vi "Arch_screen_patch_v2.0.vi"() -> ()   [LabVIEW 2012]
uses:
  <vilib>/DAQmx/write.llb/DAQmx Write (Analog DBL 1Chan 1Samp).vi
  <vilib>/DAQmx/create/channels.llb/DAQmx Create Channel (AO-Voltage-Basic).vi
  <vilib>/DAQmx/miscellaneous.llb/DAQmx Fill In Error Info.vi
panel:
  out "ROI cursor":T1={"x offset"=480, "y offset"=456, "x width"=68, "y width"=76} {"x offset" min=1 max=512 step=1; "y offset" min=1 max=512 step=1; "x width" min=1 max=512 step=1; "y width" min=1 max=512 step=1}
  out "Abs V camera":digitalwaveform(waveform)={"t0"=timestamp(0 s since 1904-01-01), "dt"=0.0, "Y"={"transitions"=[], "data"=[]}, "error"={"status"=FALSE, "code"=37421928, "source"=""}}
  out "Abs V lasers":digitalwaveform[](array[waveform])
  out "Abs V DO":digitalwaveform[](array[waveform])
  out "Abs V AO":waveform(dbl)
  out "laser boolean array abs V":bool[](array[boolean])
  out "Previous Bin":u16(ring)=2 caption="Cursor Bin" items=["1x1"=1, "2x2"=2, "4x4"=4]
  in  "Tab":T2(tab)=enum."Acquire"
  in  "Camera trigger":tag="Dev1/port0/line0"
  in  "AOTF info":T3={"AOTF calibration curve path"=path "C:/Peng/LabVIEW codes/Arch_screen_NW348/2013-04-27_AOTF_efficiency", "VISA resource name"="COM8"}
  out "Waveform generated":bool
  in  "Load Mem_AbsV waveform":bool
  in  "Cam frame rate (Hz)\nAbs V":dbl=200.0 format="%0.2p"
  out "# cam. \nframes AbsV":u32=50000
  out "Tot time \nAbs V (s)":dbl=50000.0
  out "# cam. \nframes Mem":u32=50000
  out "Tot time \nMem (s)":dbl=50000.0
  in  "Cam frame rate (Hz)\nMem":dbl=200.0 format="%0.2p"
  out "sample num AbsV":i32
  out "Sample num mem":i32
  out "Model":string="-"
  out "Initialize?":bool
  out "y pixels":i32
  out "x pixels":i32
  out "Bits per Channel":i32
  out "Camera ID":string="-"
  in  "Abs V Waveform txt file":path=path "C:/Peng/LabVIEW codes/Arch_screen_NW348/waveforms/03_waveforms.txt"
  in  "Memory Waveform txt file":path=path "C:/Peng/LabVIEW codes/Arch_screen_NW348/waveforms/03_waveforms.txt"
  in  "stop program":bool
  in  "External":dbl(ring)=10.0 caption="Cursor Bin" items=["div10"=10.0, "div50"=50.0]
  in  "Probe Gain":bool caption="Cursor Bin"
  in  "Gain":dbl(knob)=10.0 scale=1.0..100.0
  in  "Shutter lines":T4={"shutter 640nm"="Dev1/port0/line2", "shutter 594nm"="Dev1/port0/line3", "shutter 561nm"="Dev1/port0/line4", "shutter 532nm"="Dev1/port0/line5", "shutter 488nm"="Dev1/port0/line6", "shutter Dragon"="Dev1/port0/line7", "shutter Global"="Dev1/port0/line13"}
  in  "AOTF digital lines":T5={"AOTF 640nm"="Dev1/port0/line8", "AOTF 594nm"="Dev1/port0/line9", "AOTF 561nm"="Dev1/port0/line10", "AOTF 532nm"="Dev1/port0/line11", "AOTF 488nm"="Dev1/port0/line12", "AOTF weak 488nm"="Dev1/port0/line14"}
  in  "AI ports":T6={"AI scaled output"="Dev1/ai0", "AI V_m"="Dev1/ai1", "photodiode"="Dev1/ai2"}
  in  "AO ports":T7={"AO A-M External"="Dev1/ao0", "White LED"="Dev1/ao1", "447nm laser"="Dev1/ao2"}
  in  "DAQ sampling rate":dbl=10000.0 format="%0.0f"
  in  "DI camera fire":tag="Dev1/port0/line1"
  in  "Simultaneous":bool
  out "# output\nsamples L":u32=12500
  out "Laser Pump Waveform":waveform(dbl)[](graph)=[{"t0"=timestamp(0 s since 1904-01-01), "dt"=0.0001, "Y"=array[12500 elements]}, {"t0"=timestamp(0 s since 1904-01-01), "dt"=0.0001, "Y"=array[12500 elements]}]
  out "Square Waveform":waveform(dbl)[](graph)=[{"t0"=timestamp(0 s since 1904-01-01), "dt"=0.0001, "Y"=array[60000 elements]}, {"t0"=timestamp(0 s since 1904-01-01), "dt"=0.0001, "Y"=array[60000 elements]}]
  out "Triangle Waveform":waveform(dbl)[](graph)=[{"t0"=timestamp(0 s since 1904-01-01), "dt"=0.0001, "Y"=array[120000 elements]}, {"t0"=timestamp(0 s since 1904-01-01), "dt"=0.0001, "Y"=array[120000 elements]}]
  out "memory camera":digitalwaveform(waveform)={"t0"=timestamp(0 s since 1904-01-01), "dt"=0.0, "Y"={"transitions"=[], "data"=[]}, "error"={"status"=FALSE, "code"=37421928, "source"=""}}
  out "Memory DO":digitalwaveform[](array[waveform])
  out "Memory AO":waveform(dbl)
  out "Memory lasers":digitalwaveform[](array[waveform])
  out "laser boolean array memory":bool[](array[boolean])
  in  "Lasers to use":bool[](array[boolean])=[TRUE, FALSE, FALSE, FALSE, FALSE]
  in  "Square setting":T8={"Baseline Sq (mV)"=-70.0, "Stepsize Sq (mV)"=100.0, "Duty cycle (%)"=50.0, "Voltage freq. (Hz)"=5.0, "# cycles per color"=30, "Frame rate (Hz)"=1000.0, "# spect. cycles"=1, "Clamp mode"=FALSE, "Baseline Sq (pA)"=0.0, "Stepsize Sq (pA)"=500.0} caption="Square wave settings" {"Stepsize Sq (pA)" format="%0.2p"; "Baseline Sq (pA)" format="%0.2p"; "Frame rate (Hz)" format="%0.0f"; "Voltage freq. (Hz)" format="%0.2p"; "Duty cycle (%)" format="%0.2f"; "Stepsize Sq (mV)" format="%0.2p"; "Baseline Sq (mV)" format="%0.2p"}
  out "Square info":cluster{"# frames":u32, "# output\nsamples":u32}={"# frames"=6000, "# output\nsamples"=60000}
  in  "Triangle setting":T9={"# cycles per color"=3, "Voltage freq. (Hz)"=0.1, "Amplitude Tri (V)"=0.1, "# spect. cycles"=1, "Frame rate (Hz)"=10.0} caption="Triangle wave settings" {"Frame rate (Hz)" format="%0.2p"; "Amplitude Tri (V)" format="%0.2p"; "Voltage freq. (Hz)" format="%0.3f"}
  out "Triangle info":T10={"# frames"=120, "# output\nsamples"=120000, "voltage slope\n(mV/sec)"=100.0}
  in  "Pump setting":T11={"Duty cycle (%)"=50.0, "# spect. cycles"=1, "# cycles per color"=5, "Laser freq. (Hz)"=4.0, "Holding (mV)"=-70.0} caption="Laser pump settings" {"Holding (mV)" format="%0.2p"; "Laser freq. (Hz)" format="%0.2p"; "Duty cycle (%)" format="%0.2f"}
  out "Elapsed time (sec)":dbl=100.0 min=1.0 max=5000.0 step=1.0
  in  "Total time (sec)":dbl=100.0 min=1.0 max=5000.0 step=1.0
  in  "# frames":u32=100 min=1 max=5000 step=1
  in  "Acquire movie":bool
  in  "447 signal":dbl=2.5 caption="447 signal (0-5V)"
  in  "Shutters":bool[](array[boolean])=[FALSE, FALSE, FALSE, FALSE, FALSE, FALSE, FALSE]
  out "laser bool array":bool[](array[boolean])=[TRUE, FALSE, FALSE, FALSE, FALSE] caption="Waveform"
  in  "AOTF efficiency":dbl[](array[numeric])=[1.0, 0.25363829, 0.20220272, 0.020387013, 0.10018123, 0.010868696] caption="AOTF\nefficiency"
  out "simultaneous ind":bool caption="Simultaneous?"
  in  "Dichroic":u16(ring)=2 caption="Cursor Bin" items=["510/20, 640LP"=1, "ZT532/640rpc"=2]
  in  "Emission filter":u16(ring)=3 items=["600/37"=1, "ET575/50"=2, "708/75"=3, "620LP"=4, "ET590/50M"=5, "HQ660LP"=6, "525/30"=7]
  in  "apply dualview":bool
  in  "apply const power":bool
  in  "apply const fluor":bool
  in  "Const fluor.":u16[](array[numeric])=[595, 455, 150, 360, 150, 150]
  in  "Const power":u16[](array[numeric])=[248, 455, 132, 266, 475, 475]
  in  "DualView":u16[](array[numeric])=[1023, 760, 260, 800, 10, 10]
  in  "AOTF amplitude":u16[](array[numeric])=[604, 144, 112, 51, 71, 24] caption="AOTF\namplitude"
  in  "White LED":bool
  out "file size (MB)":dbl[](array[numeric])=[242.25, 4.845]
  out "cam frame\nrate (Hz)":dbl[](array[numeric])=[1000.0, 10.0]
  out "# cam\nframes":i32[](array[numeric])=[6000, 120]
  in  "Previous ROI":bool
  out "Previous ROI":T1={"x offset"=256, "y offset"=256, "x width"=512, "y width"=512} caption="Previous" {"x offset" min=1 max=512 step=1; "y offset" min=1 max=512 step=1; "x width" min=1 max=512 step=1; "y width" min=1 max=512 step=1}
  out "Location indicator":u16[][](graph)
  out "Waveform Graph":cluster{"xo":i32, dbl, "data":dbl[][]}(graph)={"xo"=0, 0.0001, "data"=array3x120000[360000 elements]}
  in  "appended folder name":string
  out "Status":string="Ready"
  in  "SAVE":bool=TRUE
  in  "Start acquisition":bool
  in  "Exposure (msec)":dbl=100.0 min=1.0 max=5000.0 step=1.0
  in  "Live":bool
  in  "Update ROI":bool
  out "ROI":T1={"x offset"=960, "y offset"=912, "x width"=136, "y width"=152} caption="Current" {"x offset" min=1 max=512 step=1; "y offset" min=1 max=512 step=1; "x width" min=1 max=512 step=1; "y width" min=1 max=512 step=1}
  in  "base path":path=path "C:/Peng/Data"
  in  "Notes":string
  out "Image":u16[][](graph)
  out "Error":errorcluster
  out "full path":path=path "C:/Peng/Data/2013-10-16 patch ssFRET rainbow/PZ083 Arch3.77Q-YFP/fov2/20131016at2350_ST_take1 640"
  in  "Snap&Save":bool
  in  "Bin (n x n)":u16(ring)=1 caption="Cursor Bin" items=["1x1"=1, "2x2"=2, "4x4"=4]
  in  "Camera mode":u16(ring) items=["Focus", "Square wave", "Triangle wave", "Memory", "Absolute Voltage"]
  in  "Symmetrical":bool=TRUE
  in  "Define ROI":bool
  out "max frame rate (Hz)":dbl
  in  "ROI selection":u16(ring)=2 items=["Full ROI", "Central quad", "Custom ROI"]
  in  "Measurements":T12={"Square wave"=TRUE, "Triangle wave"=TRUE, "Laser pump"=FALSE, "Memory"=FALSE, "Absolute Voltage"=FALSE}
  in  "White Light\nCurrent (mA)":dbl=100.0
  in  "AOTF\ndigital":bool[](array[boolean])=[FALSE, FALSE, FALSE, FALSE, FALSE, FALSE]
  in  "447nm":bool
  in  "AOTF channels":string[](array[string])=["640nm", "594nm", "561nm", "532nm", "488nm", "488 weak", ""] caption="AOTF\nchannels"
  out "Image info":T13={"max value"=189, "mean"=115, "min value"=72, "Histogram"={"X Values"=[72.585, 73.755, 74.925, 76.095, 77.265, 78.435, 79.605, 80.775, 81.945, 83.115, 84.285, 85.455, 86.625, 87.795, 88.965, 90.135, 91.305, 92.475, 93.645, 94.815, 95.985, 97.155, 98.325, 99.495, 100.665, 101.835, 103.005, 104.175, 105.345, 106.515, 107.685, 108.855, 110.025, 111.195, 112.365, 113.535, 114.705, 115.875, 117.045, 118.215, 119.385, 120.555, 121.725, 122.895, 124.065, 125.235, 126.405, 127.575, 128.745, 129.915, 131.085, 132.255, 133.425, 134.595, 135.765, 136.935, 138.105, 139.275, 140.445, 141.615, 142.785, 143.955, 145.125, 146.295, 147.465, 148.635, 149.805, 150.975, 152.145, 153.315, 154.485, 155.655, 156.825, 157.995, 159.165, 160.335, 161.505, 162.675, 163.845, 165.015, 166.185, 167.355, 168.525, 169.695, 170.865, 172.035, 173.205, 174.375, 175.545, 176.715, 177.885, 179.055, 180.225, 181.395, 182.565, 183.735, 184.905, 186.075, 187.245, 188.415], "Histogram: h(x)"=[1, 0, 0, 0, 0, 0, 0, 0, 0, 0, 0, 0, 1, 0, 2, 0, 0, 3, 1, 2, 8, 6, 23, 82, 113, 84, 265, 249, 411, 1102, 818, 853, 1028, 1082, 1261, 2548, 1184, 1231, 1256, 891, 1045, 1706, 613, 540, 482, 408, 303, 447, 154, 112, 91, 74, 87, 22, 18, 13, 13, 11, 9, 8, 1, 3, 1, 1, 1, 0, 0, 2, 0, 0, 0, 0, 1, 0, 0, 0, 0, 0, 0, 0, 0, 0, 0, 0, 0, 0, 0, 0, 0, 0, 0, 0, 0, 0, 0, 0, 0, 0, 0, 1]}}
  out "Frames Recorded":i32
  in  "Movie name":string
  out "Patch quality":T14={"Ra (Mohm)"=16.150195020321526, "Rm (Mohm)"=1531.699142639844, "Cm (pF)"=12.467883400052433}
  out "Average I-t curve":cluster{"xo":i32, dbl, dbl[]}(graph)={"xo"=0, 5e-05, [2.8707122065427546, 28.25943561367525, 495.34938130700425, 622.4519180333322, 425.26771536879573, 278.1195833345387, 189.11750895359194, 128.51335365854402, 88.53469124393202, 62.11882679632106, 45.13719962647474, 31.418606844285872, 23.429798545455782, 18.90309568623423, 14.687982318872775, 12.446269046932088, 10.239176831097117, 8.34849917972882, 7.35697405512405, 7.089655767322204, 6.89441489534627, 5.943330783548681, 5.999092552412099, 5.674022726333197, 5.807681868962271, 5.388399026472767, 4.8008359874823965, 5.397054290640863, 5.795196415013253, 5.6037857312452894, 3.6420255502292136, 4.2449093465586785, 4.462285821390441, 4.81232655490619, 4.06314881117431, 4.023702683502782, 4.856597758823761, 5.0643240833158805, 3.890043539987264, 4.402693860851977, 3.6188950637578388, 3.8093108632431627, 4.008381925697188, 3.6092449159742417, 4.208447872227028, 3.5275173543206915, 3.7487240188077378, 4.950810771116034, 4.170842165203316, 3.513042131492717, 4.365088153558202, 4.212128714503955, 3.897703919213018, 4.150696331711198, 3.6774921383958934, 3.478421076610598, 3.5812893553166996, 4.423685227161449, 4.491086914876741, 3.9399853523124615, 3.5245326999555786, 3.8015011340435922, 4.4737763887167485, 3.771705153758482, 3.5033919835424494, 3.688982707357445, 3.5072221719058696, 4.210138942235079, 4.480441882017596, 4.22560904889491, 4.265055177230385, 3.4706113488645483, 4.503423019449819, 4.148557213549512, 3.2147836308660427, 4.159202246520172, 3.6495365784348035, 4.560179676020346, 3.9188446343850734, 3.726439066639748, 3.813986586682297, 3.8717381274540426, 3.962120952275759, 3.611085335331802, 3.2735300559554843, 3.6774921393547224, 3.0860989116048767, 3.0957490597233615, 2.9091634491428553, 3.8179661263568017, 2.9687554116458377, 2.950599347172765, 3.1438504516499965, 2.9419440835611486, 3.116044240320801, 3.9556048097735528, 3.793144570341247, 4.41532866466503, 3.820950782063075, 3.8940230795432553, 4.243068928043317, 5.0057270088990995, 4.145025723437888, 4.121049701768749, 4.235408549596437, 3.484241037148812, 3.047647666451965, 3.167826472926228, 2.7938097180689163, 2.6696513744839825, 3.478421077597534, 3.52070251050323, 3.040832823259014, 3.772700038745409, 3.4802614973361625, 4.136221108929308, 3.518712740842017, 3.8967090322741544, 3.8822338110762447, 3.6580424951603736, 4.364938802393973, 4.243765113064731, 4.017733374522697, 5.402575546268753, 4.085135062157726, 4.03220859674942, 3.940830887980181, 4.681353364917516, 3.958141414588577, 3.436985179664323, 3.484091687209613, 3.9937573539364206, 3.3561031534289367, 4.123586307280213, 3.295516308920549, 3.1879723046440365, 3.183147229597545, 3.0042220007778875, 3.5649737132920962, 3.5688039024557785, 3.5504984908457278, 3.1476806401485162, 2.7408832516409616, 2.666816069009991, 2.896677996222178, 3.254528457670239, 3.812295516696531, 3.6208848342587534, 3.091918870269982, 3.752554208494307, 3.347746588573524, 3.1832965805156896, 3.4141533914677353, 3.238063467210657, 3.737233449313549, 3.665156035932181, 2.9043383758197265, 3.847762108077382, 3.295815006546575, 2.8707122061701376, 2.9196591347766976, 2.8918529229379635, 2.763018853441849, 3.248708499972387, 3.147680641571172, 3.753549092093494, 2.93512924113729, 3.1947871478342127, 3.0927644059598642, 3.065803729594899, 3.4484757489316546, 2.8580774051196585, 3.3407823961033065, 3.610090451051438, 3.1666822395681997, 3.8293073449580333, 3.5466683010591322, 2.7725196519836453, 3.63605624228866, 3.151361482411702, 2.771524768119689, 2.86290247786551, 3.5841246596346896, 3.5985998808722592, 3.8351273041809937, 3.628395862475988, 3.1811574620103262, 3.5283628884880756, 3.125395690871513, 3.6274009786868104, 3.5688039016658197, 2.986911473213223, 2.687807437324858, 3.0263576018969873, 3.394703746055811, 3.17449196711015, 3.210107905674445, 3.503391983506148, 3.298500962686518, 3.35426273396358, 2.4937107964587506, 2.899513300969879, 3.0975894787488385, 2.900358837483566, 3.1696668929879364, 3.9274998985711203, 2.991736548293083, 3.528362889331557, 3.269699866124547, 2.8975235321834654, 2.96676564182466, 2.7763498429642675, 3.0686390350921897, 2.911998753926087, 2.7340684091349785, 2.843751530540078, 2.5003762927589874, 3.188967190353448, 3.9468001942839486, 3.1024145537142283, 2.3350807478640707, 2.848576604166416, 3.5160267863942365, 3.121714850915303, 3.171656662784131, 3.0543131617334405, 2.9341343563008473, 2.7024320079126802, 2.4937107978816617, 2.802464981799372, 3.054462510324043, 3.6506808143167673, 2.947764042002109, 2.8668820164989324, 2.5677779799164897, 2.962089916122025, 3.184291464550388, 2.8572318690848606, 3.837266423481291, 2.8736968594072883, 2.4024824360153496, 3.03814686754593, 3.977740410645141, 3.0775929965325073, 3.207421950221236, 3.315115302978166, 3.31511530295825, 3.8286111597263828, 2.863051827098326, 3.188121654027938, 3.123704619874777, 3.7631992403071175, 3.669831761129438, 2.971590715530302, 3.169816241769228, 3.0621228891125574, 3.0062117702383317, 2.723423377103205, 3.5082170572886073, 3.4687709286069697, 2.8196261602637356, 3.13987091299179, 3.3292918268546083, 2.716757881605072, 1.9935459302372251, 2.463765469786085, 3.3590878088139546, 3.911184257035688, 3.7332539110731227, 2.797639907149591, 3.3246161026796726, 3.4938911844625085, 3.4015185907484784, 3.354412083213049, 3.7092778896912812, 3.3544120829400885, 3.366052000028813, 3.3276007561109537, 2.623539752408288, 3.16698093704695, 2.997705855446494, 3.1371849570223636, 3.7412129879546265, 4.116224628425303, 4.409508707303248, 3.9797301797364373, 3.460414363687271, 3.7363879143265177, 4.414333780436046, 3.944114240479511, 4.273014257618848, 4.416323549705721, 4.187456505855945, 4.628874948847732, 4.683641836040581, 3.7478784833258767, 3.4382787628796616, 3.8152801710309263, 3.6613258471654078, 3.6806261429867977, 3.3469010526306815, 3.0198414573901218, 2.993875665257011, 3.321780796754825, 2.9870608222374897, 3.0746083430207944, 2.91781871363435, 3.084258491383432, 2.89185292323233, 3.1563359041780004, 3.2706947511573845, 2.9417947343628525, 2.9494551143010703, 3.3274514068532004, 3.1302207646192888, 3.0561535815057033, 3.217768286208913, 3.6611764974160215, 3.399528820393036, 3.2024475259457126, 3.416839348063967, 2.7417287879202084, 2.97641578879201, 2.504206481875124, 3.1841421158493204, 2.4907261445403774, 2.889863153396935, 2.860067173150541, 2.8773777000467877, 2.9023486067898947, 2.894688228699809, 2.948609578617893, 3.0072066541537397, 3.191802495675408, 2.9524397675590315, 3.0707781532693157, 3.464095204428533, 3.4564348242220446, 2.997705854696192, 3.7651890097952907, 3.2255780142065733, 3.6969417858473683, 3.3237705669123585, 3.314120419459688, 3.486230806482259, 3.331430946298682, 3.4276337295913986, 3.7440482929472614, 3.7979696435108328, 3.6027287708773934, 3.22955755198841, 4.125874776384638, 4.149850797955419, 3.6468506239541543, 2.8467361844359553, 2.8658871325440525, 2.7044217775683115, 2.873696859302152, 3.568953252296793, 2.761029084912285, 3.1418606820151935, 2.7994803282863496, 3.3121306486931745, 2.689797207877824, 2.3523912747867963, 2.7640137377922342, 3.2601990672746926, 2.889863153600081, 2.5735979393854227, 2.3032949986371962, 3.091918868845924, 3.4323094545038373, 3.22259335983235, 3.435144759394521, 2.5947386555681105, 3.4622547838946183, 3.0967439436231663, 3.139025376806457, 3.0072066539772853, 2.97940044288373, 3.2870103937173187, 2.7610290841459486, 3.0476476671698296, 2.304289882517204, 2.3647273798700876, 2.6398553930502735, 3.356401851900153, 2.9908910117041128, 2.925329743873894, 3.4542957075834346, 3.4947367198543153, 2.446454941428994, 3.5658192487300653, 2.9138391755558537, 3.8389574941100566, 3.7177838033712827, 3.544678531437946, 3.1829978825016005, 3.0955997101196484, 3.247564264913362, 3.1388760280089434, 3.679332559840362, 3.2494046854319616, 3.6370511253032505, 3.3214820995739966, 3.672517716343648, 4.857293941831456, 3.5561691003982703, 3.658191842748496, 3.1656873556728815, 3.940830887540439, 4.065834766619217, 3.644711505535287, 3.3619231125444498, 3.2985009618137697, 3.057148466016686, 2.404173508156449, 2.8033105180842313, 2.773514536907434, 3.023522296436222, 3.4957316048223146, 2.9196591337052973, 2.986065937940638, 2.542807073880078, 3.232392856050453, 3.352571662706912, 3.4516097513376107, 3.0477970160338375, 3.115049355662422, 2.934283704766447, 3.759518399715842, 3.9624196517063375, 3.7219126923054717, 3.9950509371056064, 3.9729153359560283, 4.153680985884926, 3.626555443883822, 3.2765147111710906, 3.036157098054292, 3.432309455356358, 2.9842255162885896, 3.4804108463417456, 2.925479092267475, 3.146685756112349, 2.902348606900604, 3.5350283839702943, 4.16402731985239, 3.218763169057505, 3.231099274872322, 3.785036143660749, 3.384058712902455, 3.288850814307387, 3.1898127254077173, 3.9033745278776797, 4.274555977540524, 4.521728431380804, 4.585150581070805, 4.399559856997121, 4.7630809271232755, 4.2226243956178555, 2.9349798917285366, 4.338973012012414, 4.771736190279414, 4.308182146805416, 3.4321601052121467, 2.8917035738099983, 3.295665657435235, 3.7668800804821823, 2.512712397088227, 2.912844290320792, 2.5281825041943975, 2.6197095611842265, 2.7571988944454744, 3.364062229786042, 2.3147855670896695, 2.6465208886570704, 2.4099934668192833, 2.9620899162682424, 2.7495385155727723, 2.6774611023246933, 3.5842740099090826, 3.0043713499751687, 3.252538689160112, 3.4401191834700438, 3.1140544709583997, 3.0035258135825376, 3.079433417004819, 3.702612394956965, 2.4773951555330798, 2.5947386564887838, 2.6321950152318507, 2.294639735716159, 2.3157804521216305, 3.7535490926542154, 3.0005411606781016, 2.8409162258903518, 3.19379226438722, 2.658160805847134, 3.512196596422924, 2.927468861228087, 2.261859101671224, 3.3034753841867235, 2.8341013820615393, 3.1630013988305703, 3.60342495755381, 3.477426192241734, 3.2898456981942843, 2.9128442908621466, 3.401369241617793, 3.573628976358294, 3.1225603852010773, 2.9456249244133543, 3.268704982686596, 3.567809017106723, 3.743749594095346, 3.8504480628980198, 3.967791563569359, 3.5744745123093096, 3.139870911861787, 2.8224614647197415, 2.994571852654043, 3.368737955242065, 3.9053642967118813, 3.480261498043539, 2.683977248557281, 3.46678116027577, 2.641695814748386, 2.98308128423232, 2.3792026019494914, 3.1764817360571387, 3.5466683010450475, 2.645526004637833, 2.536837767028622, 2.2993154608298614, 2.7195931867553873, 3.5158774379119917, 2.8946882284706312, 3.4784210774742435, 2.987906357593042, 2.865737783050705, 3.6245656742740393, 3.2485591498456823, 3.4524552856115296, 3.1273854594221735, 2.8023156334708594, 2.821466581611065, 3.2081181366250093, 3.1398709132404155, 2.873547510373572, 3.1340509546636404, 2.5647933269685517, 2.4725700810232496, 2.713922577437449, 2.818780624340463, 2.6187146776940993, 3.2265728979400663, 3.4208188854942834, 2.6177197929199445, 3.1255450405709353, 2.438943910463403, 2.7793344966062756, 2.853401679581337, 3.437134529569843, 2.6263750563398855, 3.07843853218823, 3.7680243133907907, 3.293825237849658, 2.451429364599895, 2.965074569746934, 2.3120996104243616, 2.584242971314685, 3.443949373008597, 3.6093942653280466, 3.6315298663401596, 3.4459391420360572, 3.3978377490206912, 3.2497033835177067, 3.554627379050176, 3.7075868185832714, 3.789314380023221, 3.575768095001147, 4.030517527845748, 3.121714849339175, 2.749538515642346, 2.6456753531433232, 3.006361118994488, 2.814950435378252, 2.8053002869655455, 3.36689753564434, 3.7082830032657075, 3.4995617944544164, 3.5428381114677605, 3.2936758883194277, 2.6666667208588324, 2.8850380792147243, 2.950449998655362, 3.198467989377199, 3.026357601825418, 3.4053487790464096, 3.0706288035281237, 3.2495540340692437, 2.6283648255190557, 2.8302711934834415, 3.116889776773911, 3.38619783300024, 2.661145459479385, 3.467925394858015, 2.8429059946754496, 3.1342003033215207, 3.486230804944647, 3.0582927000685065, 3.0045206983146993, 2.907323029248498, 3.2545284579489118, 3.3805272222081584, 3.6921167117505993, 3.854726299132579, 3.3247654510691067, 3.447779562494094, 3.679631259611349, 4.746218450194578, 4.339421061074454, 4.103739175267747, 4.683641836330334, 4.4134882443951735, 4.913503763549747, 4.152835451076204, 3.6190444140867015, 4.372052346803122, 5.1491856501831235, 3.9153131443260176, 3.4757351221100636, 3.24970338400919, 3.0574471640486154, 3.206427065844133, 3.248708498890782, 3.0514778581265514, 3.4284792667479267, 3.0303371412116573, 2.5043558303503772, 2.726557378535541, 2.8284307716438994, 3.313971068918673, 2.8648922478872128, 2.671641143428947, 3.408184084420307, 3.539007923279625, 3.0100419593876726, 3.4158444623486224, 3.377393217997829, 3.211102789808683, 3.4524552870204253, 2.7542142413392883, 3.211102790653623, 2.5398224205947897, 2.384027676348172, 2.5657882114277455, 2.8455919514018952, 3.5861144301665715, 3.0802789515555187, 2.767694579085781, 2.77450942248423, 2.4580948599368115, 2.523506778234475, 2.876382815828854, 3.373563029421537, 3.4188291166461595, 3.6293907493728845, 2.890012501790204, 2.988055707253936, 3.385352295752182, 3.368041768339701, 3.866216868530548, 3.200607108116509, 3.393012674601122, 2.8034598668118655, 3.5007060284466416, 2.60339391993005, 3.668986226450739, 3.228562666862683, 3.9565996938771066, 3.850746761940187, 4.2287430548969756, 2.7408832532462495, 3.0198414568495835, 4.234563013462294, 3.437283877794516, 3.1390253787582423, 3.9757506422853788, 3.502695797235847, 2.8159453195793214, 2.8900125020017096, 3.2428885397123173, 3.10256390149142, 2.280313860930628, 2.5744434752355665, 2.6821368271173562, 2.4639148177307795, 2.448444711253609, 2.8648922468221034, 2.2147525936043913, 2.6994473551363494, 2.839921341475432, 3.0379975195405096, 2.7696843479831807, 2.1388449909872778, 2.985220402980663, 2.5794178975305786, 2.718747651289582, 2.811120245658247, 2.5351466946471115, 2.864892247210859, 3.016856802430847, 3.1515108306108623, 3.5746238617115864, 2.888868269406041, 3.5756187454741997, 3.0360077498616493, 3.1014196684774022, 2.710937923563189, 3.005216885350583, 3.3053158055183807, 3.0235222964606057, 2.9504499984049404, 2.7888352949960984, 3.9438155425655963, 3.4774261920309493, 2.679152174184789, 4.28137082148243, 3.675502369283701, 2.8820534255943944, 3.20528283120111, 3.7697153849204414, 3.949486150704954, 4.3611086129347605, 3.639886430852413, 3.4764313073827946, 3.894719265053249, 3.6350613566469847, 3.88407423119677, 3.8581084417725395, 3.8321426507056975, 4.618776752028438, 3.8110019335047043, 3.282185318935994, 3.712958728979012, 2.9879063575086664, 3.4110193886856375, 2.911003869845291, 3.031182675747701, 3.4764313075037316, 3.9947522383951863, 2.5704639368512936, 2.4349643728163146, 2.7235727253934363, 2.748543631905971, 2.691786975859794, 2.587078276268855, 2.852556142985496, 3.2189125190863614, 3.1842914652289918, 3.345906168799568, 3.2477136148729815, 3.514186366051607, 4.052802478129551, 4.437464266407563, 4.529687511680404, 4.226753285254196, 4.372897880721317, 3.7998100632476666, 3.600739001153996, 3.771854504593163, 2.9947212021110223, 2.8053002867598664, 2.608218993307086, 3.3525716618591686, 3.115894891724995, 2.86772755159027, 2.9782562090090265, 3.8639283997813365, 3.4446455587897358, 2.8512625610801563, 3.353267849250194, 4.176512772927705, 3.7812059531741755, 3.9013847589177035, 4.373594065532543, 3.949486151111848, 3.974457057236737, 4.0398689768775835, 3.9802770156724288, 3.9255101291466334, 3.9764468254645498, 4.68617843862758, 3.6580424953189214, 4.039868976500649, 4.006242805841156, 3.4581258960137555, 3.787025912602684, 3.7409142884921494, 3.7735455738841948, 3.3446125845637, 3.0609786553161276, 2.948460229833577, 2.5042064817417504, 2.4522749004642965, 3.4967264886104665, 2.6350303198045713, 2.611054297362029, 3.0985843644453364, 2.780329379754096, 2.8668820158082453, 2.686116364802426, 2.7879897604189163, 3.1198744294060066, 3.4602650148195875, 3.1198744302534345, 3.0303371409589688, 2.8111202455677153, 2.3562214651060356, 2.4734156180231146, 3.368887304693373, 3.0572978153935395, 2.503360946022986, 2.5351466953206456, 3.0621228900233657, 3.3419266298632486, 3.225578013197459, 2.8379315726950907, 2.665821185242384, 2.508186019508689, 3.4977213737469155, 3.0687883843172283, 2.581258318084501, 2.58409362302537, 3.38987867230673, 3.777525112664155, 2.829276308406159, 3.261044603319716, 2.6859670167409626, 3.215778515613859, 2.9474653449395984, 2.658011457719395, 2.926324628195077, 3.5014022140214114, 3.5754693965876014, 3.1070902795925472, 2.9965616209151382, 3.3965441663368208, 4.141891718396798, 3.4619560857926674, 3.575469395696376, 3.5774591653139067, 3.3311322481742125, 3.6100904510630714, 3.026357601091023, 3.272535171525131, 3.472601119124259, 2.949455113859931, 3.3812234088615956, 3.052323392411207, 3.3129761847539054, 3.796676059896518, 2.941794734235092, 2.955275071979059, 2.4243193404922048, 2.6148844879098574, 3.16782647239356, 2.9840761679593046, 3.1167404265729095, 3.0955997112309848, 3.4716062338254376, 3.2533842232105825, 2.8638973626515902, 2.586928927806612, 3.0446630141286297, 3.13703560731219, 3.1195757326206524, 2.623390403040666, 2.733073524383954, 2.7725196521279116, 3.017702338984356, 3.2841750888594357, 2.6235397516903234, 2.716757882733719, 3.258209297283213, 3.9814212498305848, 2.631200130229006, 3.421813770532127, 2.5975739611783095, 2.6495055416174407, 2.611054298691691, 2.5494725690420856, 3.1217148501690337, 2.2869793561090592, 3.0592875841345686, 3.0448123623561334, 2.9840761691742683, 2.288819777102465, 2.490875492496891, 3.5593031041673315, 2.862056942735918, 2.8918529226227268, 2.664975648506261, 2.955424421264373, 3.8334362334256666, 3.4294741500522, 2.6514953116853435, 2.860216521845456, 4.218247370470854, 3.5036906814591484, 3.640185130021633, 3.3324258308247305, 4.042157444754421, 3.0313320249506344, 3.203591760530328, 3.436288993026063, 2.932293935559244, 2.892847807416193, 3.788170146544091, 2.8630518259343334, 3.1332054181667934, 3.061128003867776, 2.7764991900913527, 3.0148670338601113, 2.548477684353669, 2.636870741124723, 3.3311322484611146, 3.3937088609443578, 3.098435015344185, 3.1080851631835054, 2.976415788512079, 2.9234893237889383, 2.7032775441012156, 3.4419596025018433, 3.0293422560221486, 3.064958193556626, 3.1024145539957444, 3.46892027751956, 3.4574297101470086, 3.1295245777958085, 3.183296579986558, 3.578603400360894, 3.3083004603221497, 2.832260962956884, 4.264209646646693, 3.4247984244725873, 3.316110186732325, 3.2448783095798217, 3.755538862538854, 3.1122140510041194, 3.991220748852429, 3.8873575852520257, 3.7806591160532506, 4.094089027845379, 3.710422123592654, 3.606558959780672, 3.511351060790711, 4.170145978560038, 3.947944430238941, 3.957594578530026, 3.8903422382094317, 4.450944603513299, 3.8257758561187742, 3.948939314615614, 3.9046681119328817, 3.2651734904991696, 2.73620752675853, 3.6872916378687823, 3.6122295709539602, 3.420818886165599, 3.208267486285765, 3.021681876440441, 3.2851699733153876, 2.9024979548745153, 3.0669479632632024, 2.1821213083040876, 3.513042131760244, 3.3427721661924266, 3.44862509684586, 3.0764487625964145, 2.593594423314543, 3.5947696931958446, 3.5726340914925183, 3.3043209209310733, 2.9601001454474893, 2.820621044091441, 2.967760525716685, 2.8407668776967885, 2.6811419432465633, 2.906178796291823, 2.841761761878927, 3.197622453114008, 2.40999346672357, 2.5657882121174533, 3.434149874742689, 2.9725856003173283, 3.100424785159968, 2.9601001465206704, 2.25036853271538]}
  out "Scaled output":cluster{"xo":i32, dbl, "data":dbl[][]}(graph)={"xo"=0, 5e-05, "data"=array2x40000[80000 elements]}
  in  "Test patch":bool
  in  "Patch tuning param":T15={"Amplitude (mV)"=5.0, "Number of repeats"=20, "Sampling rate"=20000.0, "Wave Freq. (Hz)"=10.0}
  in  "Save patch param":bool
  # "External Memory and Absolute Voltage waveform settings"
  # "High"
  # "Low"
  # "red"
  # "orange"
  # "yellow"
  # "To image with 447 nm laser, choose blue laser here to generate voltage waveform, \nbut TURN OFF blue laser in Acquire page and TURN ON 447 nm laser"
  # "green"
  # "blue"
  # "Voltage"
  # "Current"
  # "Camera settings"
  # "Focus mode settings"
  # "ROI control"
  # "square"
  # "triangle"
  # "mem"
  # "Abs V"
  # "Laser settings"
  # "640nm"
  # "594nm"
  # "561nm"
  # "532nm"
  # "488nm"
  # "Dragon"
  # "Global"
  # "V"
  # "File settings"
  # "Lasers: \n1) Expansion\n2) Shutters\n3) Waveform\n4) White LED off\n5) Em. filter\n\nPatch:\n1) Vclamp\n2) Vhold off"
  # "square"
  # "triangle"
  # "mem"
  # "AbsV"
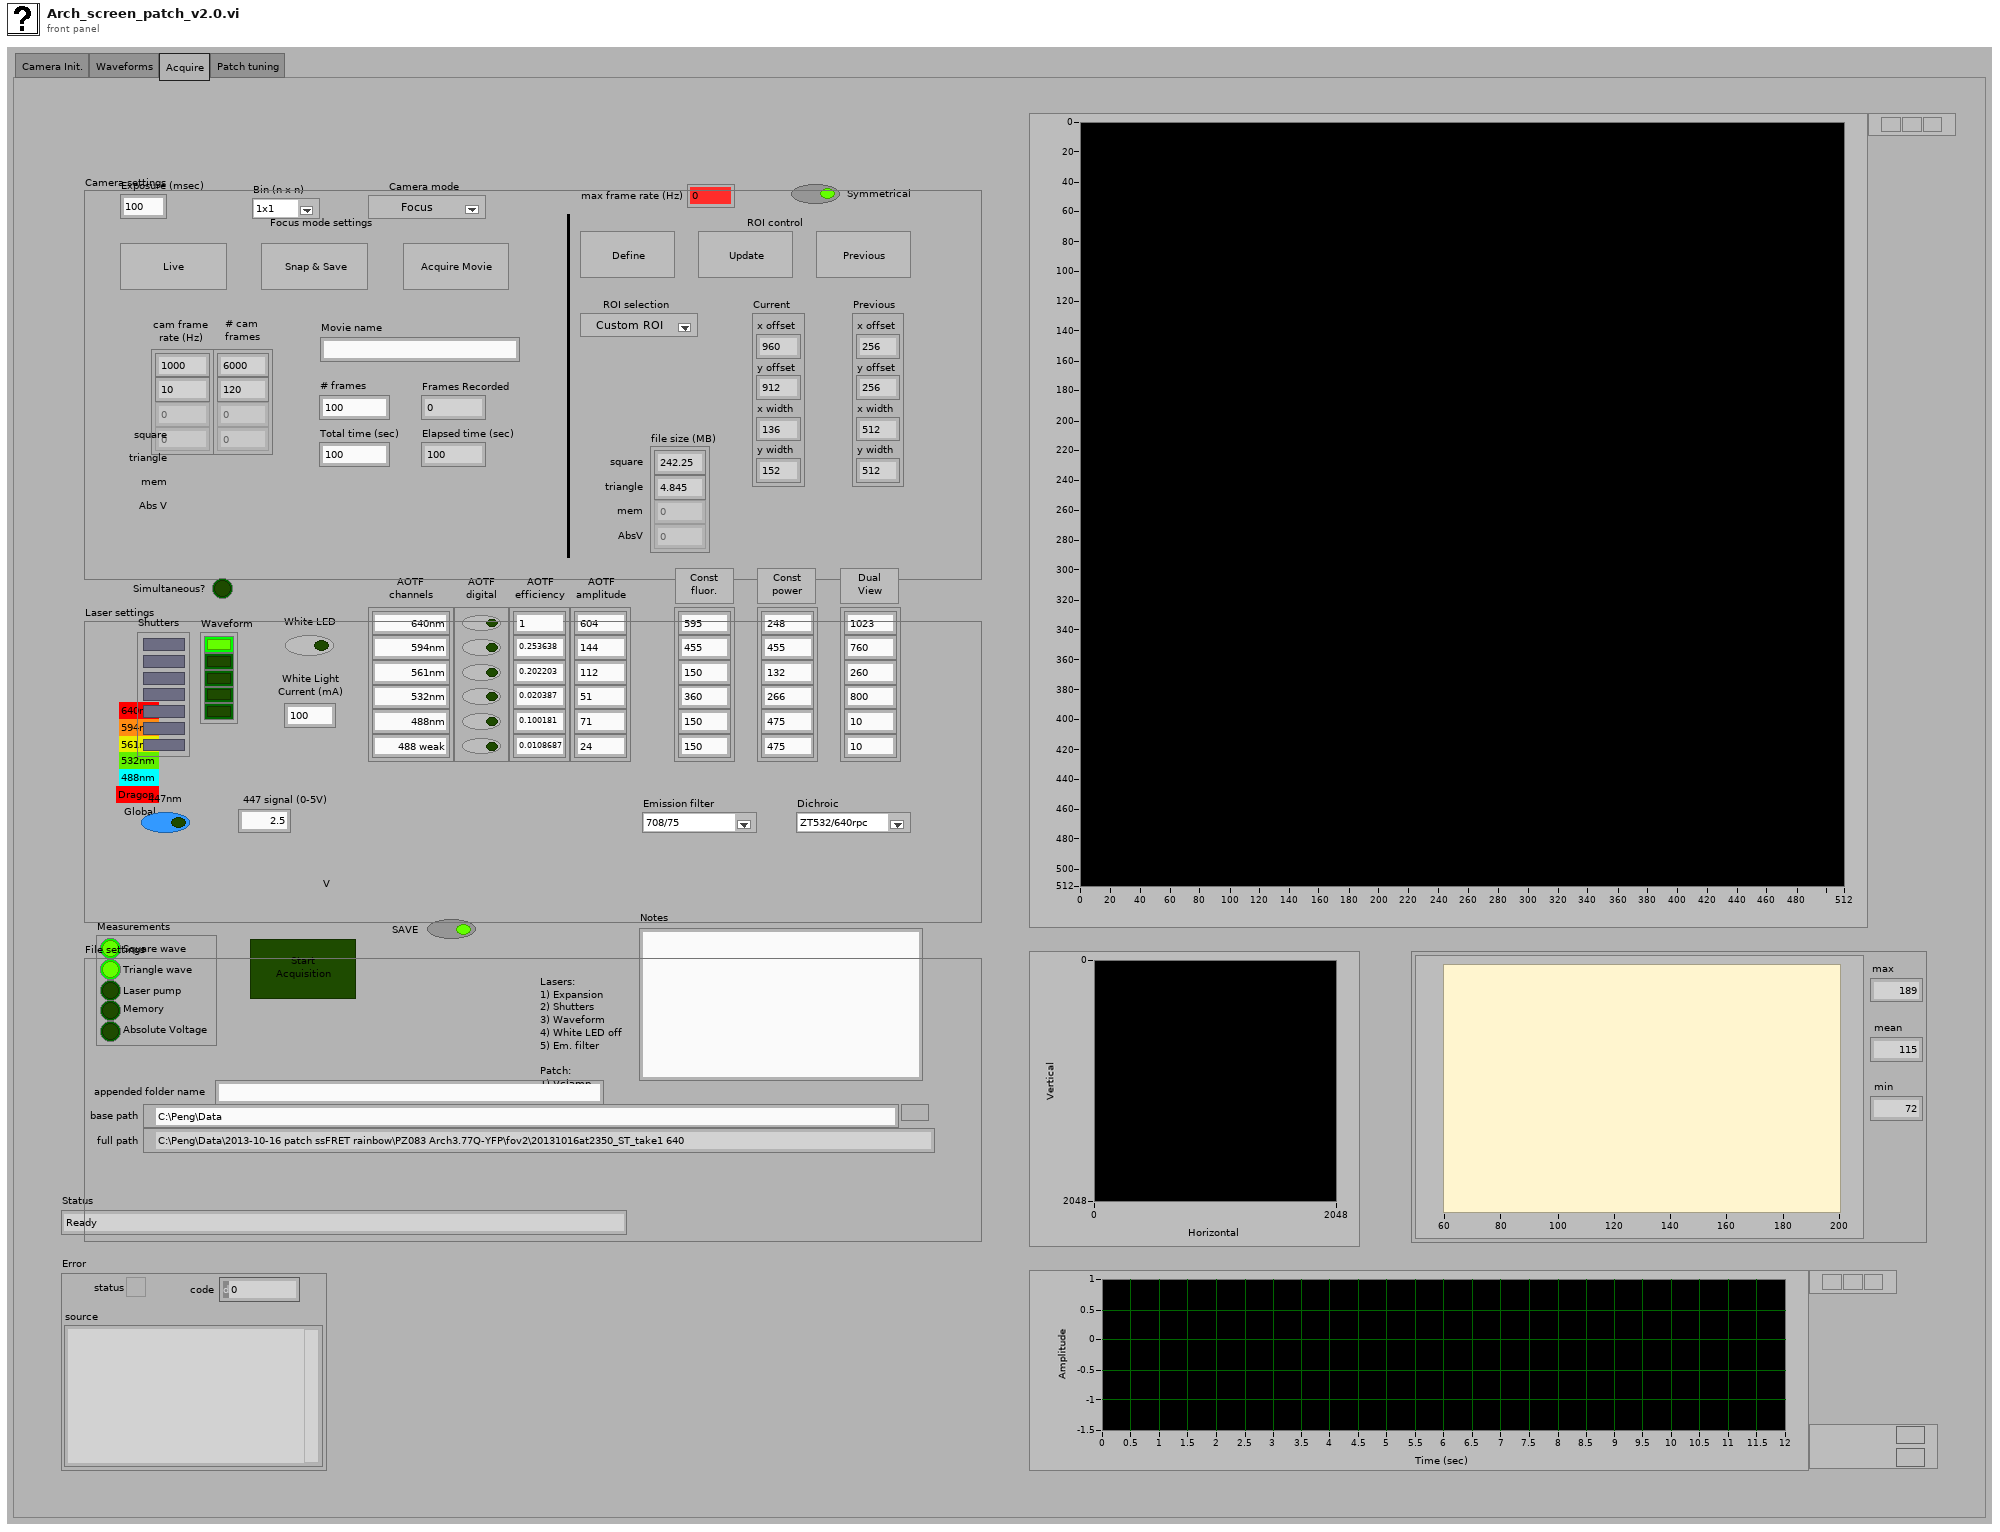
[diagram p1: front panel]
types:
  T1 = cluster{"x offset":i32, "y offset":i32, "x width":i32, "y width":i32}
  T2 = enum32{"Camera Init.", "Waveforms", "Acquire", "Patch tuning"}
  T3 = cluster{"AOTF calibration curve path":path, "VISA resource name":refnum<visa-resource-name>}
  T4 = cluster{"shutter 640nm":tag, "shutter 594nm":tag, "shutter 561nm":tag, "shutter 532nm":tag, "shutter 488nm":tag, "shutter Dragon":tag, "shutter Global":tag}
  T5 = cluster{"AOTF 640nm":tag, "AOTF 594nm":tag, "AOTF 561nm":tag, "AOTF 532nm":tag, "AOTF 488nm":tag, "AOTF weak 488nm":tag}
  T6 = cluster{"AI scaled output":tag, "AI V_m":tag, "photodiode":tag}
  T7 = cluster{"AO A-M External":tag, "White LED":tag, "447nm laser":tag}
  T8 = cluster{"Baseline Sq (mV)":dbl, "Stepsize Sq (mV)":dbl, "Duty cycle (%)":dbl, "Voltage freq. (Hz)":dbl, "# cycles per color":u32, "Frame rate (Hz)":dbl, "# spect. cycles":u32, "Clamp mode":bool, "Baseline Sq (pA)":dbl, "Stepsize Sq (pA)":dbl}
  T9 = cluster{"# cycles per color":u32, "Voltage freq. (Hz)":dbl, "Amplitude Tri (V)":dbl, "# spect. cycles":u32, "Frame rate (Hz)":dbl}
  T10 = cluster{"# frames":u32, "# output\nsamples":u32, "voltage slope\n(mV/sec)":dbl}
  T11 = cluster{"Duty cycle (%)":dbl, "# spect. cycles":u32, "# cycles per color":u32, "Laser freq. (Hz)":dbl, "Holding (mV)":dbl}
  T12 = cluster{"Square wave":bool, "Triangle wave":bool, "Laser pump":bool, "Memory":bool, "Absolute Voltage":bool}
  T13 = cluster{"max value":u16, "mean":i16, "min value":u16, "Histogram":cluster{"X Values":dbl[], "Histogram: h(x)":i32[]}}
  T14 = cluster{"Ra (Mohm)":dbl, "Rm (Mohm)":dbl, "Cm (pF)":dbl}
  T15 = cluster{"Amplitude (mV)":dbl, "Number of repeats":i32, "Sampling rate":dbl, "Wave Freq. (Hz)":dbl}
  T16 = cluster{"width":u32, "height":u32, "datatype":u32}
  T17 = enum8{"Enabled", "Disabled", "Disabled and Grayed Out"}
  T18 = cluster{"# cam. frames":u32, "# output\nsamples":u32}
  T19 = cluster{"Value":i32, "Minimum":i32, "Maximum":i32, "Increment":i32}
  T20 = cluster{"# cam. frame":u32, "# output\nsamples":u32, "voltage slope\n(mV/sec)":dbl}
  T21 = cluster{"X min":dbl, "Y min":dbl, "X max":dbl, "Y max":dbl}
  T22 = cluster{"max value":u16, "mean":i16, "min value":u16, "Image histogram":cluster{"X Values":dbl[], "Histogram: h(x)":i32[]}}
  T23 = cluster{"Cursor.Cursor X":dbl, "Cursor.Cursor Y":dbl, "Cursor.Cursor X":dbl, "Cursor.Cursor Y":dbl}
  T24 = cluster{"Cursor1. X":dbl, "Cursor1. Y":dbl, "Cursor2. X":dbl, "Cursor2. Y":dbl}
  T25 = cluster{"x offset":dbl, "y offset":dbl, "x width":dbl, "y width":dbl}
  T26 = typedef "LVPointDoubleTypeDef.ctl" = cluster{"Cursor X":dbl, "Cursor Y":dbl}
  T27 = cluster{"XScale.Minimum":dbl, "YScale.Minimum":dbl, "XScale.Maximum":dbl, "YScale.Maximum":dbl}
  T28 = cluster{"Cursor.Cursor Position":T26, "Cursor.Cursor Position":T26}
  T29 = cluster{"Cursor1.Position":T26, "Cursor2.Position":T26}
  T30 = cluster{"Active Cursor":u32, "Active Cursor":u32, dbl, dbl}
  T31 = cluster{"ROI":cluster{"x offset":i32, "y offset":i32, "x width":i32, "y width":i32}, "Exposure (msec)":dbl, i32}
  T32 = cluster{"Voltage freq. (Hz)":dbl, "# cycles per color":u32, "# spect. cycles":u32}
  T33 = cluster{"Laser freq. (Hz)":dbl, "# cycles per color":u32, "# spect. cycles":u32}
  T34 = cluster{"cam frame\nrate (Hz)":dbl[], "# cam\nframes":i32[], "ROI":cluster{"x offset":i32, "y offset":i32, "x width":i32, "y width":i32}}
  T35 = cluster{cluster{"Voltage freq. (Hz)":dbl, "# cycles per color":u32, "# spect. cycles":u32}, cluster{"Voltage freq. (Hz)":dbl, "# cycles per color":u32, "# spect. cycles":u32}, cluster{"Laser freq. (Hz)":dbl, "# cycles per color":u32, "# spect. cycles":u32}, "DAQ sampling rate":dbl}
  T36 = cluster{"Measurements":cluster{"Square wave":bool, "Triangle wave":bool, "Laser pump":bool, "Memory":bool, "Absolute Voltage":bool}, "laser bool array":bool[], "Simultaneous":bool, "AOTF efficiency":dbl[]}
  T37 = cluster{"ROI":cluster{"x offset":i32, "y offset":i32, "x width":i32, "y width":i32}, dbl, i32}
  T38 = cluster{"DI camera fire":tag, tag[], "AO A-M External":tag, "AI ports":tag[]}
  T39 = cluster{"Ra (Mohm)":string, "Rm (Mohm)":string, "Cm (pF)":string}
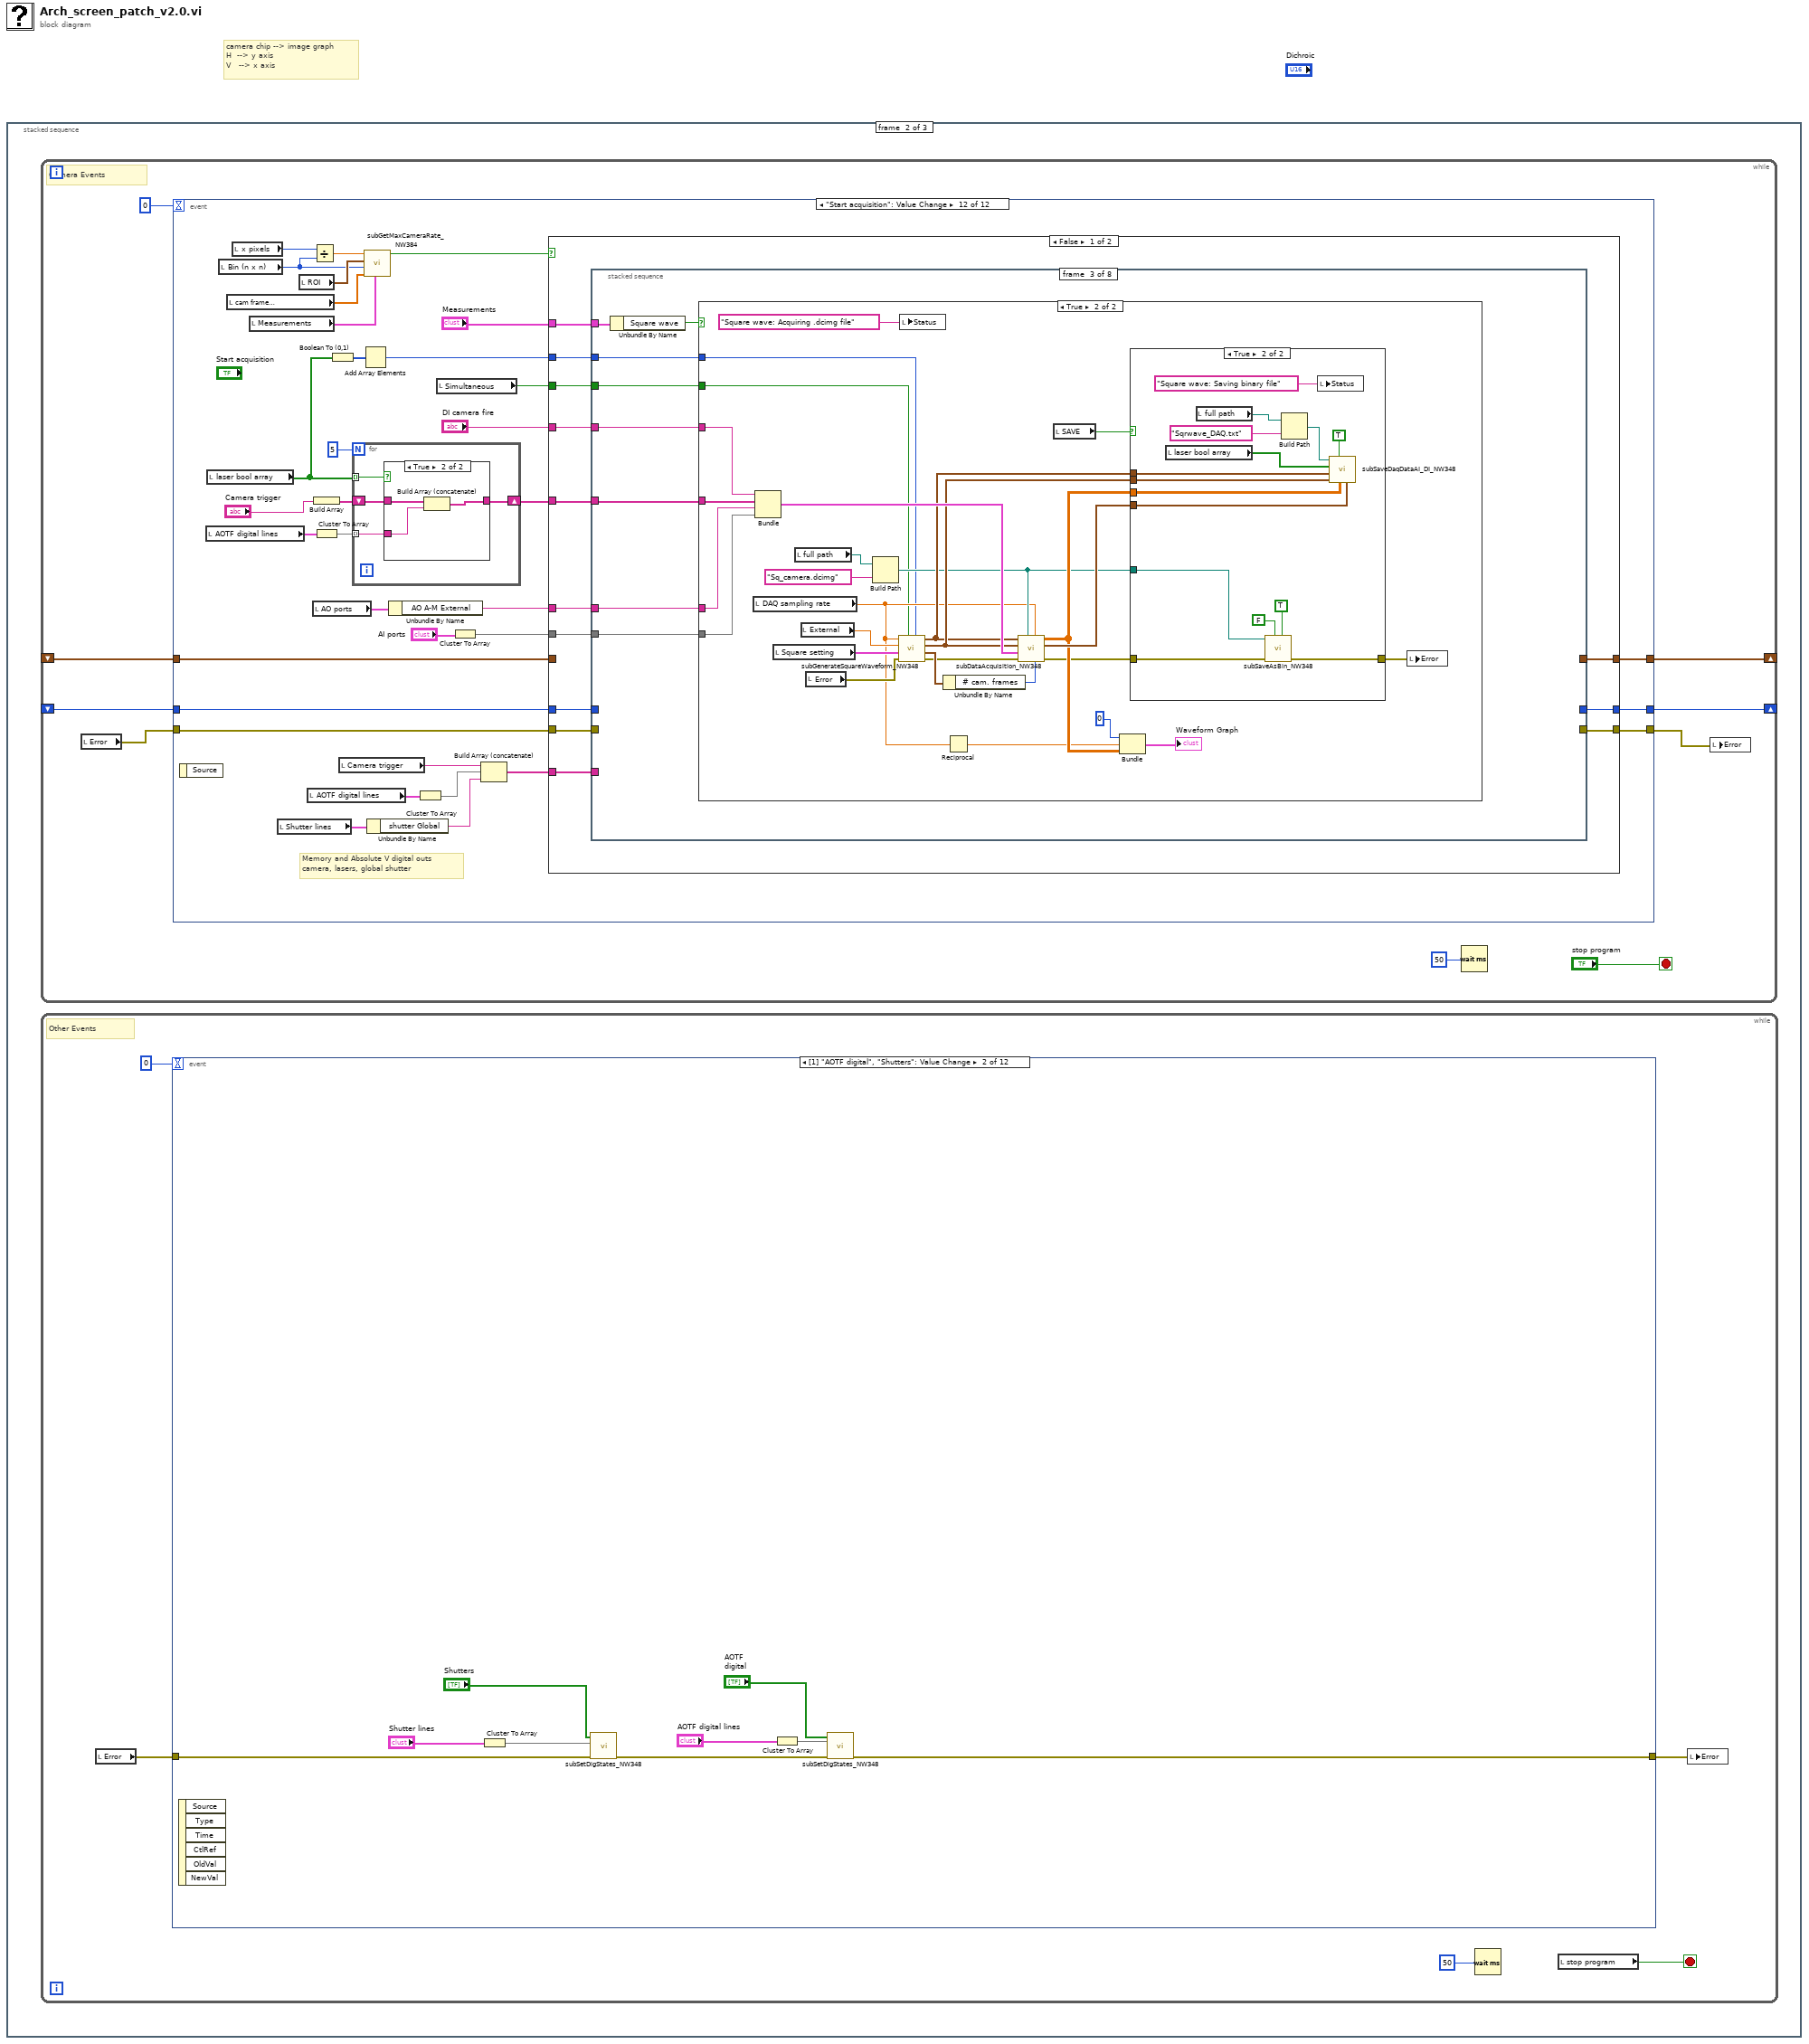
[diagram p0: block diagram]
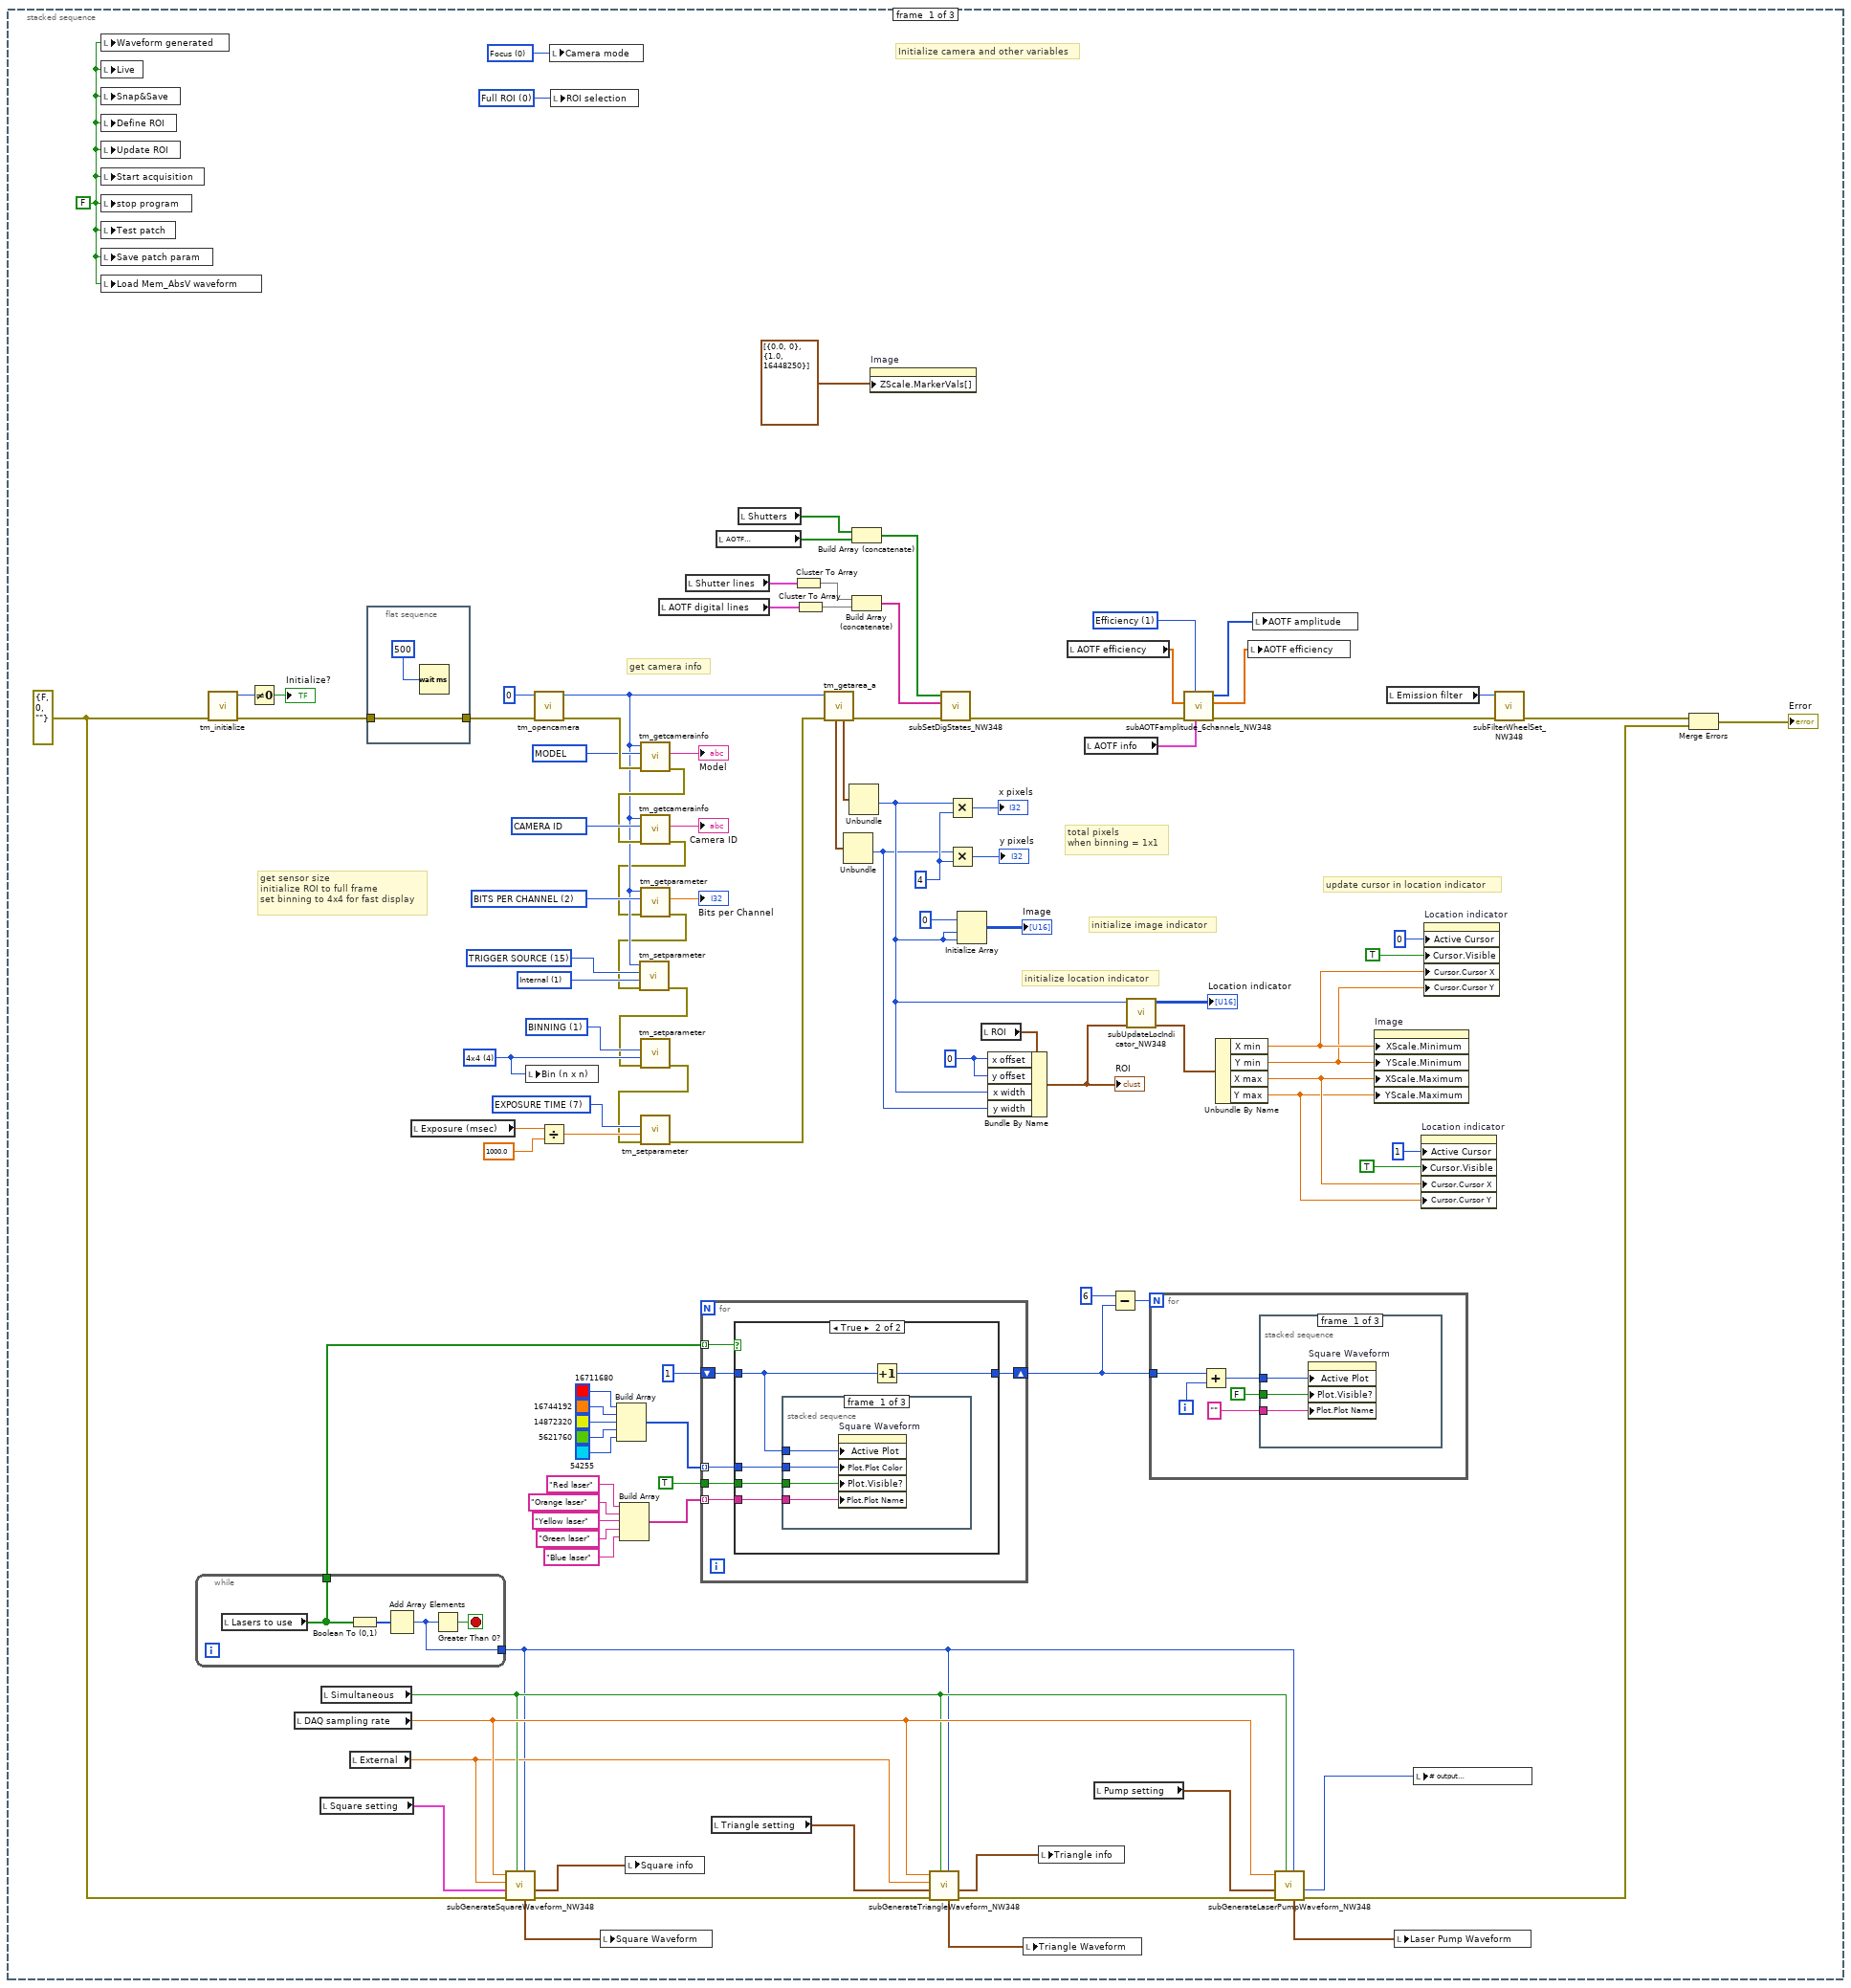
[diagram p2: hidden frame]
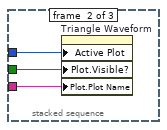
[diagram p3: hidden frame]
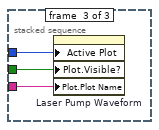
[diagram p4: hidden frame]
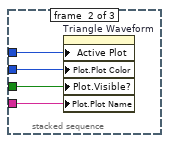
[diagram p6: hidden frame]
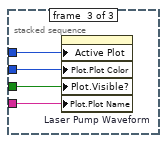
[diagram p7: hidden frame]
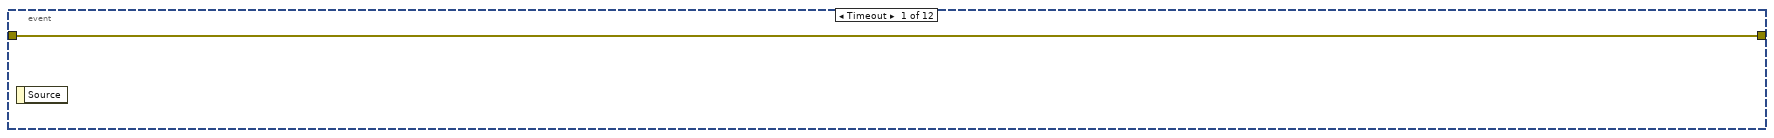
[diagram p8: hidden frame]
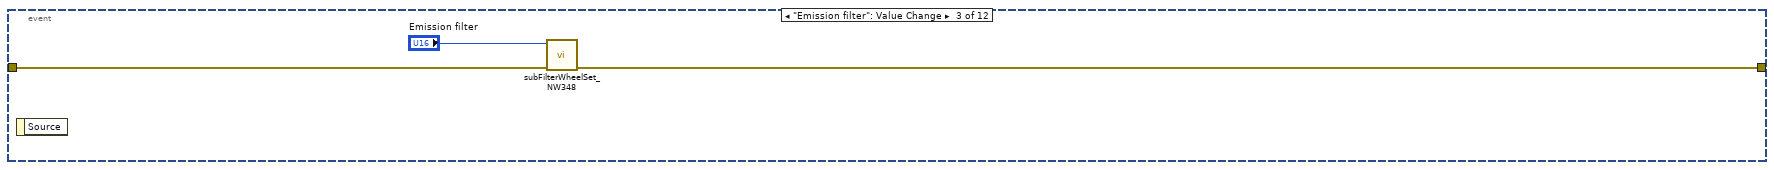
[diagram p9: hidden frame]
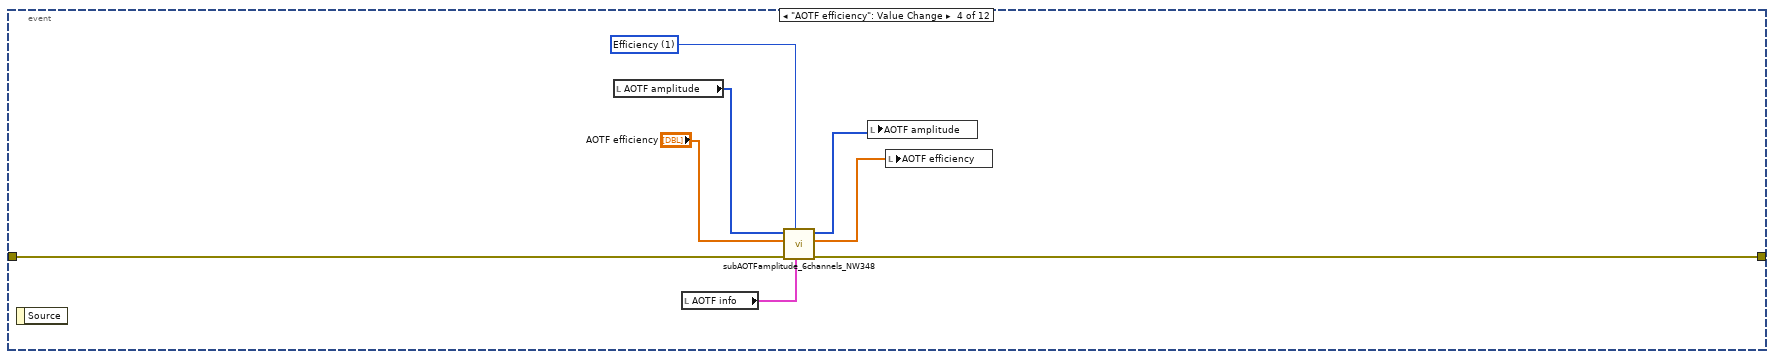
[diagram p10: hidden frame]
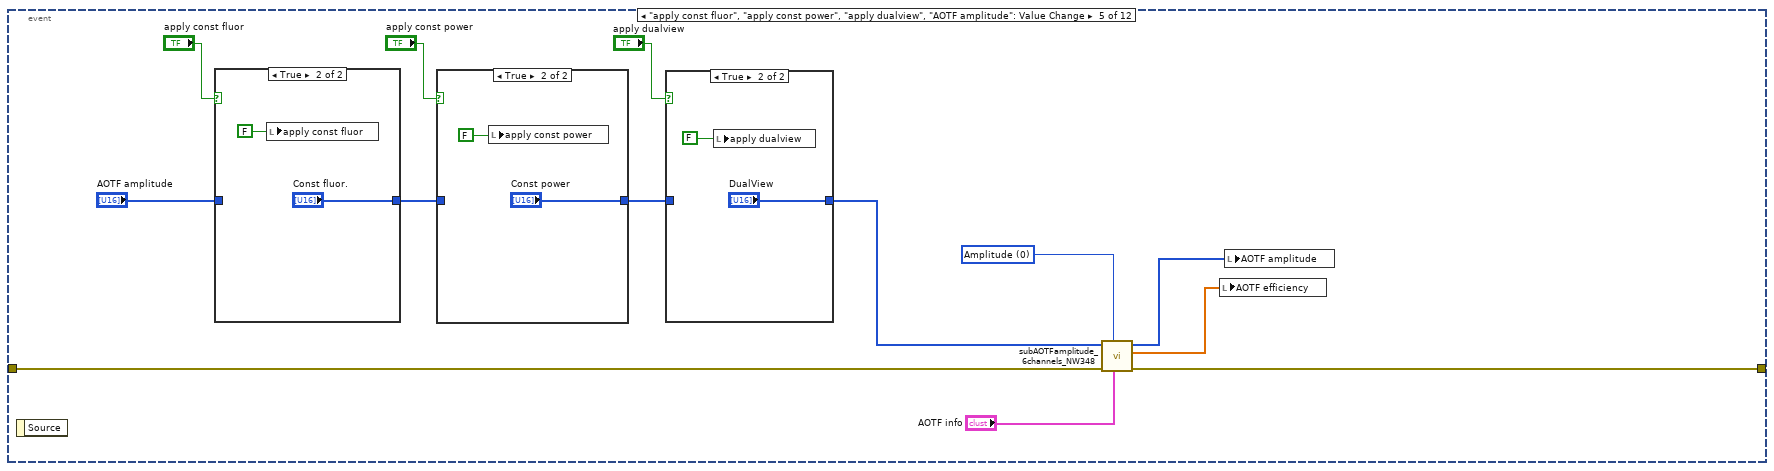
[diagram p11: hidden frame]
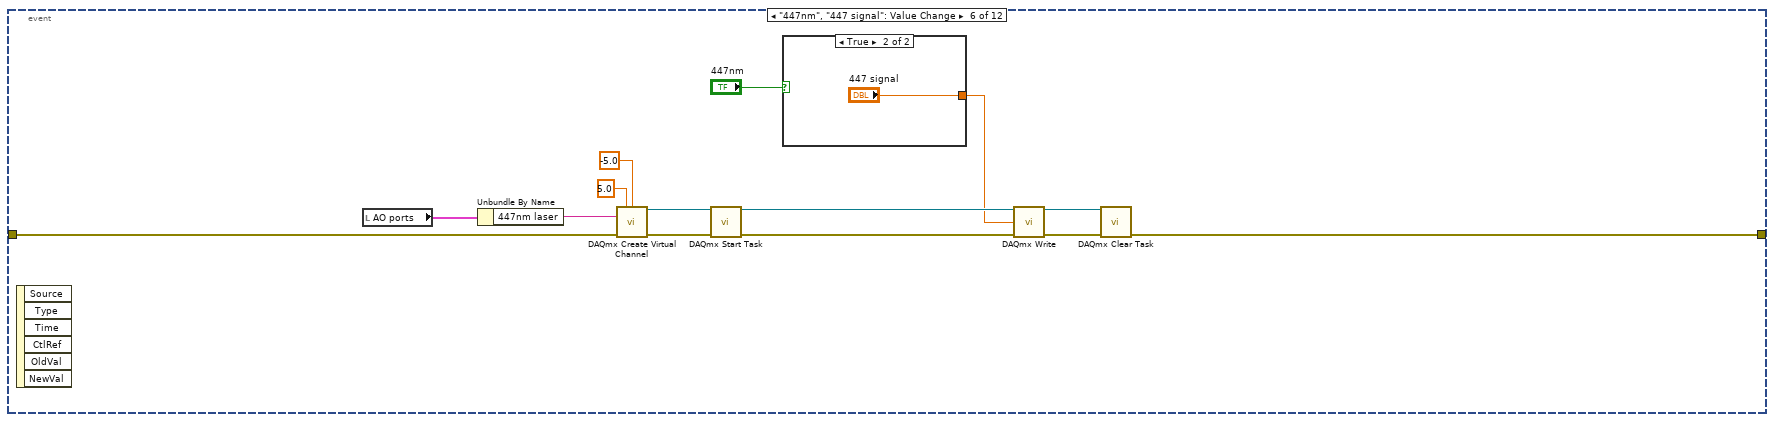
[diagram p15: hidden frame]
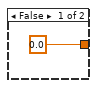
[diagram p16: hidden frame]
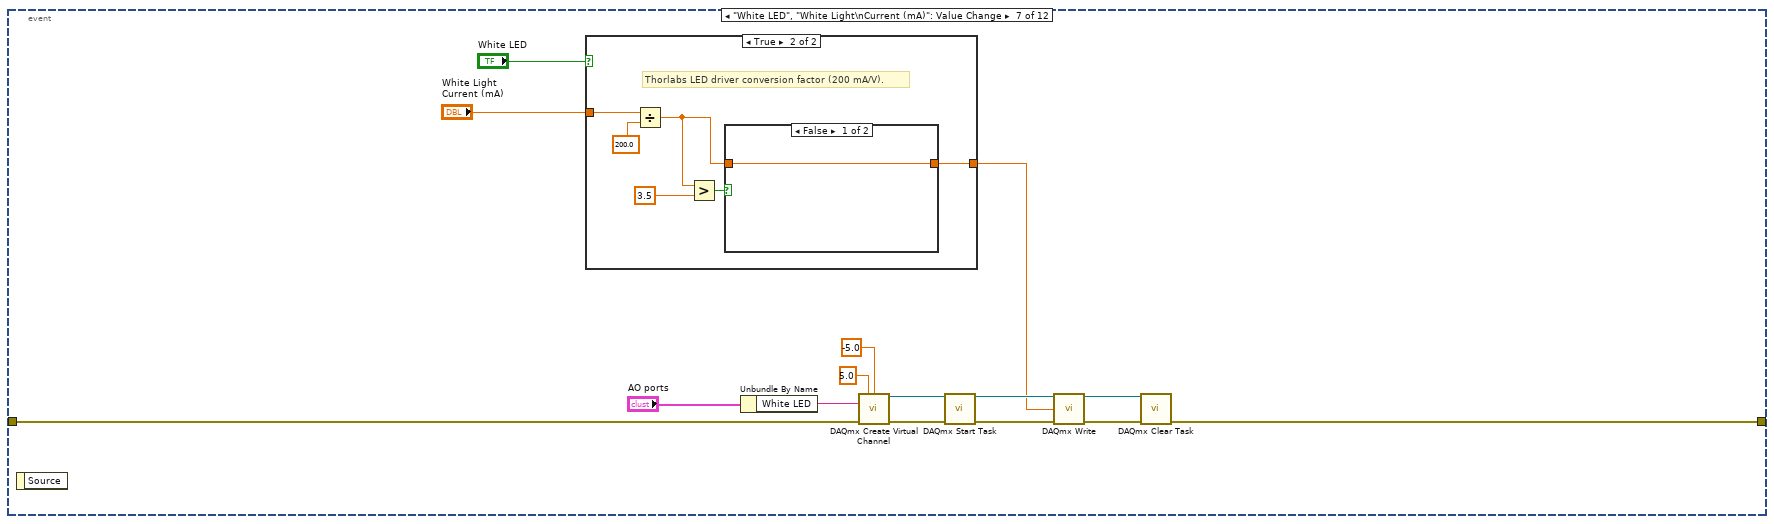
[diagram p17: hidden frame]
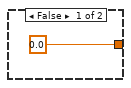
[diagram p18: hidden frame]
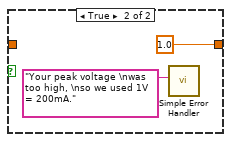
[diagram p19: hidden frame]
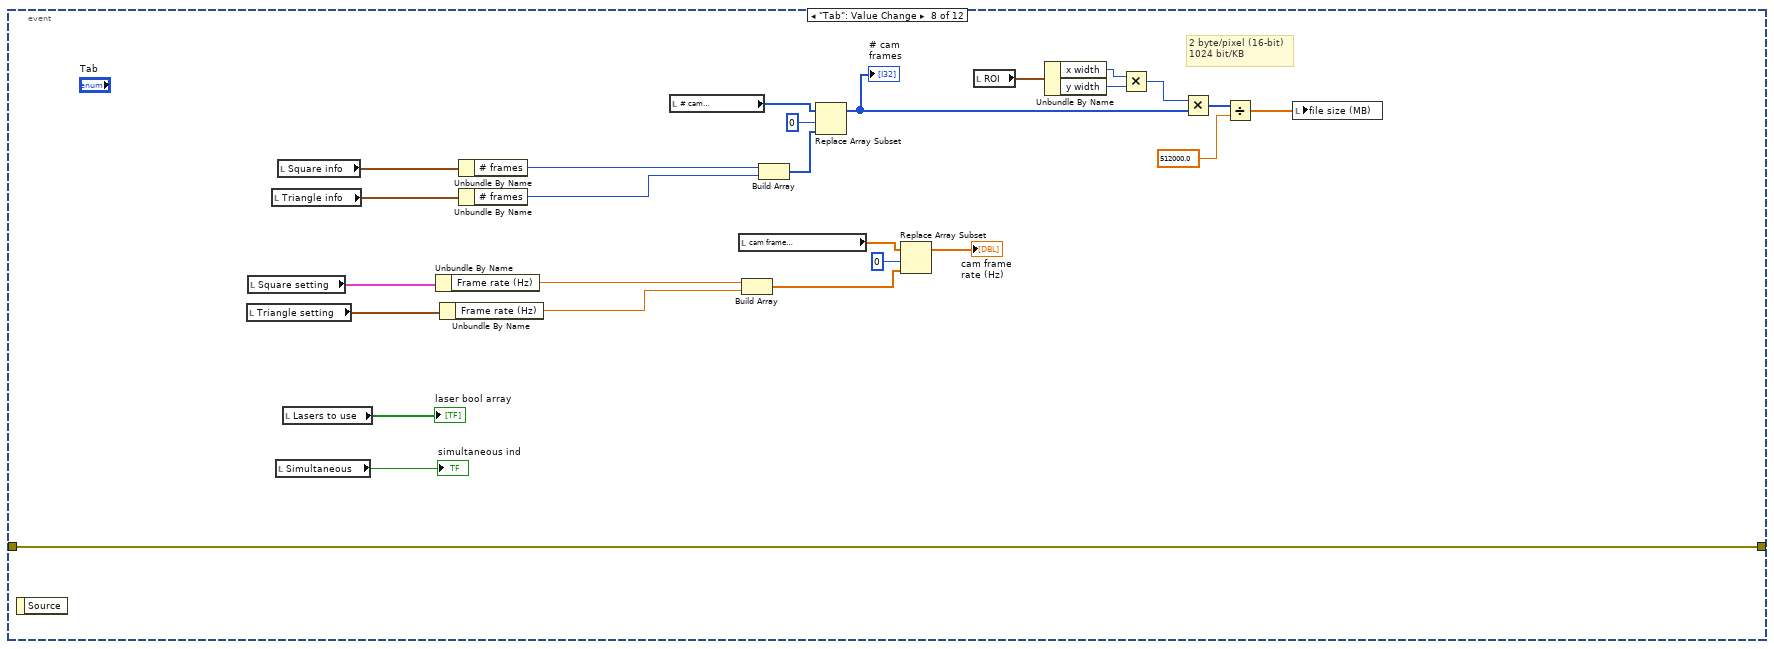
[diagram p20: hidden frame]
diagram:
  # "camera chip --> image graph\nH  --> y axis\nV   --> x axis"
  n1 = stacked-sequence {
    frame #0 {
      w42 = 1 items=["Internal"=1, "External"=2, "Software"=3] ("Trigger Source")
      w43 = 15 items=["BINNING"=1, "BITS PER CHANNEL"=2, "ACTIVE VIEW INDEX"=3, "CCD MODE"=4, "SENSOR MODE"=5, "READOUT MODE"=6, "EXPOSURE TIME"=7, "CONTRAST GAIN"=8, "CONTRAST OFFSET"=9, "LIGHT MODE"=10, "SENSITIVITY"=11, "WHITE BALANCE"=12, "PHOTON IMAGING MODE"=13, "HIGH DYNAMIC RANGE MODE"=14, "TRIGGER SOURCE"=15, "TRIGGER ACTIVE"=16, "TRIGGER MODE"=17, "TRIGGER POLARITY"=18, "TRIGGER GLOBAL EXPOSURE"=19, "FIRST TRIGGER BEHAVIOR"=20, "TRIGGER TIMES"=21, "OUTPUT TRIGGER POLARITY"=22, "OUTPUT TRIGGER DELAY"=23, "OUTPUT TRIGGER PERIOD"=24, "TEMPERATURE"=25, "TEMPERATURE TARGET"=26, "SENSOR COOLER FAN"=27, "MECHANICAL SHUTTER"=28, "BACK FOCUS POSITION"=29, "FRAMEBUNDLE MODE"=30, "FRAMEBUNDLE NUMBER"=31, "LINEBUNDLE HEIGHT"=32, "TRIGGER CONNECTOR"=33, "IMAGE PIXEL TYPE"=34] ("Parameter")
      w49 = 7 items=["BINNING"=1, "BITS PER CHANNEL"=2, "ACTIVE VIEW INDEX"=3, "CCD MODE"=4, "SENSOR MODE"=5, "READOUT MODE"=6, "EXPOSURE TIME"=7, "CONTRAST GAIN"=8, "CONTRAST OFFSET"=9, "LIGHT MODE"=10, "SENSITIVITY"=11, "WHITE BALANCE"=12, "PHOTON IMAGING MODE"=13, "HIGH DYNAMIC RANGE MODE"=14, "TRIGGER SOURCE"=15, "TRIGGER ACTIVE"=16, "TRIGGER MODE"=17, "TRIGGER POLARITY"=18, "TRIGGER GLOBAL EXPOSURE"=19, "FIRST TRIGGER BEHAVIOR"=20, "TRIGGER TIMES"=21, "OUTPUT TRIGGER POLARITY"=22, "OUTPUT TRIGGER DELAY"=23, "OUTPUT TRIGGER PERIOD"=24, "TEMPERATURE"=25, "TEMPERATURE TARGET"=26, "SENSOR COOLER FAN"=27, "MECHANICAL SHUTTER"=28, "BACK FOCUS POSITION"=29, "FRAMEBUNDLE MODE"=30, "FRAMEBUNDLE NUMBER"=31, "LINEBUNDLE HEIGHT"=32, "TRIGGER CONNECTOR"=33, "IMAGE PIXEL TYPE"=34] ("Parameter")
      w4 = errorcluster {"status"=FALSE, "code"=0, "source"=""} ("camera \ninitialization\nerror")
      w75 = u16 1 items=["Amplitude", "Efficiency"] ("Input type")
      w82 = u16 4 items=["1x1"=1, "2x2"=2, "4x4"=4] ("Bin (n x n)")
      w86 = 4 ("milliseconds to wait")
      w89 = 0 ("milliseconds to wait")
      w90 = 1 items=["BINNING"=1, "BITS PER CHANNEL"=2, "ACTIVE VIEW INDEX"=3, "CCD MODE"=4, "SENSOR MODE"=5, "READOUT MODE"=6, "EXPOSURE TIME"=7, "CONTRAST GAIN"=8, "CONTRAST OFFSET"=9, "LIGHT MODE"=10, "SENSITIVITY"=11, "WHITE BALANCE"=12, "PHOTON IMAGING MODE"=13, "HIGH DYNAMIC RANGE MODE"=14, "TRIGGER SOURCE"=15, "TRIGGER ACTIVE"=16, "TRIGGER MODE"=17, "TRIGGER POLARITY"=18, "TRIGGER GLOBAL EXPOSURE"=19, "FIRST TRIGGER BEHAVIOR"=20, "TRIGGER TIMES"=21, "OUTPUT TRIGGER POLARITY"=22, "OUTPUT TRIGGER DELAY"=23, "OUTPUT TRIGGER PERIOD"=24, "TEMPERATURE"=25, "TEMPERATURE TARGET"=26, "SENSOR COOLER FAN"=27, "MECHANICAL SHUTTER"=28, "BACK FOCUS POSITION"=29, "FRAMEBUNDLE MODE"=30, "FRAMEBUNDLE NUMBER"=31, "LINEBUNDLE HEIGHT"=32, "TRIGGER CONNECTOR"=33, "IMAGE PIXEL TYPE"=34] ("Parameter")
      w92 = 2 items=["BINNING"=1, "BITS PER CHANNEL"=2, "ACTIVE VIEW INDEX"=3, "CCD MODE"=4, "SENSOR MODE"=5, "READOUT MODE"=6, "EXPOSURE TIME"=7, "CONTRAST GAIN"=8, "CONTRAST OFFSET"=9, "LIGHT MODE"=10, "SENSITIVITY"=11, "WHITE BALANCE"=12, "PHOTON IMAGING MODE"=13, "HIGH DYNAMIC RANGE MODE"=14, "TRIGGER SOURCE"=15, "TRIGGER ACTIVE"=16, "TRIGGER MODE"=17, "TRIGGER POLARITY"=18, "TRIGGER GLOBAL EXPOSURE"=19, "FIRST TRIGGER BEHAVIOR"=20, "TRIGGER TIMES"=21, "OUTPUT TRIGGER POLARITY"=22, "OUTPUT TRIGGER DELAY"=23, "OUTPUT TRIGGER PERIOD"=24, "TEMPERATURE"=25, "TEMPERATURE TARGET"=26, "SENSOR COOLER FAN"=27, "MECHANICAL SHUTTER"=28, "BACK FOCUS POSITION"=29, "FRAMEBUNDLE MODE"=30, "FRAMEBUNDLE NUMBER"=31, "LINEBUNDLE HEIGHT"=32, "TRIGGER CONNECTOR"=33, "IMAGE PIXEL TYPE"=34] ("Parameter")
      w98 = u32 67109122 items=["BUS"=67109121, "CAMERA ID"=67109122, "VENDOR"=67109123, "MODEL"=67109124, "CAMERA VERSION"=67109125, "DRIVER VERSION"=67109126, "MODULE VERSIOIN"=67109127, "DCAMAPI VERSION"=67109128] ("Info ID")
      w97 = u32 67109124 items=["BUS"=67109121, "CAMERA ID"=67109122, "VENDOR"=67109123, "MODEL"=67109124, "CAMERA VERSION"=67109125, "DRIVER VERSION"=67109126, "MODULE VERSIOIN"=67109127, "DCAMAPI VERSION"=67109128] ("Info ID")
      w105 = u16 0 items=["Focus", "Square wave", "Triangle wave"] ("Camera mode")
      w106 = u16 0 items=["Full ROI", "Central quad", "Custom ROI"] ("ROI selection")
      w71 = FALSE ("stop program")
      # "update cursor in location indicator"
      # "initialize image indicator"
      # "initialize location indicator"
      # "get sensor size\ninitialize ROI to full frame\nset binning to 4x4 for fast display"
      # "total pixels\nwhen binning = 1x1"
      # "get camera info"
      # "Initialize camera and other variables"
      n2 = local write "Waveform generated"(w71) -> ()
      n3 = local write "Live"(w71) -> ()
      n4 = local write "Snap&Save"(w71) -> ()
      n5 = local write "Define ROI"(w71) -> ()
      n6 = local write "Update ROI"(w71) -> ()
      n7 = local write "Start acquisition"(w71) -> ()
      n8 = local write "stop program"(w71) -> ()
      n9 = local write "Test patch"(w71) -> ()
      n10 = local write "Save patch param"(w71) -> ()
      n11 = local write "Load Mem_AbsV waveform"(w71) -> ()
      n12 = while {
        tunnel: [w147] -> w5
        tunnel: [w146] -> w37
        stop <- w148 stop-if-true
        n13 = local read "Lasers to use"() -> (w146:bool[])
        n14 = Boolean To (0,1)(Boolean=w146) -> (0, 1=w149:i16[])
        n15 = Add Array Elements(numeric array=w149) -> (sum=w147:i16)
        n16 = Greater Than 0?(x=w147) -> (x > 0?=w148:bool)
      }
      n17 = call <userlib>:"tm_initialize.vi"("error in (no error)"=w4) -> ("error out"=w81:errorcluster, "Number Of Cameras"=w103:u32)  [unwired: 9 in]
      n18 = Not Equal To 0?(x=w103) -> (x != 0?=→"Initialize?":bool)
      n19 = local read "DAQ sampling rate"() -> (w10:dbl)
      n20 = local read "Square setting"() -> (w11:T8)
      n21 = local read "Simultaneous"() -> (w9:bool)
      n22 = local read "External"() -> (w7:dbl)
      n23 = flat-sequence {
        tunnel: w81 -> [w150]
        tunnel: [w150] -> w80
        frame #0 {
          n24 = Wait (ms)(milliseconds to wait=u32 500) -> ()  [unwired: 1 out]
        }
      }
      n25 = local read "Exposure (msec)"() -> (w48:dbl)
      n26 = call "subGenerateSquareWaveform_NW348.vi"("num colors"=w5, "Simultaneous"=w9, "error in (no error)"=w4, "Square wave settings"=w11, "External"=w7, "DAQ sampling rate"=w10) -> ("error out"=w8:errorcluster, "Info"=w13:T18, "Display Waveform"=w14:waveform(dbl)[])  [unwired: 3 out]
      n27 = local write "Bin (n x n)"(w82) -> ()
      n28 = call <userlib>:"tm_opencamera.vi"("error in (no error)"=w80, "Camera Index"=u32 0 ("milliseconds to wait")) -> ("error out"=w100:errorcluster, "Handle out"=w41:u32)  [unwired: 8 in]
      n29 = Divide(x=w48, y=1000.0 ("milliseconds to wait")) -> (x/y=w47:dbl)
      n30 = local write "Camera mode"(w105) -> ()
      n31 = local write "ROI selection"(w106) -> ()
      n32 = local write "Square Waveform"(w14) -> ()
      n33 = Build Array(u32 16711680, u32 16744192, u32 14872320, u32 5621760, u32 54255) -> (w24:u32[])
      n34 = Build Array("Red laser", "Orange laser", "Yellow laser", "Green laser", "Blue laser") -> (w25:string[])
      n35 = local write "Square info"(w13) -> ()
      n36 = call <userlib>:"tm_getcamerainfo.vi"("error in (no error)"=w100, "Info ID"=w97, "Handle in"=w41) -> ("error out"=w96:errorcluster, "String"=→"Model":string)  [unwired: 6 in, 1 out]
      n37 = call <userlib>:"tm_getcamerainfo.vi"("error in (no error)"=w96, "Info ID"=w98, "Handle in"=w41) -> ("error out"=w40:errorcluster, "String"=→"Camera ID":string)  [unwired: 6 in, 1 out]
      n38 = call <userlib>:"tm_getparameter.vi"("error in (no error)"=w40, "Parameter"=w92, "Handle in"=w41) -> ("error out"=w39:errorcluster, "Value out"=→"Bits per Channel":dbl)  [unwired: 6 in, 1 out]
      n39 = call <userlib>:"tm_setparameter.vi"("error in (no error)"=w39, "Value in"=w42, "Parameter"=w43, "Handle in"=w41) -> ("error out"=w38:errorcluster)  [unwired: 6 in, 1 out]
      n40 = call <userlib>:"tm_setparameter.vi"("error in (no error)"=w38, "Value in"=w82, "Parameter"=w90) -> ("error out"=w45:errorcluster)  [unwired: 7 in, 1 out]
      n41 = call <userlib>:"tm_setparameter.vi"("error in (no error)"=w45, "Value in"=w47, "Parameter"=w49) -> ("error out"=w44:errorcluster)  [unwired: 7 in, 1 out]
      n42 = local read "AOTF digital lines"() -> (w57:T5)
      n43 = local read "Shutter lines"() -> (w58:T4)
      n44 = for {
        shift-right: [w125] -> w23
        shift-left: 1 -> [w126]
        tunnel: w37 -> [w127] mode=indexing
        tunnel: w25 -> [w124] mode=indexing
        tunnel: w24 -> [w123] mode=indexing
        tunnel: TRUE ("Plot.Visible") -> [w122]
        n45 = case shown="True" w127 {
          tunnel: w126 -> [w128 w129]
          tunnel: [w128 w133] -> w125
          tunnel: w124 -> [_ w131]
          tunnel: w123 -> [_ w130]
          tunnel: w122 -> [_ w132]
          frame False {
          }
          frame True {
            n46 = stacked-sequence {
              tunnel: w132 -> [w134 w139 w144]
              tunnel: w131 -> [w135 w138 w143]
              tunnel: w130 -> [w137 w140 w145]
              tunnel: w129 -> [w136 w141 w142]
              frame #0 {
                n47 = property on="Square Waveform" class="WFGraph (strict)"("Active Plot"=w136, "Plot.Plot Color"=w137, "Plot.Visible?"=w134, "Plot.Plot Name"=w135) -> ()  [unwired: 2 in, 2 out]
              }
              frame #1 {
                n48 = property on="Triangle Waveform" class="WFGraph (strict)"("Active Plot"=w141, "Plot.Plot Color"=w140, "Plot.Visible?"=w139, "Plot.Plot Name"=w138) -> ()  [unwired: 2 in, 2 out]
              }
              frame #2 {
                n49 = property on="Laser Pump Waveform" class="WFGraph (strict)"("Active Plot"=w142, "Plot.Plot Color"=w145, "Plot.Visible?"=w144, "Plot.Plot Name"=w143) -> ()  [unwired: 2 in, 2 out]
              }
            }
            n50 = Increment(x=w129) -> (x+1=w133:i32)
          }
        }
      }
      n51 = local read "Triangle setting"() -> (w12:T9)
      n52 = local read "AOTF\ndigital"() -> (w53:bool[])
      n53 = local read "Shutters"() -> (w52:bool[])
      n54 = Cluster To Array(cluster=w58) -> (array=w56:tag[])
      n55 = Cluster To Array(cluster=w57) -> (array=w55:tag[])
      n56 = call <userlib>:"tm_getarea_a.vi"("error in (no error)"=w44, "Handle in"=w41) -> ("error out"=w60:errorcluster, "H Width"=w94:T19, "V Width"=w93:T19)  [unwired: 4 in, 3 out]
      n57 = Unbundle(w93) -> ("Maximum"=w79:i32)  [unwired: 3 out]
      n58 = Unbundle(w94) -> ("Maximum"=w83:i32)  [unwired: 3 out]
      n59 = Build Array (concatenate)(w52, w53) -> (w51:bool[])
      n60 = Build Array (concatenate)(w56, w55) -> (w54:tag[])
      n61 = property on="Image" class="IntGraph (strict)"("ZScale.MarkerVals[]"=cluster{dbl, u32}[] [{0.0, 0}, {1.0, 16448250}] ("Z Scale.Marker Values[]")) -> ()  [unwired: 2 in, 2 out]
      n62 = call "subGenerateTriangleWaveform_NW348.vi"("num colors"=w5, "Simultaneous"=w9, "error in (no error)"=w8, "Triangle wave settings"=w12, "External"=w7, "DAQ sampling rate"=w10) -> ("error out"=w6:errorcluster, "Triangle info"=w17:T20, "Triangle Waveform"=w18:waveform(dbl)[])  [unwired: 3 out]
      n63 = call "subSetDigStates_NW348.vi"("Error in (no error)"=w60, "Digital line array"=w54, "Digital state array"=w51) -> ("Error out"=w59:errorcluster)  [unwired: 8 in]
      n64 = Multiply(x=w83, y=w86) -> (x*y=→"x pixels":i32)
      n65 = Multiply(x=w79, y=w86) -> (x*y=→"y pixels":i32)
      n66 = Initialize Array(u16 0 ("element"), w83, w83) -> (→"Image":u16[][])
      n67 = local read "ROI"() -> (w102:T1)
      n68 = Bundle By Name(cluster=w102, "x offset"=w89, "y offset"=w89, "x width"=w83, "y width"=w79) -> (w72:T1)
      "ROI" <- w72
      n69 = local write "Triangle Waveform"(w18) -> ()
      n70 = local write "Triangle info"(w17) -> ()
      n71 = local read "AOTF efficiency"() -> (w69:dbl[])
      n72 = local read "AOTF info"() -> (w74:T3)
      n73 = local read "Pump setting"() -> (w16:T11)
      n74 = Subtract(x=6, y=w23) -> (x-y=w21:i32)
      n75 = call "subUpdateLocIndicator_NW348.vi"("ROI"=w72, "pixel range"=w83) -> ("Graph scale"=w85:T21, "Location indicator"=→"Location indicator":u16[][])  [unwired: 8 in]
      n76 = for {
        N: w21 -> [_]
        tunnel: w23 -> [w109]
        i -> [w108]
        n77 = Add(x=w109, y=w108) -> (x+y=w112:i32)
        n78 = stacked-sequence {
          tunnel: w112 -> [w115 w118 w119]
          tunnel: "" ("Plot.Plot Name") -> [w114 w116 w120]
          tunnel: FALSE ("Plot.Visible") -> [w113 w117 w121]
          frame #0 {
            n79 = property on="Square Waveform" class="WFGraph (strict)"("Active Plot"=w115, "Plot.Visible?"=w113, "Plot.Plot Name"=w114) -> ()  [unwired: 2 in, 2 out]
          }
          frame #1 {
            n80 = property on="Triangle Waveform" class="WFGraph (strict)"("Active Plot"=w118, "Plot.Visible?"=w117, "Plot.Plot Name"=w116) -> ()  [unwired: 2 in, 2 out]
          }
          frame #2 {
            n81 = property on="Laser Pump Waveform" class="WFGraph (strict)"("Active Plot"=w119, "Plot.Visible?"=w121, "Plot.Plot Name"=w120) -> ()  [unwired: 2 in, 2 out]
          }
        }
      }
      n82 = call "subAOTFamplitude_6channels_NW348.vi"("AOTF info"=w74, "Input type"=w75, "Error in"=w59, "Efficiency In"=w69) -> ("Error out"=w50:errorcluster, "Efficiency Out"=w70:dbl[], "Amplitude Out"=w76:u16[])  [unwired: 5 in]
      n83 = Unbundle By Name(w85) -> ("X min"=w65:dbl, "Y min"=w64:dbl, "X max"=w62:dbl, "Y max"=w61:dbl)
      n84 = local write "AOTF efficiency"(w70) -> ()
      n85 = local write "AOTF amplitude"(w76) -> ()
      n86 = call "subGenerateLaserPumpWaveform_NW348.vi"("num colors"=w5, "Simultaneous"=w9, "error in (no error)"=w6, "Laser pump settings"=w16, "A & D I/O\nsampling rate"=w10) -> ("error out"=w3:errorcluster, "num. output\nsamples L"=w19:u32, "Display Waveform"=w15:waveform(dbl)[])  [unwired: 2 in, 2 out]
      n87 = property on="Image" class="IntGraph (strict)"("XScale.Minimum"=w65, "YScale.Minimum"=w64, "XScale.Maximum"=w62, "YScale.Maximum"=w61) -> ()  [unwired: 2 in, 2 out]
      n88 = local read "Emission filter"() -> (w73:u16)
      n89 = local write "Laser Pump Waveform"(w15) -> ()
      n90 = local write "# output\nsamples L"(w19) -> ()
      n91 = property on="Location indicator" class="IntGraph (strict)"("Active Cursor"=u16 1 ("element"), "Cursor.Visible"=TRUE, "Cursor.Cursor X"=w62, "Cursor.Cursor Y"=w61) -> ()  [unwired: 2 in, 2 out]
      n92 = property on="Location indicator" class="IntGraph (strict)"("Active Cursor"=u16 0 ("element"), "Cursor.Visible"=TRUE, "Cursor.Cursor X"=w65, "Cursor.Cursor Y"=w64) -> ()  [unwired: 2 in, 2 out]
      n93 = call "subFilterWheelSet_NW348.vi"("Error in"=w50, "Filter Wheel Position - Control"=w73) -> ("Error out"=w2:errorcluster)  [unwired: 9 in]
      n94 = Merge Errors(w2, w3) -> (→"Error":errorcluster)
    }
    frame #1 {
      n95 = while {
        shift-right: [w423] -> _
        shift-left: _ -> [w424]
        shift-right: [w421] -> _
        shift-left: _ -> [w422]
        stop <- "stop program" stop-if-true
        # "Camera Events"
        n96 = local read "Error"() -> (w426:errorcluster)
        n97 = event shown="[11] \"Start acquisition\": Value Change" {
          selector: _ -> [_ _ _ _ _ _ _ _ _ _ _ _]
          dyn-events: _ -> [_ _ _ _ _ _ _ _ _ _ _ _]
          timeout: 0 -> [_ _ _ _ _ _ _ _ _ _ _ _]
          tunnel: w426 -> [w442 w518 w532 w596 w701 w724 w782 w856 w894 w977 w989 w1001]
          tunnel: w422 -> [w441 w519 w531 w595 w702 w723 w781 w855 w895 w978 w990 w1000]
          tunnel: w424 -> [w432 w515 _ _ w703 _ w776 _ _ w979 w991 w992]
          tunnel: [w429 w515 w528 w586 w703 w718 w778 w850 w888 w979 w991 w999] -> w423
          tunnel: [w433 w517 w529 w588 w702 w715 w779 w852 w881 w978 w990 w998] -> w421
          tunnel: [w434 w516 w530 w589 w701 w716 w780 w853 w882 w977 w989 w997] -> w425
          event Timeout {
            n98 = event-data() -> ()  [unwired: 1 in, 1 out]
            n99 = local read "Define ROI"() -> (w431:bool)
            n100 = local read "Live"() -> (w430:bool)
            n101 = case shown="True" w430 {
              tunnel: w442 -> [w444 w457]
              tunnel: w441 -> [w445 w456]
              tunnel: [w444 w455] -> w434
              tunnel: [w445 w454] -> w433
              tunnel: w432 -> [_ w450]
              tunnel: [T16 {"width"=0, "height"=0, "datatype"=0} ("Buffer") w450] -> w429
              frame False {
              }
              frame True {
                n102 = local read "Bin (n x n)"() -> (w448:u16)
                n103 = local read "x pixels"() -> (w447:i32)
                n104 = call <userlib>:"tm_waitnextframe.vi"("error in (no error)"=w457, "Handle in"=w456) -> ("error out"=w458:errorcluster, "Frame Index"=w460:i32, "Handle out"=w459:u32)  [unwired: 6 in, 1 out]
                n105 = Divide(x=w447, y=w448) -> (x/y=w446:dbl)
                n106 = call <userlib>:"tm_getframe_a.vi"("error in (no error)"=w458, "Frame Index"=w460, "Buffer"=w450, "Handle in"=w459) -> ("error out"=w455:errorcluster, "Data 16"=w452:u16[][], "Handle out"=w454:u32)  [unwired: 4 in, 1 out]
                n107 = local read "ROI"() -> (w453:T1)
                n108 = call "subPadImage_NW348.vi"("ROI"=w453, "Full size"=w446, "Image in"=w452) -> ("image info"=→"Image info":T22, "Image out"=w451:u16[][])  [unwired: 7 in]
                n109 = local write "Image"(w451) -> ()
              }
            }
            n110 = case shown="True" w431 {
              frame False {
              }
              frame True {
                w465 = u32 4 ("Active Cursor")
                # "set ROI cursor"
                # "2 byte/pixel (16-bit)\n1024 bit/KB"
                # "calculate frame rate\nbased on cursor"
                # "update cursor info"
                n111 = local read "Bin (n x n)"() -> (w466:u16)
                n112 = property on="Image" class="IntGraph (strict)"("Active Cursor"=u32 0) -> ("Cursor.Cursor X"=w497:dbl, "Cursor.Cursor Y"=w498:dbl)  [unwired: 2 in, 2 out]
                n113 = property on="Image" class="IntGraph (strict)"("Active Cursor"=u32 1) -> ("Cursor.Cursor X"=w499:dbl, "Cursor.Cursor Y"=w500:dbl)  [unwired: 2 in, 2 out]
                n114 = local read "x pixels"() -> (w468:i32)
                n115 = Divide(x=w468, y=w466) -> (x/y=w467:dbl)
                n116 = Bundle("Cursor.Cursor X"=w497, "Cursor.Cursor Y"=w498, "Cursor.Cursor X"=w499, "Cursor.Cursor Y"=w500) -> (w501:T23)  [unwired: 1 in]
                n117 = call "subApplyCursorLimit_NW348.vi"("Cursor limit"=w467, "Cursor input"=w501, "Symmetrical ROI"="Symmetrical") -> ("Cursor output"=w476:T24)  [unwired: 2 in]
                n118 = Unbundle By Name(w476) -> ("Cursor1. X"=w480:dbl, "Cursor1. Y"=w479:dbl)
                n119 = Unbundle By Name(w476) -> ("Cursor2. X"=w478:dbl, "Cursor2. Y"=w477:dbl)
                n120 = Unbundle By Name(w476) -> ("Cursor1. X"=w475:dbl, "Cursor2. X"=w474:dbl, "Cursor1. Y"=w473:dbl, "Cursor2. Y"=w472:dbl)
                n121 = property on="Image" class="IntGraph (strict)"("Active Cursor"=u32 0, "Cursor.Cursor X"=w480, "Cursor.Cursor Y"=w479) -> ()  [unwired: 2 in, 2 out]
                n122 = property on="Image" class="IntGraph (strict)"("Active Cursor"=u32 1, "Cursor.Cursor X"=w478, "Cursor.Cursor Y"=w477) -> ()  [unwired: 2 in, 2 out]
                n123 = Max & Min(x=w475, y=w474) -> (max(x,y)=w494:dbl, min(x,y)=w486:dbl)
                n124 = Max & Min(x=w473, y=w472) -> (max(x,y)=w493:dbl, min(x,y)=w484:dbl)
                n125 = Subtract(x=w494, y=w486) -> (x-y=w487:dbl)
                n126 = Subtract(x=w493, y=w484) -> (x-y=w485:dbl)
                n127 = local read "# cam\nframes"() -> (w490:i32[])
                n128 = Multiply(x=w487, y=w485) -> (x*y=w492:dbl)
                n129 = local read "ROI cursor"() -> (w488:T1)
                n130 = Bundle By Name(cluster=w488, "x width"=w487, "x offset"=w486, "y width"=w485, "y offset"=w484) -> (w462:T1)
                n131 = Multiply(x=w490, y=w492) -> (x*y=w491:dbl[])
                n132 = local read "cam frame\nrate (Hz)"() -> (w483:dbl[])
                n133 = Divide(x=w491, y=512000.0) -> (x/y=→"file size (MB)":dbl[])
                n134 = Divide(x=w462, y=w465) -> (x/y=w463:T25)
                n135 = local read "Measurements"() -> (w482:T12)
                n136 = Round To Nearest(number=w463) -> (nearest integer value=w464:T25)
                n137 = Multiply(x=w464, y=w465) -> (x*y=w461:T25)
                "ROI cursor" <- w461
                n138 = call "subGetMaxCameraRate_NW384.vi"("measure bool cluster"=w482, "cam frame\nrate (Hz)"=w483, "Bin (n x n)"=w466, "ROI"=w461, "Binned pixels"=w467) -> ("max frame rate (Hz)"=→"max frame rate (Hz)":dbl, "ROI too large"=w471:bool)  [unwired: 5 in]
                n139 = Select(t=u32 16723242, s=w471, f=u32 14745528) -> (s? t:f=w504:u32)
                n140 = property on="max frame rate (Hz)" class="DigNum (strict)"("NumText.BGColor"=w504) -> ()  [unwired: 2 in, 2 out]
              }
            }
            n141 = property on="Image" class="IntGraph (strict)"() -> ("XScale.Minimum"=w437:dbl, "YScale.Minimum"=w438:dbl, "XScale.Maximum"=w439:dbl, "YScale.Maximum"=w440:dbl)  [unwired: 2 in, 2 out]
            n142 = property on="Location indicator" class="IntGraph (strict)"("Active Cursor"=u32 0, "Cursor.Cursor X"=w437, "Cursor.Cursor Y"=w438) -> ()  [unwired: 2 in, 2 out]
            n143 = property on="Location indicator" class="IntGraph (strict)"("Active Cursor"=u32 1, "Cursor.Cursor X"=w439, "Cursor.Cursor Y"=w440) -> ()  [unwired: 2 in, 2 out]
          }
          event "Exposure (msec)", "Camera mode": Value Change {
            w520 = 7 items=["BINNING"=1, "BITS PER CHANNEL"=2, "ACTIVE VIEW INDEX"=3, "CCD MODE"=4, "SENSOR MODE"=5, "READOUT MODE"=6, "EXPOSURE TIME"=7, "CONTRAST GAIN"=8, "CONTRAST OFFSET"=9, "LIGHT MODE"=10, "SENSITIVITY"=11, "WHITE BALANCE"=12, "PHOTON IMAGING MODE"=13, "HIGH DYNAMIC RANGE MODE"=14, "TRIGGER SOURCE"=15, "TRIGGER ACTIVE"=16, "TRIGGER MODE"=17, "TRIGGER POLARITY"=18, "TRIGGER GLOBAL EXPOSURE"=19, "FIRST TRIGGER BEHAVIOR"=20, "TRIGGER TIMES"=21, "OUTPUT TRIGGER POLARITY"=22, "OUTPUT TRIGGER DELAY"=23, "OUTPUT TRIGGER PERIOD"=24, "TEMPERATURE"=25, "TEMPERATURE TARGET"=26, "SENSOR COOLER FAN"=27, "MECHANICAL SHUTTER"=28, "BACK FOCUS POSITION"=29, "FRAMEBUNDLE MODE"=30, "FRAMEBUNDLE NUMBER"=31, "LINEBUNDLE HEIGHT"=32, "TRIGGER CONNECTOR"=33, "IMAGE PIXEL TYPE"=34] ("Parameter")
            n144 = event-data() -> ()  [unwired: 1 in, 1 out]
            n145 = local read "cam frame\nrate (Hz)"() -> (w514:dbl[])
            n146 = Reciprocal(x=w514) -> (1/x=w513:dbl[])
            n147 = Divide(x="Exposure (msec)", y=1000.0 ("milliseconds to wait")) -> (x/y=w511:dbl)
            n148 = Build Array (concatenate)(w511, w513) -> (w510:dbl[])
            n149 = Index Array(array=w510, index="Camera mode") -> (element=w508:dbl)
            n150 = call <userlib>:"tm_setparameter.vi"("error in (no error)"=w518, "Value in"=w508, "Parameter"=w520, "Handle in"=w519) -> ("error out"=w516:errorcluster, "Handle out"=w517:u32)  [unwired: 6 in]
          }
          event "Bin (n x n)": Value Change {
            # "calculate frame rate\nbased on ROI"
            n151 = event-data() -> ("OldVal"=w553:u16, "NewVal"=w522:u16)  [unwired: 1 in]
            n152 = local read "Live"() -> (w533:bool)
            n153 = case shown="True" w533 {
              tunnel: [w578 w583] -> w523
              tunnel: [w579 w582] -> w524
              tunnel: w531 -> [w579 w581]
              tunnel: w532 -> [w578 w580]
              frame False {
              }
              frame True {
                n154 = call <userlib>:"tm_stopcapture.vi"("error in (no error)"=w580, "Handle in"=w581) -> ("error out"=w584:errorcluster, "Handle out"=w585:u32)  [unwired: 8 in]
                n155 = call <userlib>:"tm_unpreparecapture.vi"("error in (no error)"=w584, "Handle in"=w585) -> ("error out"=w583:errorcluster, "Handle out"=w582:u32)  [unwired: 8 in]
              }
            }
            n156 = local read "x pixels"() -> (w552:i32)
            n157 = Divide(x=w552, y="Bin (n x n)") -> (x/y=w546:dbl)
            n158 = property on="Image" class="IntGraph (strict)"() -> ("XScale.Minimum"=w544:dbl, "YScale.Minimum"=w543:dbl, "XScale.Maximum"=w542:dbl, "YScale.Maximum"=w541:dbl)  [unwired: 2 in, 2 out]
            n159 = property on="Image" class="IntGraph (strict)"("Active Cursor"=u32 0) -> ("Cursor.Cursor Position"=w565:T26)  [unwired: 2 in, 2 out]
            n160 = property on="Image" class="IntGraph (strict)"("Active Cursor"=u32 1) -> ("Cursor.Cursor Position"=w566:T26)  [unwired: 2 in, 2 out]
            n161 = Bundle("XScale.Minimum"=w544, "YScale.Minimum"=w543, "XScale.Maximum"=w542, "YScale.Maximum"=w541) -> (w540:T27)  [unwired: 1 in]
            n162 = Bundle("Cursor.Cursor Position"=w565, "Cursor.Cursor Position"=w566) -> (w539:T28)  [unwired: 1 in]
            n163 = local read "ROI"() -> (w537:T1)
            n164 = call "subUpdateCameraBin_NW348.vi"("Bin (n x n)"=w522, "Previous bin"=w553, "Cursor in"=w539, "Error in (no error)"=w523, "Graph scale in"=w540, "ROI in"=w537, "Handle in"=w524) -> ("Error out"=w525:errorcluster, "Graph scale out"=w560:T27, "ROI out"=w536:T1, "Handle out"=w526:u32, "Cursor out"=w538:T29)
            n165 = local write "ROI"(w536) -> ()
            n166 = call "subUpdateLocIndicator_NW348.vi"("ROI"=w536, "pixel range"=w546) -> ("Location indicator"=w551:u16[][])  [unwired: 8 in, 1 out]
            n167 = Unbundle(w538) -> ("Cursor1.Position"=w555:T26, "Cursor2.Position"=w554:T26)
            n168 = local read "cam frame\nrate (Hz)"() -> (w547:dbl[])
            n169 = local read "Measurements"() -> (w545:T12)
            n170 = Unbundle By Name(w560) -> ("XScale.Minimum"=w559:dbl, "YScale.Minimum"=w558:dbl, "XScale.Maximum"=w557:dbl, "YScale.Maximum"=w556:dbl)
            n171 = local write "Location indicator"(w551) -> ()
            n172 = property on="Image" class="IntGraph (strict)"("Active Cursor"=u32 0, "Cursor.Cursor Position"=w555) -> ()  [unwired: 2 in, 2 out]
            n173 = property on="Image" class="IntGraph (strict)"("Active Cursor"=u32 1, "Cursor.Cursor Position"=w554) -> ()  [unwired: 2 in, 2 out]
            n174 = call "subGetMaxCameraRate_NW384.vi"("measure bool cluster"=w545, "cam frame\nrate (Hz)"=w547, "Bin (n x n)"="Bin (n x n)", "ROI"=w536, "Binned pixels"=w546) -> ("max frame rate (Hz)"=w534:dbl, "ROI too large"=w535:bool)  [unwired: 5 in]
            n175 = property on="Image" class="IntGraph (strict)"("XScale.Minimum"=w559, "YScale.Minimum"=w558, "XScale.Maximum"=w557, "YScale.Maximum"=w556) -> ()  [unwired: 2 in, 2 out]
            n176 = local write "max frame rate (Hz)"(w534) -> ()
            n177 = Select(t=u32 16723242, s=w535, f=u32 14745528) -> (s? t:f=w548:u32)
            n178 = property on="max frame rate (Hz)" class="DigNum (strict)"("NumText.BGColor"=w548) -> ()  [unwired: 2 in, 2 out]
            n179 = local read "Live"() -> (w527:bool)
            n180 = case shown="True" w527 {
              tunnel: w526 -> [w569 w574]
              tunnel: w525 -> [w568 w573]
              tunnel: [w568 w572] -> w530
              tunnel: [w569 w571] -> w529
              tunnel: [T16 {"width"=0, "height"=0, "datatype"=0} ("Buffer") w570] -> w528
              frame False {
              }
              frame True {
                w575 = 1 items=["Snap", "Sequence"] ("Capture mode")
                n181 = call <userlib>:"tm_preparecapture.vi"("error in (no error)"=w573, "Capture mode"=w575, "Handle in"=w574) -> ("error out"=w577:errorcluster, "Buffer"=w570:T16, "Handle out"=w576:u32)  [unwired: 5 in, 1 out]
                n182 = call <userlib>:"tm_startcapture_b.vi"("error in (no error)"=w577, "Handle in"=w576) -> ("error out"=w572:errorcluster, "Handle out"=w571:u32)  [unwired: 8 in]
              }
            }
          }
          event "Update ROI": Value Change {
            n183 = event-data() -> ()  [unwired: 1 in, 1 out]
            n184 = local read "Live"() -> (w592:bool)
            n185 = case shown="False" w592 {
              tunnel: [w618 w623] -> w593
              tunnel: [w619 w622] -> w594
              tunnel: w596 -> [w618 w621]
              tunnel: w595 -> [w619 w620]
              frame False {
              }
              frame True {
                n186 = call <userlib>:"tm_stopcapture.vi"("error in (no error)"=w621, "Handle in"=w620) -> ("error out"=w624:errorcluster, "Handle out"=w625:u32)  [unwired: 8 in]
                n187 = call <userlib>:"tm_unpreparecapture.vi"("error in (no error)"=w624, "Handle in"=w625) -> ("error out"=w623:errorcluster, "Handle out"=w622:u32)  [unwired: 8 in]
              }
            }
            n188 = flat-sequence {
              tunnel: [w631] -> w606
              tunnel: ["ROI selection"] -> w605
              tunnel: w594 -> [w627]
              tunnel: w593 -> [w626]
              tunnel: [w627] -> w603
              tunnel: [w626] -> w602
              tunnel: [w630] -> w599
              tunnel: w606 -> [w640]
              tunnel: w605 -> [w639]
              tunnel: [w638] -> w604
              tunnel: w603 -> [w638]
              tunnel: w602 -> [w637]
              tunnel: [w637] -> w601
              tunnel: [w636] -> w600
              tunnel: w599 -> [w636]
              tunnel: [w635] -> w598
              tunnel: [w634] -> w597
              tunnel: [w665] -> w590
              tunnel: [w666] -> w591
              tunnel: w604 -> [w689]
              tunnel: w601 -> [w688]
              tunnel: w600 -> [w687]
              tunnel: w598 -> [w686]
              tunnel: w597 -> [w670]
              frame #0 {
                n189 = local read "Bin (n x n)"() -> (w630:u16)
                "Previous Bin" <- w630
                n190 = local read "ROI"() -> (→"Previous ROI":T1)
                n191 = local read "Define ROI"() -> (w631:bool)
                n192 = local write "Update ROI"(FALSE ("Update ROI")) -> ()
                n193 = property on="Previous ROI" class="Bool (strict)"("DisabledEnum"=T17."Enabled" ("Disabled")) -> ()  [unwired: 2 in, 2 out]
              }
              frame #1 {
                n194 = case shown="False" w640 {
                  tunnel: [w643 w662] -> w634
                  tunnel: w639 -> [w642 _]
                  tunnel: [w641 w659] -> w635
                  frame False {
                    n195 = case shown="1" w642 {
                      tunnel: [w648 w654] -> w643
                      tunnel: [w647 w653] -> w641
                      frame 0, Default {
                        w647 = u16 4 items=["1x1"=1, "2x2"=2, "4x4"=4] ("Bin (n x n)")
                        w649 = u32 0 ("Active Cursor")
                        # "full ROI"
                        n196 = local read "Previous Bin"() -> (w646:u16)
                        n197 = local read "x pixels"() -> (w645:i32)
                        n198 = local write "Bin (n x n)"(w647) -> ()
                        n199 = Divide(x=w645, y=w646) -> (x/y=w644:dbl)
                        n200 = Bundle("Active Cursor"=w649, "Active Cursor"=w649, w644, w644) -> (w648:T30)  [unwired: 1 in]
                      }
                      frame 1 {
                        w653 = u16 2 items=["1x1"=1, "2x2"=2, "4x4"=4] ("Bin (n x n)")
                        # "Central quadrant"
                        n201 = local read "Previous Bin"() -> (w651:u16)
                        n202 = local read "x pixels"() -> (w652:i32)
                        n203 = Divide(x=w652, y=w651) -> (x/y=w650:dbl)
                        n204 = local write "Bin (n x n)"(w653) -> ()
                        n205 = Multiply(x=0.25, y=w650) -> (x*y=w657:dbl)
                        n206 = Multiply(x=w650, y=0.5) -> (x*y=w655:dbl)
                        n207 = Bundle(w657, w657, w655, w655) -> (w654:cluster{dbl, dbl, dbl, dbl})  [unwired: 1 in]
                      }
                    }
                  }
                  frame True {
                    w659 = u16 1 items=["1x1"=1, "2x2"=2, "4x4"=4] ("Bin (n x n)")
                    w661 = u16 2 items=["Full ROI", "Central quad", "Custom ROI"] ("ROI selection")
                    w660 = FALSE ("Visible")
                    n208 = local write "Define ROI"(w660) -> ()
                    n209 = property on="Image" class="IntGraph (strict)"("Active Cursor"=u32 0, "Cursor.Visible"=w660) -> ()  [unwired: 2 in, 2 out]
                    n210 = property on="Image" class="IntGraph (strict)"("Active Cursor"=u32 1, "Cursor.Visible"=w660) -> ()  [unwired: 2 in, 2 out]
                    n211 = local write "ROI selection"(w661) -> ()
                    n212 = local read "ROI cursor"() -> (w662:T1)
                    n213 = local write "Bin (n x n)"(w659) -> ()
                  }
                }
              }
              frame #2 {
                # "cursor position = ROI"
                # "calculate frame rate\nbased on ROI"
                # "new pixel range"
                # "update ROI with new camera bin"
                n214 = call "subUpdateCameraBin_NW348.vi"("Bin (n x n)"=w686, "Previous bin"=w687, "Error in (no error)"=w688, "ROI in"=w670, "Handle in"=w689) -> ("Error out"=w691:errorcluster, "ROI out"=w669:T1, "Handle out"=w692:u32)  [unwired: 2 in, 2 out]
                n215 = local read "cam frame\nrate (Hz)"() -> (w682:dbl[])
                n216 = local read "Bin (n x n)"() -> (w672:u16)
                n217 = Unbundle By Name(w669) -> ("x offset"=w679:i32, "y offset"=w681:i32, "x width"=w678:i32, "y width"=w680:i32)
                n218 = call "subImageROI2CameraROI_NW348.vi"("image ROI"=w669) -> ("camera ROI"=w690:T1)
                n219 = local write "ROI"(w669) -> ()
                n220 = local read "x pixels"() -> (w693:i32)
                n221 = local read "Measurements"() -> (w671:T12)
                n222 = call <userlib>:"tm_setarea.vi"("error in (no error)"=w691, "Sub Region"=w690, "Handle in"=w692) -> ("error out"=w665:errorcluster, "Handle out"=w666:u32)  [unwired: 7 in]
                n223 = Divide(x=w693, y=w672) -> (x/y=w673:dbl)
                n224 = Add(x=w681, y=w680) -> (x+y=w677:i32)
                n225 = call "subUpdateLocIndicator_NW348.vi"("ROI"=w669, "pixel range"=w673) -> ("Graph scale"=w694:T21, "Location indicator"=w699:u16[][])  [unwired: 8 in]
                n226 = call "subGetMaxCameraRate_NW384.vi"("measure bool cluster"=w671, "cam frame\nrate (Hz)"=w682, "Bin (n x n)"=w672, "ROI"=w669, "Binned pixels"=w673) -> ("max frame rate (Hz)"=w668:dbl, "ROI too large"=w667:bool)  [unwired: 5 in]
                n227 = Add(x=w679, y=w678) -> (x+y=w676:i32)
                n228 = property on="Image" class="IntGraph (strict)"("Active Cursor"=u32 0, "Cursor.Cursor X"=w679, "Cursor.Cursor Y"=w681) -> ()  [unwired: 2 in, 2 out]
                n229 = Select(t=u32 16723242, s=w667, f=u32 14745528) -> (s? t:f=w683:u32)
                n230 = local write "max frame rate (Hz)"(w668) -> ()
                n231 = Unbundle By Name(w694) -> ("X min"=w695:dbl, "Y min"=w696:dbl, "X max"=w697:dbl, "Y max"=w698:dbl)
                n232 = property on="Image" class="IntGraph (strict)"("Active Cursor"=u32 1, "Cursor.Cursor X"=w676, "Cursor.Cursor Y"=w677) -> ()  [unwired: 2 in, 2 out]
                n233 = property on="max frame rate (Hz)" class="DigNum (strict)"("NumText.BGColor"=w683) -> ()  [unwired: 2 in, 2 out]
                n234 = local write "Location indicator"(w699) -> ()
                n235 = property on="Image" class="IntGraph (strict)"("XScale.Minimum"=w695, "YScale.Minimum"=w696, "XScale.Maximum"=w697, "YScale.Maximum"=w698) -> ()  [unwired: 2 in, 2 out]
              }
            }
            n236 = local read "Live"() -> (w587:bool)
            n237 = case shown="True" w587 {
              tunnel: w591 -> [w609 w614]
              tunnel: w590 -> [w608 w613]
              tunnel: [w608 w612] -> w589
              tunnel: [w609 w611] -> w588
              tunnel: [T16 {"width"=0, "height"=0, "datatype"=0} ("Buffer") w610] -> w586
              frame False {
              }
              frame True {
                w615 = 1 items=["Snap", "Sequence"] ("Capture mode")
                n238 = call <userlib>:"tm_preparecapture.vi"("error in (no error)"=w613, "Capture mode"=w615, "Handle in"=w614) -> ("error out"=w617:errorcluster, "Buffer"=w610:T16, "Handle out"=w616:u32)  [unwired: 5 in, 1 out]
                n239 = call <userlib>:"tm_startcapture_b.vi"("error in (no error)"=w617, "Handle in"=w616) -> ("error out"=w612:errorcluster, "Handle out"=w611:u32)  [unwired: 8 in]
              }
            }
          }
          event "Define ROI": Value Change {
            n240 = event-data() -> ()  [unwired: 1 in, 1 out]
            n241 = case shown="False" "Define ROI" {
              frame False {
                w704 = FALSE ("Visible")
                # "hide cursors from image graph"
                n242 = property on="Image" class="IntGraph (strict)"("Active Cursor"=u32 0, "Cursor.Visible"=w704) -> ()  [unwired: 2 in, 2 out]
                n243 = property on="Image" class="IntGraph (strict)"("Active Cursor"=u32 1, "Cursor.Visible"=w704) -> ()  [unwired: 2 in, 2 out]
              }
              frame True {
                w707 = TRUE ("Visible")
                # "initialize ROI cursor to\nthe current field of view"
                n244 = property on="Image" class="IntGraph (strict)"() -> ("XScale.Minimum"=w712:dbl, "YScale.Minimum"=w711:dbl, "XScale.Maximum"=w710:dbl, "YScale.Maximum"=w709:dbl)  [unwired: 2 in, 2 out]
                n245 = property on="Image" class="IntGraph (strict)"("Active Cursor"=u32 0, "Cursor.Visible"=w707, "Cursor.Cursor X"=w712, "Cursor.Cursor Y"=w711) -> ()  [unwired: 2 in, 2 out]
                n246 = property on="Image" class="IntGraph (strict)"("Active Cursor"=u32 1, "Cursor.Visible"=w707, "Cursor.Cursor X"=w710, "Cursor.Cursor Y"=w709) -> ()  [unwired: 2 in, 2 out]
              }
            }
          }
          event "Previous ROI": Value Change {
            w741 = 1 items=["BINNING"=1, "BITS PER CHANNEL"=2, "ACTIVE VIEW INDEX"=3, "CCD MODE"=4, "SENSOR MODE"=5, "READOUT MODE"=6, "EXPOSURE TIME"=7, "CONTRAST GAIN"=8, "CONTRAST OFFSET"=9, "LIGHT MODE"=10, "SENSITIVITY"=11, "WHITE BALANCE"=12, "PHOTON IMAGING MODE"=13, "HIGH DYNAMIC RANGE MODE"=14, "TRIGGER SOURCE"=15, "TRIGGER ACTIVE"=16, "TRIGGER MODE"=17, "TRIGGER POLARITY"=18, "TRIGGER GLOBAL EXPOSURE"=19, "FIRST TRIGGER BEHAVIOR"=20, "TRIGGER TIMES"=21, "OUTPUT TRIGGER POLARITY"=22, "OUTPUT TRIGGER DELAY"=23, "OUTPUT TRIGGER PERIOD"=24, "TEMPERATURE"=25, "TEMPERATURE TARGET"=26, "SENSOR COOLER FAN"=27, "MECHANICAL SHUTTER"=28, "BACK FOCUS POSITION"=29, "FRAMEBUNDLE MODE"=30, "FRAMEBUNDLE NUMBER"=31, "LINEBUNDLE HEIGHT"=32, "TRIGGER CONNECTOR"=33, "IMAGE PIXEL TYPE"=34] ("Parameter")
            w742 = u16 2 items=["Full ROI", "Central quad", "Custom ROI"] ("ROI selection")
            w735 = FALSE ("Update ROI")
            # "calculate frame rate\nbased on ROI"
            # "set new ROI"
            # "update location indicator"
            n247 = event-data() -> ()  [unwired: 1 in, 1 out]
            n248 = local read "Live"() -> (w722:bool)
            n249 = case shown="False" w722 {
              tunnel: [w762 w767] -> w720
              tunnel: [w763 w766] -> w721
              tunnel: w723 -> [w763 w765]
              tunnel: w724 -> [w762 w764]
              frame False {
              }
              frame True {
                n250 = call <userlib>:"tm_stopcapture.vi"("error in (no error)"=w764, "Handle in"=w765) -> ("error out"=w768:errorcluster, "Handle out"=w769:u32)  [unwired: 8 in]
                n251 = call <userlib>:"tm_unpreparecapture.vi"("error in (no error)"=w768, "Handle in"=w769) -> ("error out"=w767:errorcluster, "Handle out"=w766:u32)  [unwired: 8 in]
              }
            }
            n252 = local write "Define ROI"(w735) -> ()
            n253 = local write "Previous ROI"(w735) -> ()
            n254 = property on="Image" class="IntGraph (strict)"("Active Cursor"=u32 0, "Cursor.Visible"=w735) -> ()  [unwired: 2 in, 2 out]
            n255 = property on="Image" class="IntGraph (strict)"("Active Cursor"=u32 1, "Cursor.Visible"=w735) -> ()  [unwired: 2 in, 2 out]
            n256 = local write "ROI selection"(w742) -> ()
            n257 = stacked-sequence {
              seq-local: [w771 _ _] -> [_ _ w775]
              seq-local: [w770 _ _] -> [_ _ w774]
              tunnel: [_ w773 _] -> w728
              tunnel: [_ w772 _] -> w727
              frame #0 {
                n258 = local read "Bin (n x n)"() -> (w770:u16)
                n259 = local read "ROI"() -> (w771:T1)
              }
              frame #1 {
                n260 = local read "Previous ROI"() -> (w773:T1)
                n261 = local read "Previous Bin"() -> (w772:u16)
                n262 = local write "ROI"(w773) -> ()
                n263 = local write "Bin (n x n)"(w772) -> ()
              }
              frame #2 {
                n264 = local write "Previous ROI"(w775) -> ()
                n265 = local write "Previous Bin"(w774) -> ()
              }
            }
            n266 = local read "x pixels"() -> (w736:i32)
            n267 = local read "cam frame\nrate (Hz)"() -> (w731:dbl[])
            n268 = local read "Measurements"() -> (w729:T12)
            n269 = Divide(x=w736, y=w727) -> (x/y=w730:dbl)
            n270 = call <userlib>:"tm_setparameter.vi"("error in (no error)"=w720, "Value in"=w727, "Parameter"=w741, "Handle in"=w721) -> ("error out"=w740:errorcluster, "Handle out"=w739:u32)  [unwired: 6 in]
            n271 = call "subUpdateLocIndicator_NW348.vi"("ROI"=w728, "pixel range"=w730) -> ("Graph scale"=w744:T21, "Location indicator"=w749:u16[][])  [unwired: 8 in]
            n272 = call "subImageROI2CameraROI_NW348.vi"("image ROI"=w728) -> ("camera ROI"=w743:T1)
            n273 = call "subGetMaxCameraRate_NW384.vi"("measure bool cluster"=w729, "cam frame\nrate (Hz)"=w731, "Bin (n x n)"=w727, "ROI"=w728, "Binned pixels"=w730) -> ("max frame rate (Hz)"=w725:dbl, "ROI too large"=w726:bool)  [unwired: 5 in]
            n274 = local write "max frame rate (Hz)"(w725) -> ()
            n275 = Select(t=u32 16723242, s=w726, f=u32 14745528) -> (s? t:f=w732:u32)
            n276 = call <userlib>:"tm_setarea.vi"("error in (no error)"=w740, "Sub Region"=w743, "Handle in"=w739) -> ("error out"=w717:errorcluster, "Handle out"=w719:u32)  [unwired: 7 in]
            n277 = local write "Location indicator"(w749) -> ()
            n278 = Unbundle By Name(w744) -> ("X min"=w745:dbl, "Y min"=w746:dbl, "X max"=w747:dbl, "Y max"=w748:dbl)
            n279 = property on="max frame rate (Hz)" class="DigNum (strict)"("NumText.BGColor"=w732) -> ()  [unwired: 2 in, 2 out]
            n280 = property on="Image" class="IntGraph (strict)"("XScale.Minimum"=w745, "YScale.Minimum"=w746, "XScale.Maximum"=w747, "YScale.Maximum"=w748) -> ()  [unwired: 2 in, 2 out]
            n281 = local read "Live"() -> (w714:bool)
            n282 = Wait (ms)(milliseconds to wait=u32 200) -> ()  [unwired: 1 out]
            n283 = case shown="False" w714 {
              tunnel: w719 -> [w753 w758]
              tunnel: w717 -> [w752 w757]
              tunnel: [w752 w756] -> w716
              tunnel: [w753 w755] -> w715
              tunnel: [T16 {"width"=0, "height"=0, "datatype"=0} ("Buffer") w754] -> w718
              frame False {
              }
              frame True {
                w759 = 1 items=["Snap", "Sequence"] ("Capture mode")
                n284 = call <userlib>:"tm_preparecapture.vi"("error in (no error)"=w757, "Capture mode"=w759, "Handle in"=w758) -> ("error out"=w761:errorcluster, "Buffer"=w754:T16, "Handle out"=w760:u32)  [unwired: 5 in, 1 out]
                n285 = call <userlib>:"tm_startcapture_b.vi"("error in (no error)"=w761, "Handle in"=w760) -> ("error out"=w756:errorcluster, "Handle out"=w755:u32)  [unwired: 8 in]
              }
            }
          }
          event "Live": Value Change {
            n286 = event-data() -> ()  [unwired: 1 in, 1 out]
            n287 = case shown="False" "Live" {
              tunnel: w782 -> [w787 w791]
              tunnel: w781 -> [w785 w792]
              tunnel: [w786 w796] -> w780
              tunnel: [w783 w795] -> w779
              tunnel: [w784 w794] -> w778
              tunnel: w776 -> [w784 _]
              frame False {
                n288 = local write "Status"("Ready" ("Status")) -> ()
                n289 = call <userlib>:"tm_stopcapture.vi"("error in (no error)"=w787, "Handle in"=w785) -> ("error out"=w788:errorcluster, "Handle out"=w789:u32)  [unwired: 8 in]
                n290 = call <userlib>:"tm_unpreparecapture.vi"("error in (no error)"=w788, "Handle in"=w789) -> ("error out"=w786:errorcluster, "Handle out"=w783:u32)  [unwired: 8 in]
              }
              frame True {
                w799 = 1 items=["Snap", "Sequence"] ("Capture mode")
                n291 = local write "Status"("Focusing" ("Status")) -> ()
                n292 = call <userlib>:"tm_preparecapture.vi"("error in (no error)"=w791, "Capture mode"=w799, "Handle in"=w792) -> ("error out"=w798:errorcluster, "Buffer"=w794:T16, "Handle out"=w797:u32)  [unwired: 5 in, 1 out]
                n293 = call <userlib>:"tm_startcapture_b.vi"("error in (no error)"=w798, "Handle in"=w797) -> ("error out"=w796:errorcluster, "Handle out"=w795:u32)  [unwired: 8 in]
              }
            }
          }
          event "Snap&Save": Value Change {
            w800 = bool[] [FALSE, FALSE, FALSE, FALSE, FALSE, FALSE]
            # "Turn off all lasers AOTF"
            # "Turn off 447 laser"
            n294 = event-data() -> ()  [unwired: 1 in, 1 out]
            n295 = local read "Live"() -> (w854:bool)
            n296 = local read "Exposure (msec)"() -> (w804:dbl)
            n297 = case shown="True" w854 {
              tunnel: [w874 w877] -> w808
              tunnel: w856 -> [w874 w876]
              tunnel: w855 -> [_ w875]
              frame False {
              }
              frame True {
                n298 = call <userlib>:"tm_stopcapture.vi"("error in (no error)"=w876, "Handle in"=w875) -> ("error out"=w878:errorcluster, "Handle out"=w879:u32)  [unwired: 8 in]
                n299 = call <userlib>:"tm_unpreparecapture.vi"("error in (no error)"=w878, "Handle in"=w879) -> ("error out"=w877:errorcluster)  [unwired: 8 in, 1 out]
              }
            }
            n300 = local read "ROI"() -> (w805:T1)
            n301 = Bundle("ROI"=w805, "Exposure (msec)"=w804, 1) -> (w810:T31)  [unwired: 1 in]
            n302 = local read "Bin (n x n)"() -> (w803:u16)
            n303 = local read "cam frame\nrate (Hz)"() -> (w837:dbl[])
            n304 = local read "x pixels"() -> (w802:i32)
            n305 = call "subSnapshot_NW348.vi"("Error in"=w808, "Camera info"=w810) -> ("Error out"=w807:errorcluster, "Image"=w806:u16[][])  [unwired: 8 in]
            n306 = Divide(x=w802, y=w803) -> (x/y=w801:dbl)
            n307 = local read "Camera mode"() -> (w842:u16)
            n308 = Reciprocal(x=w837) -> (1/x=w838:dbl[])
            n309 = Divide(x=w804, y=1000.0 ("milliseconds to wait")) -> (x/y=w840:dbl)
            n310 = local read "AOTF digital lines"() -> (w848:T5)
            n311 = call "subPadImage_NW348.vi"("ROI"=w805, "Full size"=w801, "Image in"=w806) -> ("image info"=w845:T22, "Image out"=w844:u16[][])  [unwired: 7 in]
            n312 = Build Array (concatenate)(w840, w838) -> (w841:dbl[])
            n313 = local write "Image"(w844) -> ()
            n314 = local write "Image info"(w845) -> ()
            n315 = local read "AO ports"() -> (w835:T7)
            n316 = Index Array(array=w841, index=w842) -> (element=w846:dbl)
            n317 = local read "AOTF efficiency"() -> (w813:dbl[])
            n318 = local read "Emission filter"() -> (w824:u16)
            n319 = local read "AOTF\ndigital"() -> (w820:bool[])
            n320 = Cluster To Array(cluster=w848) -> (array=w849:tag[])
            n321 = local read "447nm"() -> (w819:bool)
            n322 = local write "AOTF\ndigital"(w800) -> ()
            n323 = Unbundle By Name(w835) -> ("447nm laser"=w836:tag)
            n324 = call "subSetDigStates_NW348.vi"("Error in (no error)"=w807, "Digital line array"=w849, "Digital state array"=w800) -> ("Error out"=w834:errorcluster)  [unwired: 8 in]
            n325 = Multiply(x=1000.0 ("y"), y=w846) -> (x*y=w818:dbl)
            n326 = Build Array (concatenate)(w813, 1.0 ("y")) -> (w822:dbl[])
            n327 = local read "Bin (n x n)"() -> (w817:u16)
            n328 = Build Array(w818) -> (w843:dbl[])
            n329 = Build Array (concatenate)(w820, w819) -> (w821:bool[])
            n330 = call-poly <vilib>:"DAQmx Create Virtual Channel.vi"("maximum value"=5.0, "minimum value"=-5.0, "physical channels"=w836, "error in"=w834) -> ("task out"=w828:refnum<k21>, "error out"=w829:errorcluster)  [unwired: 5 in, 5 out]
            n331 = call "subAcquisitionInfo_NW348.vi"("Emission filter"=w824, "Bin (n x n)"=w817, "AOTF digital"=w821, "Channel names"="AOTF channels", "Efficiency"=w822, "Exposure time (msec)"=w843) -> ("Text"=w815:string)  [unwired: 4 in, 1 out]
            n332 = call <vilib>:"DAQmx Start Task.vi"("task/channels in"=w828, "error in"=w829) -> ("task out"=w827:refnum<k21>, "error out"=w826:errorcluster)  [unwired: 12 out]
            n333 = local read "base path"() -> (w811:path)
            n334 = call-poly <vilib>:"DAQmx Write.vi"("task/channels in"=w827, "data"=0.0 ("minimum value"), "error in"=w826) -> ("task out"=w833:refnum<k21>, "error out"=w832:errorcluster)  [unwired: 1 in, 10 out]
            n335 = call <vilib>:"DAQmx Clear Task.vi"("task in"=w833, "error in"=w832) -> ("error out"=w816:errorcluster)  [unwired: 13 out]
            n336 = flat-sequence {
              tunnel: w815 -> [w863]
              tunnel: w816 -> [w862]
              tunnel: w811 -> [w860]
              tunnel: w806 -> [w859]
              tunnel: [w858] -> w812
              frame #0 {
                w861 = TRUE ("Snap&Save")
                n337 = local write "Snap&Save"(FALSE ("Snap&Save")) -> ()
                n338 = call "subSaveAsTiff_NW348.vi"("Open file dialog? (F)"=w861, "Save Text file? (F)"=w861, "Error in (no error)"=w862, "text"=w863, "File path/name"=w860, "Image"=w859) -> ("Error out"=w858:errorcluster)  [unwired: 5 in]
              }
            }
            n339 = local read "Live"() -> (w851:bool)
            n340 = case shown="False" w851 {
              tunnel: w812 -> [w866 w870]
              tunnel: [w866 w869] -> w853
              tunnel: [u32 0 ("Handle out") w868] -> w852
              tunnel: [T16 {"width"=0, "height"=0, "datatype"=0} ("Buffer") w867] -> w850
              frame False {
              }
              frame True {
                w871 = 1 items=["Snap", "Sequence"] ("Capture mode")
                n341 = call <userlib>:"tm_preparecapture.vi"("error in (no error)"=w870, "Capture mode"=w871) -> ("error out"=w873:errorcluster, "Buffer"=w867:T16, "Handle out"=w872:u32)  [unwired: 6 in, 1 out]
                n342 = call <userlib>:"tm_startcapture_b.vi"("error in (no error)"=w873, "Handle in"=w872) -> ("error out"=w869:errorcluster, "Handle out"=w868:u32)  [unwired: 8 in]
              }
            }
          }
          event "Acquire movie": Value Change {
            w885 = bool[] [FALSE, FALSE, FALSE, FALSE, FALSE, FALSE]
            w914 = 1 items=["Snap", "Sequence"] ("Capture mode")
            # "Turn off all lasers AOTF"
            n343 = event-data() -> ()  [unwired: 1 in, 5 out]
            n344 = flat-sequence {
              tunnel: [w932] -> w890
              frame #0 {
                n345 = Get Date/Time In Seconds() -> (seconds since 1Jan1904=w925:timestamp)
                n346 = Format Date/Time String(time format string (%c)="_at%H%M%S", seconds (now)=w925) -> (date/time string=w924:string)  [unwired: 1 in]
                n347 = local read "base path"() -> (w929:path)
                n348 = local write "Status"("Acquiring movie" ("Status")) -> ()
                n349 = Concatenate Strings("Movie name", w924, ".dcimg" ("string")) -> (w930:string)
                n350 = Build Path(base path=w929, name or relative path=w930) -> (appended path=w932:path)
              }
            }
            n351 = local read "Live"() -> (w896:bool)
            n352 = case shown="True" w896 {
              tunnel: [w944 w948] -> w893
              tunnel: w894 -> [w944 w947]
              tunnel: w895 -> [w943 w946]
              tunnel: [w943 w945] -> w892
              frame False {
              }
              frame True {
                n353 = call <userlib>:"tm_stopcapture.vi"("error in (no error)"=w947, "Handle in"=w946) -> ("error out"=w949:errorcluster, "Handle out"=w950:u32)  [unwired: 8 in]
                n354 = call <userlib>:"tm_unpreparecapture.vi"("error in (no error)"=w949, "Handle in"=w950) -> ("error out"=w948:errorcluster, "Handle out"=w945:u32)  [unwired: 8 in]
              }
            }
            n355 = local read "# frames"() -> (w901:u32)
            n356 = call <userlib>:"tm_preparecapture.vi"("error in (no error)"=w893, "Capture mode"=w914, "Handle in"=w892) -> ("error out"=w913:errorcluster, "Handle out"=w912:u32)  [unwired: 5 in, 2 out]
            n357 = call <userlib>:"tm_startrecorder.vi"("error in (no error)"=w913, "frames"=w901, "File"=w890, "Handle in"=w912) -> ("error out"=w911:errorcluster, "Handle out"=w910:u32)  [unwired: 6 in]
            n358 = Tick Count (ms)() -> (millisecond timer value=w880:u32)
            n359 = call <userlib>:"tm_startcapture_b.vi"("error in (no error)"=w911, "Handle in"=w910) -> ("error out"=w909:errorcluster, "Handle out"=w908:u32)  [unwired: 8 in]
            n360 = case shown="No Error" w909 {
              selector: w909 -> [w956 w970]
              tunnel: w908 -> [w955 w971]
              tunnel: [w953 w971] -> w902
              tunnel: [w954 w970] -> w903
              tunnel: w901 -> [w952 _]
              tunnel: w880 -> [w951 _]
              frame No Error {
                n361 = while {
                  tunnel: w956 -> [w967]
                  tunnel: w955 -> [w966]
                  tunnel: [w965] -> w954
                  tunnel: [w968] -> w953
                  tunnel: w952 -> [w969]
                  tunnel: w951 -> [w960]
                  stop <- w963 stop-if-true
                  n362 = Tick Count (ms)() -> (millisecond timer value=w959:u32)
                  n363 = Wait (ms)(milliseconds to wait=u32 100) -> ()  [unwired: 1 out]
                  n364 = Subtract(x=w959, y=w960) -> (x-y=w958:u32)
                  n365 = call <userlib>:"tm_getrecorderstatus.vi"("error in (no error)"=w967, "Handle"=w966) -> ("error out"=w965:errorcluster, "Count"=w964:i32, "Handle"=w968:u32)  [unwired: 6 in, 1 out]
                  "Frames Recorded" <- w964
                  n366 = Divide(x=w958, y=1000.0) -> (x/y=→"Elapsed time (sec)":dbl)
                  n367 = Greater Or Equal?(x=w964, y=w969) -> (x >= y?=w963:bool)
                }
              }
              frame Error {
              }
            }
            n368 = call <userlib>:"tm_stoprecorder.vi"("error in (no error)"=w903, "Handle in"=w902) -> ("error out"=w904:errorcluster, "Handle out"=w905:u32)  [unwired: 8 in]
            n369 = local read "AOTF digital lines"() -> (w899:T5)
            n370 = call <userlib>:"tm_stopcapture.vi"("error in (no error)"=w904, "Handle in"=w905) -> ("error out"=w907:errorcluster, "Handle out"=w906:u32)  [unwired: 8 in]
            n371 = call <userlib>:"tm_unpreparecapture.vi"("error in (no error)"=w907, "Handle in"=w906) -> ("error out"=w898:errorcluster)  [unwired: 8 in, 1 out]
            n372 = Cluster To Array(cluster=w899) -> (array=w900:tag[])
            n373 = flat-sequence {
              tunnel: w885 -> [w923]
              tunnel: w900 -> [w922]
              tunnel: w898 -> [w921]
              tunnel: [w920] -> w897
              frame #0 {
                n374 = local write "Status"("Saving binary file" ("Status")) -> ()
                n375 = call "subSetDigStates_NW348.vi"("Error in (no error)"=w921, "Digital line array"=w922, "Digital state array"=w923) -> ("Error out"=w920:errorcluster)  [unwired: 8 in]
              }
            }
            n376 = local write "AOTF\ndigital"(w885) -> ()
            n377 = call "subSaveAsBin_NW348.vi"("Delete .dcimg?"=TRUE, "Save Text file?"=FALSE, "Error in"=w897, ".dcimg file name"=w890) -> ("Error out"=w889:errorcluster)  [unwired: 7 in]
            n378 = local read "Live"() -> (w891:bool)
            n379 = case shown="True" w891 {
              tunnel: w889 -> [w935 w939]
              tunnel: [w935 w938] -> w883
              tunnel: [u32 0 ("Handle out") w937] -> w884
              tunnel: [T16 {"width"=0, "height"=0, "datatype"=0} ("Buffer") w936] -> w888
              frame False {
              }
              frame True {
                w940 = 1 items=["Snap", "Sequence"] ("Capture mode")
                n380 = call <userlib>:"tm_preparecapture.vi"("error in (no error)"=w939, "Capture mode"=w940) -> ("error out"=w942:errorcluster, "Buffer"=w936:T16, "Handle out"=w941:u32)  [unwired: 6 in, 1 out]
                n381 = call <userlib>:"tm_startcapture_b.vi"("error in (no error)"=w942, "Handle in"=w941) -> ("error out"=w938:errorcluster, "Handle out"=w937:u32)  [unwired: 8 in]
              }
            }
            n382 = flat-sequence {
              tunnel: w884 -> [w917]
              tunnel: w883 -> [w918]
              tunnel: [w918] -> w882
              tunnel: [w917] -> w881
              frame #0 {
                n383 = local write "Acquire movie"(FALSE ("Acquire movie")) -> ()
                n384 = local write "Status"("ready" ("Status")) -> ()
              }
            }
          }
          event "# frames": Value Change {
            n385 = event-data() -> ()  [unwired: 1 in, 1 out]
            n386 = local read "Exposure (msec)"() -> (w975:dbl)
            n387 = Multiply(x="# frames", y=w975) -> (x*y=w974:dbl)
            n388 = Divide(x=w974, y=1000.0) -> (x/y=w972:dbl)
            n389 = local write "Total time (sec)"(w972) -> ()
          }
          event "Total time (sec)": Value Change {
            n390 = event-data() -> ()  [unwired: 1 in, 5 out]
            n391 = local read "Exposure (msec)"() -> (w987:dbl)
            n392 = Multiply(x=1000.0 ("y"), y="Total time (sec)") -> (x*y=w983:dbl)
            n393 = Divide(x=w983, y=w987) -> (x/y=w988:dbl)
            n394 = Round To Nearest(number=w988) -> (nearest integer value=w986:dbl)
            n395 = local write "# frames"(w986) -> ()
            n396 = Multiply(x=w986, y=w987) -> (x*y=w981:dbl)
            n397 = Divide(x=w981, y=1000.0) -> (x/y=w980:dbl)
            n398 = local write "Total time (sec)"(w980) -> ()
          }
          event "Start acquisition": Value Change {
            # "Memory and Absolute V digital outs\ncamera, lasers, global shutter"
            n399 = event-data() -> ()  [unwired: 1 in, 1 out]
            n400 = local read "AOTF digital lines"() -> (w1012:T5)
            n401 = local read "laser bool array"() -> (w995:bool[])
            n402 = local read "Bin (n x n)"() -> (w1022:u16)
            n403 = local read "cam frame\nrate (Hz)"() -> (w1026:dbl[])
            n404 = local read "x pixels"() -> (w1023:i32)
            n405 = local read "Measurements"() -> (w1025:T12)
            n406 = local read "Shutter lines"() -> (w1018:T4)
            n407 = local read "ROI"() -> (w1024:T1)
            n408 = local read "AOTF digital lines"() -> (w1019:T5)
            n409 = Divide(x=w1023, y=w1022) -> (x/y=w1021:dbl)
            n410 = local read "AO ports"() -> (w1011:T7)
            n411 = Build Array("Camera trigger") -> (w1014:tag[])
            n412 = Cluster To Array(cluster=w1012) -> (array=w1010:tag[])
            n413 = Boolean To (0,1)(Boolean=w995) -> (0, 1=w996:i16[])
            n414 = local read "Camera trigger"() -> (w1016:tag)
            n415 = for {
              N: 5 -> [_]
              tunnel: w995 -> [w1030] mode=indexing
              tunnel: w1010 -> [w1028] mode=indexing
              shift-right: [w1027] -> w1005
              shift-left: w1014 -> [w1029]
              n416 = case shown="True" w1030 {
                tunnel: w1029 -> [w1031 w1034]
                tunnel: w1028 -> [_ w1032]
                tunnel: [w1031 w1033] -> w1027
                frame False {
                }
                frame True {
                  n417 = Build Array (concatenate)(w1034, w1032) -> (w1033:tag[])
                }
              }
            }
            n418 = Add Array Elements(numeric array=w996) -> (sum=w994:i16)
            n419 = call "subGetMaxCameraRate_NW384.vi"("measure bool cluster"=w1025, "cam frame\nrate (Hz)"=w1026, "Bin (n x n)"=w1022, "ROI"=w1024, "Binned pixels"=w1021) -> ("ROI too large"=w1020:bool)  [unwired: 5 in, 1 out]
            n420 = Unbundle By Name(w1018) -> ("shutter Global"=w1015:tag)
            n421 = Unbundle By Name(w1011) -> ("AO A-M External"=w1004:tag)
            n422 = Cluster To Array(cluster=w1019) -> (array=w1017:tag[])
            n423 = local read "Simultaneous"() -> (w993:bool)
            n424 = Cluster To Array(cluster="AI ports") -> (array=w1003:tag[])
            n425 = Build Array (concatenate)(w1016, w1017, w1015) -> (w1002:tag[])
            n426 = case shown="False" w1020 {
              tunnel: "Measurements" -> [w1047 _]
              tunnel: "DI camera fire" -> [w1046 _]
              tunnel: w1005 -> [w1045 _]
              tunnel: w1004 -> [w1044 _]
              tunnel: w1003 -> [w1043 _]
              tunnel: w1002 -> [w1042 _]
              tunnel: w1001 -> [w1037 w1457]
              tunnel: w1000 -> [w1038 w1458]
              tunnel: [w1041 w1455] -> w999
              tunnel: [w1040 w1458] -> w998
              tunnel: [w1039 w1457] -> w997
              tunnel: w994 -> [w1036 _]
              tunnel: w993 -> [w1035 _]
              tunnel: w992 -> [_ w1455]
              frame False {
                n427 = stacked-sequence {
                  tunnel: w1043 -> [_ _ w1187 w1234 w1286 w1332 w1377 _]
                  tunnel: w1047 -> [w1082 w1132 w1186 w1239 w1291 w1336 w1381 _]
                  tunnel: w1045 -> [_ _ w1184 w1236 w1288 _ _ _]
                  tunnel: w1044 -> [_ _ w1183 w1235 w1287 w1333 w1378 _]
                  tunnel: w1046 -> [_ _ w1182 w1237 w1289 w1334 w1379 _]
                  tunnel: w1042 -> [_ _ _ _ _ w1331 w1376 _]
                  tunnel: [_ _ _ _ _ _ _ w1438] -> w1041
                  tunnel: [_ _ _ _ _ _ _ w1439] -> w1040
                  tunnel: [_ _ _ _ _ _ _ w1440] -> w1039
                  tunnel: w1038 -> [w1050 _ _ _ _ _ _ w1435]
                  tunnel: w1037 -> [w1049 _ _ _ _ _ _ _]
                  tunnel: w1036 -> [_ _ w1181 w1233 w1285 _ _ _]
                  tunnel: w1035 -> [_ _ w1180 w1232 w1284 _ _ _]
                  frame #0 {
                    # "1. Create folder name with current time.\n2. Save notes as a text file.\n3. Save experimental parameters in tab-delimited text file."
                    n428 = Cluster To Array(cluster=w1082) -> (array=w1077:bool[])
                    n429 = local read "Live"() -> (w1051:bool)
                    n430 = for {
                      N: 5 -> [_]
                      tunnel: w1077 -> [w1118] mode=indexing
                      tunnel: string[] ["S", "T", "L", "M", "A"] -> [w1117] mode=indexing
                      shift-right: [w1116] -> w1079
                      shift-left: "_" -> [w1115]
                      n431 = case shown="True" w1118 {
                        tunnel: w1117 -> [_ w1120]
                        tunnel: [w1119 w1121] -> w1116
                        tunnel: w1115 -> [w1119 w1122]
                        frame False {
                        }
                        frame True {
                          n432 = Concatenate Strings(w1122, w1120) -> (w1121:string)
                        }
                      }
                    }
                    n433 = case shown="False" w1051 {
                      tunnel: [w1083 w1086] -> w1048
                      tunnel: w1049 -> [w1083 w1085]
                      tunnel: w1050 -> [_ w1084]
                      frame False {
                      }
                      frame True {
                        n434 = call <userlib>:"tm_stopcapture.vi"("error in (no error)"=w1085, "Handle in"=w1084) -> ("error out"=w1087:errorcluster, "Handle out"=w1088:u32)  [unwired: 8 in]
                        n435 = call <userlib>:"tm_unpreparecapture.vi"("error in (no error)"=w1087, "Handle in"=w1088) -> ("error out"=w1086:errorcluster)  [unwired: 8 in, 1 out]
                      }
                    }
                    n436 = Get Date/Time In Seconds() -> (seconds since 1Jan1904=w1073:timestamp)
                    n437 = Format Date/Time String(time format string (%c)="%H%M%S", seconds (now)=w1073) -> (date/time string=w1075:string)  [unwired: 1 in]
                    n438 = local write "Error"(w1048) -> ()
                    n439 = Concatenate Strings(w1075, w1079, "_", "appended folder name") -> (w1067:string)
                    n440 = Build Path(base path="base path", name or relative path=w1067) -> (appended path=w1068:path)
                    n441 = local read "Square setting"() -> (w1064:T8)
                    n442 = local read "Triangle setting"() -> (w1060:T9)
                    n443 = local read "Pump setting"() -> (w1059:T11)
                    n444 = Create Folder(path (use dialog)=w1068) -> (created path=w1066:path)  [unwired: 2 in, 2 out]
                    "full path" <- w1066
                    n445 = Build Path(base path=w1066, name or relative path="notes.txt") -> (appended path=w1072:path)
                    n446 = Unbundle By Name(w1064) -> ("Voltage freq. (Hz)"=w1063:dbl, "# cycles per color"=w1062:u32, "# spect. cycles"=w1061:u32)
                    n447 = Unbundle By Name(w1060) -> ("Voltage freq. (Hz)"=w1058:dbl, "# cycles per color"=w1057:u32, "# spect. cycles"=w1056:u32)
                    n448 = Unbundle By Name(w1059) -> ("Laser freq. (Hz)"=w1055:dbl, "# cycles per color"=w1054:u32, "# spect. cycles"=w1053:u32)
                    n449 = Write to Text File(file (use dialog)=w1072, text="Notes") -> ()  [unwired: 2 in, 3 out]
                    n450 = case shown="True" "SAVE" {
                      tunnel: w1066 -> [_ w1098]
                      tunnel: w1063 -> [_ w1097]
                      tunnel: w1062 -> [_ w1096]
                      tunnel: w1061 -> [_ w1095]
                      tunnel: w1058 -> [_ w1094]
                      tunnel: w1057 -> [_ w1093]
                      tunnel: w1056 -> [_ w1092]
                      tunnel: w1055 -> [_ w1091]
                      tunnel: w1054 -> [_ w1090]
                      tunnel: w1053 -> [_ w1089]
                      frame False {
                      }
                      frame True {
                        n451 = local read "cam frame\nrate (Hz)"() -> (w1101:dbl[])
                        n452 = local read "DAQ sampling rate"() -> (w1109:dbl)
                        n453 = local read "AOTF efficiency"() -> (w1113:dbl[])
                        n454 = local read "laser bool array"() -> (w1110:bool[])
                        n455 = local read "# cam\nframes"() -> (w1103:i32[])
                        n456 = local read "Measurements"() -> (w1114:T12)
                        n457 = local read "Simultaneous"() -> (w1112:bool)
                        n458 = local read "ROI"() -> (w1104:T1)
                        n459 = Bundle("Voltage freq. (Hz)"=w1097, "# cycles per color"=w1096, "# spect. cycles"=w1095) -> (w1105:T32)  [unwired: 1 in]
                        n460 = Bundle("Voltage freq. (Hz)"=w1094, "# cycles per color"=w1093, "# spect. cycles"=w1092) -> (w1106:T32)  [unwired: 1 in]
                        n461 = Bundle("Laser freq. (Hz)"=w1091, "# cycles per color"=w1090, "# spect. cycles"=w1089) -> (w1107:T33)  [unwired: 1 in]
                        n462 = Bundle("cam frame\nrate (Hz)"=w1101, "# cam\nframes"=w1103, "ROI"=w1104) -> (w1102:T34)  [unwired: 1 in]
                        n463 = Build Path(base path=w1098, name or relative path="experimental_parameters.txt") -> (appended path=w1100:path)
                        n464 = Bundle(w1105, w1106, w1107, "DAQ sampling rate"=w1109) -> (w1108:T35)  [unwired: 1 in]
                        n465 = Bundle("Measurements"=w1114, "laser bool array"=w1110, "Simultaneous"=w1112, "AOTF efficiency"=w1113) -> (w1111:T36)  [unwired: 1 in]
                        n466 = call "subSaveExptParams_NW348.vi"("Path"=w1100, "Recording params"=w1111, "DAQ params"=w1108, "Camera params"=w1102) -> ()  [unwired: 7 in, 1 out]
                      }
                    }
                  }
                  frame #1 {
                    # "frames to average"
                    # "Background measurement"
                    n467 = local read "Triangle setting"() -> (w1130:T9)
                    n468 = local read "Square setting"() -> (w1131:T8)
                    n469 = Unbundle By Name(w1132) -> ("Square wave"=w1136:bool, "Triangle wave"=w1135:bool, "Memory"=w1134:bool, "Absolute Voltage"=w1133:bool)
                    n470 = local read "AOTF digital lines"() -> (w1126:T5)
                    n471 = local read "Cam frame rate (Hz)\nAbs V"() -> (w1140:dbl)
                    n472 = local read "Cam frame rate (Hz)\nMem"() -> (w1141:dbl)
                    n473 = Unbundle By Name(w1130) -> ("Frame rate (Hz)"=w1128:dbl)
                    n474 = Unbundle By Name(w1131) -> ("Frame rate (Hz)"=w1129:dbl)
                    n475 = local read "Error"() -> (w1124:errorcluster)
                    n476 = Build Array(w1136, w1135, w1134, w1133) -> (w1143:bool[])
                    n477 = Cluster To Array(cluster=w1126) -> (array=w1125:tag[])
                    n478 = call "subSetDigStates_NW348.vi"("Error in (no error)"=w1124, "Digital line array"=w1125, "Digital state array"=bool[] [FALSE, FALSE, FALSE, FALSE, FALSE, FALSE] ("Laser digital state array")) -> ("Error out"=w1123:errorcluster)  [unwired: 8 in]
                    n479 = Build Array(w1129, w1128, w1141, w1140) -> (w1139:dbl[])
                    n480 = for {
                      N: 4 -> [_]
                      tunnel: w1143 -> [w1150] mode=indexing
                      tunnel: string[] ["Square wave ", "Triangle wave", "Memory", "Absolute voltage"] -> [w1149] mode=indexing
                      tunnel: w1139 -> [w1148] mode=indexing
                      shift-right: [w1146] -> w1138
                      shift-left: w1123 -> [w1147]
                      tunnel: i32[] [100, 10, 20, 20] -> [w1145] mode=indexing
                      n481 = case shown="True" w1150 {
                        tunnel: w1149 -> [_ w1173]
                        tunnel: w1148 -> [_ w1172]
                        tunnel: w1147 -> [w1151 w1163]
                        tunnel: [w1151 w1158] -> w1146
                        tunnel: w1145 -> [_ w1166]
                        frame False {
                        }
                        frame True {
                          w1168 = u16 1 items=["Amplitude", "Efficiency"] ("Input type")
                          n482 = Reciprocal(x=w1172) -> (1/x=w1161:dbl)
                          n483 = local read "AOTF efficiency"() -> (w1167:dbl[])
                          n484 = local read "AOTF info"() -> (w1169:T3)
                          n485 = local read "ROI"() -> (w1165:T1)
                          n486 = Multiply(x=w1161, y=1000.0) -> (x*y=w1162:dbl)
                          n487 = local read "full path"() -> (w1157:path)
                          n488 = Concatenate Strings("Bkgnd_" ("Status"), w1173, ".tiff" ("Status")) -> (w1174:string)
                          n489 = Bundle("ROI"=w1165, w1162, w1166) -> (w1164:T37)  [unwired: 1 in]
                          n490 = call "subAOTFamplitude_6channels_NW348.vi"("AOTF info"=w1169, "Input type"=w1168, "Error in"=w1163, "Efficiency In"=w1167) -> ("Error out"=w1153:errorcluster)  [unwired: 5 in, 2 out]
                          n491 = Build Path(base path=w1157, name or relative path=w1174) -> (appended path=w1156:path)
                          n492 = call "subSnapshot_NW348.vi"("Error in"=w1153, "Camera info"=w1164) -> ("Error out"=w1159:errorcluster, "Image"=w1155:u16[][])  [unwired: 8 in]
                          n493 = local read "SAVE"() -> (w1154:bool)
                          n494 = case shown="True" w1154 {
                            tunnel: w1159 -> [w1175 w1179]
                            tunnel: [w1175 w1178] -> w1158
                            tunnel: w1156 -> [_ w1177]
                            tunnel: w1155 -> [_ w1176]
                            frame False {
                            }
                            frame True {
                              n495 = call "subSaveAsTiff_NW348.vi"("Error in (no error)"=w1179, "File path/name"=w1177, "Image"=w1176) -> ("Error out"=w1178:errorcluster)  [unwired: 8 in]
                            }
                          }
                          "Status" <- "background" ("Status")
                        }
                      }
                    }
                    n496 = local write "Error"(w1138) -> ()
                  }
                  frame #2 {
                    n497 = Unbundle By Name(w1186) -> ("Square wave"=w1185:bool)
                    n498 = case shown="True" w1185 {
                      tunnel: w1187 -> [_ w1203]
                      tunnel: w1184 -> [_ w1205]
                      tunnel: w1183 -> [_ w1204]
                      tunnel: w1182 -> [_ w1197]
                      tunnel: w1181 -> [_ w1189]
                      tunnel: w1180 -> [_ w1188]
                      frame False {
                      }
                      frame True {
                        n499 = local read "DAQ sampling rate"() -> (w1192:dbl)
                        n500 = Bundle("DI camera fire"=w1197, w1205, "AO A-M External"=w1204, "AI ports"=w1203) -> (w1202:T38)  [unwired: 1 in]
                        n501 = local read "Square setting"() -> (w1209:T8)
                        n502 = local read "full path"() -> (w1212:path)
                        n503 = local read "External"() -> (w1208:dbl)
                        n504 = local read "Error"() -> (w1196:errorcluster)
                        n505 = Build Path(base path=w1212, name or relative path="Sq_camera.dcimg") -> (appended path=w1199:path)
                        n506 = call "subGenerateSquareWaveform_NW348.vi"("num colors"=w1189, "Simultaneous"=w1188, "error in (no error)"=w1196, "Square wave settings"=w1209, "External"=w1208, "DAQ sampling rate"=w1192) -> ("error out"=w1195:errorcluster, "Info"=w1198:T18, "AO waveform"=w1201:waveform(dbl), "DO waveform"=w1200:digitalwaveform[])  [unwired: 2 out]
                        n507 = local write "Status"("Square wave: Acquiring .dcimg file" ("Status")) -> ()
                        n508 = Unbundle By Name(w1198) -> ("# cam. frames"=w1193:u32)
                        n509 = Reciprocal(x=w1192) -> (1/x=w1206:dbl)
                        n510 = call "subDataAcquisition_NW348.vi"("# cam.\nframes"=w1193, "DAQ sampling rate"=w1192, "Image file path"=w1199, "error in (no error)"=w1195, "DAQ ports"=w1202, "AO waveform"=w1201, "DO waveform"=w1200) -> ("error out"=w1191:errorcluster, "DI waveform"=w1215:digitalwaveform, "AI data"=w1214:dbl[][])  [unwired: 1 in, 1 out]
                        n511 = local read "SAVE"() -> (w1213:bool)
                        n512 = Bundle(0, w1206, "AI data"=w1214) -> (→"Waveform Graph":cluster{i32, dbl, "AI data":dbl[][]})  [unwired: 1 in]
                        n513 = case shown="True" w1213 {
                          tunnel: w1200 -> [_ w1230]
                          tunnel: w1201 -> [_ w1229]
                          tunnel: w1214 -> [_ w1223]
                          tunnel: w1215 -> [_ w1224]
                          tunnel: w1199 -> [_ w1221]
                          tunnel: w1191 -> [w1216 w1222]
                          tunnel: [w1216 w1218] -> w1194
                          frame False {
                          }
                          frame True {
                            n514 = local read "laser bool array"() -> (w1231:bool[])
                            n515 = local read "full path"() -> (w1225:path)
                            n516 = call "subSaveAsBin_NW348.vi"("Delete .dcimg?"=TRUE, "Save Text file?"=FALSE, "Error in"=w1222, ".dcimg file name"=w1221) -> ("Error out"=w1218:errorcluster)  [unwired: 7 in]
                            n517 = Build Path(base path=w1225, name or relative path="Sqrwave_DAQ.txt") -> (appended path=w1228:path)
                            n518 = local write "Status"("Square wave: Saving binary file" ("Status")) -> ()
                            n519 = call "subSaveDaqDataAI_DI_NW348.vi"("DI waveform"=w1224, "AI data"=w1223, "Square or \nTriangle wave"=TRUE ("Square or \nTriangle wave"), "AO sq"=w1229, "Square\ndig. waveform"=w1230, "laser bool\n array"=w1231, "path"=w1228) -> ()  [unwired: 5 in]
                          }
                        }
                        n520 = local write "Error"(w1194) -> ()
                      }
                    }
                  }
                  frame #3 {
                    n521 = Unbundle By Name(w1239) -> ("Triangle wave"=w1238:bool)
                    n522 = case shown="True" w1238 {
                      tunnel: w1234 -> [_ w1256]
                      tunnel: w1236 -> [_ w1258]
                      tunnel: w1235 -> [_ w1257]
                      tunnel: w1237 -> [_ w1253]
                      tunnel: w1233 -> [_ w1241]
                      tunnel: w1232 -> [_ w1240]
                      frame False {
                      }
                      frame True {
                        n523 = local read "DAQ sampling rate"() -> (w1250:dbl)
                        n524 = Bundle("DI camera fire"=w1253, w1258, "AO A-M External"=w1257, "AI ports"=w1256) -> (w1255:T38)  [unwired: 1 in]
                        n525 = local read "Triangle setting"() -> (w1248:T9)
                        n526 = local read "full path"() -> (w1264:path)
                        n527 = local read "External"() -> (w1249:dbl)
                        n528 = local read "Error"() -> (w1247:errorcluster)
                        n529 = Build Path(base path=w1264, name or relative path="Tri_camera.dcimg") -> (appended path=w1254:path)
                        n530 = call "subGenerateTriangleWaveform_NW348.vi"("num colors"=w1241, "Simultaneous"=w1240, "error in (no error)"=w1247, "Triangle wave settings"=w1248, "External"=w1249, "DAQ sampling rate"=w1250) -> ("error out"=w1244:errorcluster, "Triangle info"=w1243:T20, "AO tri"=w1245:waveform(dbl), "Triangle\ndig. waveform"=w1246:digitalwaveform[])  [unwired: 2 out]
                        n531 = local write "Status"("Triangle wave: Acquiring .dcimg file" ("Status")) -> ()
                        n532 = Unbundle By Name(w1243) -> ("# cam. frame"=w1251:u32)
                        n533 = Reciprocal(x=w1250) -> (1/x=w1259:dbl)
                        n534 = call "subDataAcquisition_NW348.vi"("# cam.\nframes"=w1251, "DAQ sampling rate"=w1250, "Image file path"=w1254, "error in (no error)"=w1244, "DAQ ports"=w1255, "AO waveform"=w1245, "DO waveform"=w1246) -> ("error out"=w1242:errorcluster, "DI waveform"=w1267:digitalwaveform, "AI data"=w1266:dbl[][])  [unwired: 1 in, 1 out]
                        n535 = local read "SAVE"() -> (w1265:bool)
                        n536 = Bundle(0, w1259, "AI data"=w1266) -> (w1261:cluster{i32, dbl, "AI data":dbl[][]})  [unwired: 1 in]
                        n537 = case shown="True" w1265 {
                          tunnel: w1246 -> [_ w1282]
                          tunnel: w1245 -> [_ w1281]
                          tunnel: w1266 -> [_ w1275]
                          tunnel: w1267 -> [_ w1276]
                          tunnel: w1254 -> [_ w1273]
                          tunnel: w1242 -> [w1268 w1274]
                          tunnel: [w1268 w1270] -> w1252
                          frame False {
                          }
                          frame True {
                            n538 = local read "laser bool array"() -> (w1283:bool[])
                            n539 = local read "full path"() -> (w1277:path)
                            n540 = call "subSaveAsBin_NW348.vi"("Delete .dcimg?"=TRUE, "Save Text file?"=FALSE, "Error in"=w1274, ".dcimg file name"=w1273) -> ("Error out"=w1270:errorcluster)  [unwired: 7 in]
                            n541 = Build Path(base path=w1277, name or relative path="Triwave_DAQ.txt") -> (appended path=w1280:path)
                            n542 = local write "Status"("Triangle wave: Saving binary file" ("Status")) -> ()
                            n543 = call "subSaveDaqDataAI_DI_NW348.vi"("DI waveform"=w1276, "AI data"=w1275, "Square or \nTriangle wave"=TRUE ("Square or \nTriangle wave"), "AO sq"=w1281, "Square\ndig. waveform"=w1282, "laser bool\n array"=w1283, "path"=w1280) -> ()  [unwired: 5 in]
                          }
                        }
                        n544 = local write "Waveform Graph"(w1261) -> ()
                        n545 = local write "Error"(w1252) -> ()
                      }
                    }
                  }
                  frame #4 {
                    n546 = Unbundle By Name(w1291) -> ("Laser pump"=w1290:bool)
                    n547 = case shown="True" w1290 {
                      tunnel: w1286 -> [_ w1313]
                      tunnel: w1288 -> [_ w1315]
                      tunnel: w1287 -> [_ w1314]
                      tunnel: w1289 -> [_ w1311]
                      tunnel: w1285 -> [_ w1294]
                      tunnel: w1284 -> [_ w1293]
                      frame False {
                      }
                      frame True {
                        w1298 = u16 1 items=["Amplitude", "Efficiency"] ("Input type")
                        w1303 = u16 0 items=["Amplitude", "Efficiency"] ("Input type")
                        # "Switch back to default setting"
                        # "For pumping measurement, \nswitch to constant laser power."
                        n548 = Bundle("DI camera fire"=w1311, w1315, "AO A-M External"=w1314, "AI ports"=w1313) -> (w1312:T38)  [unwired: 1 in]
                        n549 = local read "Error"() -> (w1300:errorcluster)
                        n550 = local read "Const power"() -> (w1301:u16[])
                        n551 = local read "AOTF info"() -> (w1302:T3)
                        n552 = local write "Status"("Laser Pump" ("Status")) -> ()
                        n553 = call "subAOTFamplitude_6channels_NW348.vi"("AOTF info"=w1302, "Input type"=w1303, "Error in"=w1300, "Amplitude In"=w1301) -> ("Error out"=w1299:errorcluster)  [unwired: 5 in, 2 out]
                        n554 = local read "DAQ sampling rate"() -> (w1310:dbl)
                        n555 = local read "Pump setting"() -> (w1308:T11)
                        n556 = local read "External"() -> (w1309:dbl)
                        n557 = call "subGenerateLaserPumpWaveform_NW348.vi"("num colors"=w1294, "Simultaneous"=w1293, "error in (no error)"=w1299, "Laser pump settings"=w1308, "External"=w1309, "A & D I/O\nsampling rate"=w1310) -> ("error out"=w1307:errorcluster, "AO waveform"=w1305:waveform(dbl), "DO waveform"=w1306:digitalwaveform[])  [unwired: 1 in, 2 out]
                        n558 = Reciprocal(x=w1310) -> (1/x=w1316:dbl)
                        n559 = call "subDataAcquisition_NW348.vi"("DAQ sampling rate"=w1310, "error in (no error)"=w1307, "DAQ ports"=w1312, "AO waveform"=w1305, "DO waveform"=w1306) -> ("error out"=w1296:errorcluster, "DI waveform"=w1321:digitalwaveform, "AI data"=w1320:dbl[][])  [unwired: 3 in, 1 out]
                        n560 = local read "SAVE"() -> (w1319:bool)
                        n561 = case shown="True" w1319 {
                          tunnel: w1306 -> [_ w1329]
                          tunnel: w1305 -> [_ w1328]
                          tunnel: w1320 -> [_ w1322]
                          tunnel: w1321 -> [_ w1323]
                          frame False {
                          }
                          frame True {
                            n562 = local read "laser bool array"() -> (w1330:bool[])
                            n563 = local read "full path"() -> (w1324:path)
                            n564 = Build Path(base path=w1324, name or relative path="Laser_pump_DAQ.txt") -> (appended path=w1327:path)
                            n565 = call "subSaveDaqDataAI_DI_NW348.vi"("DI waveform"=w1323, "AI data"=w1322, "Square or \nTriangle wave"=FALSE ("Square or \nTriangle wave"), "AO sq"=w1328, "Square\ndig. waveform"=w1329, "laser bool\n array"=w1330, "path"=w1327) -> ()  [unwired: 5 in]
                          }
                        }
                        n566 = local read "AOTF efficiency"() -> (w1297:dbl[])
                        n567 = Bundle(0, w1316, "AI data"=w1320) -> (w1318:cluster{i32, dbl, "AI data":dbl[][]})  [unwired: 1 in]
                        n568 = local read "AOTF info"() -> (w1292:T3)
                        n569 = local write "Waveform Graph"(w1318) -> ()
                        n570 = call "subAOTFamplitude_6channels_NW348.vi"("AOTF info"=w1292, "Input type"=w1298, "Error in"=w1296, "Efficiency In"=w1297) -> ("Error out"=w1295:errorcluster)  [unwired: 5 in, 2 out]
                        n571 = local write "Error"(w1295) -> ()
                      }
                    }
                  }
                  frame #5 {
                    n572 = Unbundle By Name(w1336) -> ("Memory"=w1335:bool)
                    n573 = case shown="False" w1335 {
                      tunnel: w1332 -> [_ w1352]
                      tunnel: w1333 -> [_ w1353]
                      tunnel: w1334 -> [_ w1350]
                      tunnel: w1331 -> [_ w1337]
                      frame False {
                      }
                      frame True {
                        n574 = Bundle("DI camera fire"=w1350, w1337, "AO A-M External"=w1353, "AI ports"=w1352) -> (w1351:T38)  [unwired: 1 in]
                        n575 = local read "full path"() -> (w1347:path)
                        n576 = local read "Error"() -> (w1338:errorcluster)
                        n577 = local read "Memory DO"() -> (w1340:digitalwaveform[])
                        n578 = local read "Memory AO"() -> (w1339:waveform(dbl))
                        n579 = local read "# cam. \nframes Mem"() -> (w1341:u32)
                        n580 = Build Path(base path=w1347, name or relative path="Mem_camera.dcimg") -> (appended path=w1345:path)
                        n581 = Reciprocal(x=5000.0 ("A & D I/O\nsampling rate")) -> (1/x=w1354:dbl)
                        n582 = local write "Status"("Memory: Acquiring .dcimg file" ("Status")) -> ()
                        n583 = call "subDataAcquisition_NW348.vi"("# cam.\nframes"=w1341, "DAQ sampling rate"=5000.0 ("A & D I/O\nsampling rate"), "Image file path"=w1345, "error in (no error)"=w1338, "DAQ ports"=w1351, "AO waveform"=w1339, "DO waveform"=w1340) -> ("error out"=w1348:errorcluster, "DI waveform"=w1359:digitalwaveform, "AI data"=w1358:dbl[][])  [unwired: 1 in, 1 out]
                        n584 = Bundle(0, w1354, "AI data"=w1358) -> (w1356:cluster{i32, dbl, "AI data":dbl[][]})  [unwired: 1 in]
                        n585 = local read "SAVE"() -> (w1357:bool)
                        n586 = local write "Waveform Graph"(w1356) -> ()
                        n587 = case shown="True" w1357 {
                          tunnel: w1340 -> [_ w1374]
                          tunnel: w1339 -> [_ w1373]
                          tunnel: w1358 -> [_ w1367]
                          tunnel: w1359 -> [_ w1368]
                          tunnel: w1345 -> [_ w1365]
                          tunnel: w1348 -> [w1360 w1366]
                          tunnel: [w1360 w1362] -> w1349
                          frame False {
                          }
                          frame True {
                            n588 = local read "laser bool array"() -> (w1375:bool[])
                            n589 = local read "full path"() -> (w1369:path)
                            n590 = call "subSaveAsBin_NW348.vi"("Delete .dcimg?"=TRUE, "Save Text file?"=FALSE, "Error in"=w1366, ".dcimg file name"=w1365) -> ("Error out"=w1362:errorcluster)  [unwired: 7 in]
                            n591 = Build Path(base path=w1369, name or relative path="Mem_DAQ.txt") -> (appended path=w1372:path)
                            n592 = local write "Status"("Memory: Saving binary file" ("Status")) -> ()
                            n593 = call "subSaveDaqDataAI_DI_NW348.vi"("DI waveform"=w1368, "AI data"=w1367, "Square or \nTriangle wave"=TRUE ("Square or \nTriangle wave"), "AO sq"=w1373, "Square\ndig. waveform"=w1374, "laser bool\n array"=w1375, "path"=w1372) -> ()  [unwired: 5 in]
                          }
                        }
                        n594 = local write "Error"(w1349) -> ()
                      }
                    }
                  }
                  frame #6 {
                    n595 = Unbundle By Name(w1381) -> ("Absolute Voltage"=w1380:bool)
                    n596 = case shown="True" w1380 {
                      tunnel: w1377 -> [_ w1397]
                      tunnel: w1378 -> [_ w1398]
                      tunnel: w1379 -> [_ w1395]
                      tunnel: w1376 -> [_ w1382]
                      frame False {
                      }
                      frame True {
                        n597 = Bundle("DI camera fire"=w1395, w1382, "AO A-M External"=w1398, "AI ports"=w1397) -> (w1396:T38)  [unwired: 1 in]
                        n598 = local read "full path"() -> (w1392:path)
                        n599 = local read "Error"() -> (w1384:errorcluster)
                        n600 = local read "Abs V DO"() -> (w1386:digitalwaveform[])
                        n601 = local read "Abs V AO"() -> (w1385:waveform(dbl))
                        n602 = local read "# cam. \nframes AbsV"() -> (w1387:u32)
                        n603 = Build Path(base path=w1392, name or relative path="AbsV_camera.dcimg") -> (appended path=w1390:path)
                        n604 = Reciprocal(x=5000.0 ("A & D I/O\nsampling rate")) -> (1/x=w1399:dbl)
                        n605 = local write "Status"("Absolute Voltage: Acquiring .dcimg file" ("Status")) -> ()
                        n606 = call "subDataAcquisition_NW348.vi"("# cam.\nframes"=w1387, "DAQ sampling rate"=5000.0 ("A & D I/O\nsampling rate"), "Image file path"=w1390, "error in (no error)"=w1384, "DAQ ports"=w1396, "AO waveform"=w1385, "DO waveform"=w1386) -> ("error out"=w1393:errorcluster, "DI waveform"=w1404:digitalwaveform, "AI data"=w1403:dbl[][])  [unwired: 1 in, 1 out]
                        n607 = local read "SAVE"() -> (w1402:bool)
                        n608 = Bundle(0, w1399, "AI data"=w1403) -> (w1401:cluster{i32, dbl, "AI data":dbl[][]})  [unwired: 1 in]
                        n609 = case shown="True" w1402 {
                          tunnel: w1386 -> [_ w1419]
                          tunnel: w1385 -> [_ w1418]
                          tunnel: w1403 -> [_ w1412]
                          tunnel: w1404 -> [_ w1413]
                          tunnel: w1390 -> [_ w1410]
                          tunnel: w1393 -> [w1405 w1411]
                          tunnel: [w1405 w1407] -> w1394
                          frame False {
                          }
                          frame True {
                            n610 = local read "laser bool array"() -> (w1420:bool[])
                            n611 = local read "full path"() -> (w1414:path)
                            n612 = call "subSaveAsBin_NW348.vi"("Delete .dcimg?"=TRUE, "Save Text file?"=FALSE, "Error in"=w1411, ".dcimg file name"=w1410) -> ("Error out"=w1407:errorcluster)  [unwired: 7 in]
                            n613 = Build Path(base path=w1414, name or relative path="AbsV_DAQ.txt") -> (appended path=w1417:path)
                            n614 = local write "Status"("Absolute Voltage: Saving binary file" ("Status")) -> ()
                            n615 = call "subSaveDaqDataAI_DI_NW348.vi"("DI waveform"=w1413, "AI data"=w1412, "Square or \nTriangle wave"=TRUE ("Square or \nTriangle wave"), "AO sq"=w1418, "Square\ndig. waveform"=w1419, "laser bool\n array"=w1420, "path"=w1417) -> ()  [unwired: 5 in]
                          }
                        }
                        n616 = local write "Waveform Graph"(w1401) -> ()
                        n617 = local write "Error"(w1394) -> ()
                      }
                    }
                  }
                  frame #7 {
                    w1431 = 7 items=["BINNING"=1, "BITS PER CHANNEL"=2, "ACTIVE VIEW INDEX"=3, "CCD MODE"=4, "SENSOR MODE"=5, "READOUT MODE"=6, "EXPOSURE TIME"=7, "CONTRAST GAIN"=8, "CONTRAST OFFSET"=9, "LIGHT MODE"=10, "SENSITIVITY"=11, "WHITE BALANCE"=12, "PHOTON IMAGING MODE"=13, "HIGH DYNAMIC RANGE MODE"=14, "TRIGGER SOURCE"=15, "TRIGGER ACTIVE"=16, "TRIGGER MODE"=17, "TRIGGER POLARITY"=18, "TRIGGER GLOBAL EXPOSURE"=19, "FIRST TRIGGER BEHAVIOR"=20, "TRIGGER TIMES"=21, "OUTPUT TRIGGER POLARITY"=22, "OUTPUT TRIGGER DELAY"=23, "OUTPUT TRIGGER PERIOD"=24, "TEMPERATURE"=25, "TEMPERATURE TARGET"=26, "SENSOR COOLER FAN"=27, "MECHANICAL SHUTTER"=28, "BACK FOCUS POSITION"=29, "FRAMEBUNDLE MODE"=30, "FRAMEBUNDLE NUMBER"=31, "LINEBUNDLE HEIGHT"=32, "TRIGGER CONNECTOR"=33, "IMAGE PIXEL TYPE"=34] ("Parameter")
                    w1436 = 1 items=["Internal"=1, "External"=2, "Software"=3] ("Trigger Source")
                    w1437 = 15 items=["BINNING"=1, "BITS PER CHANNEL"=2, "ACTIVE VIEW INDEX"=3, "CCD MODE"=4, "SENSOR MODE"=5, "READOUT MODE"=6, "EXPOSURE TIME"=7, "CONTRAST GAIN"=8, "CONTRAST OFFSET"=9, "LIGHT MODE"=10, "SENSITIVITY"=11, "WHITE BALANCE"=12, "PHOTON IMAGING MODE"=13, "HIGH DYNAMIC RANGE MODE"=14, "TRIGGER SOURCE"=15, "TRIGGER ACTIVE"=16, "TRIGGER MODE"=17, "TRIGGER POLARITY"=18, "TRIGGER GLOBAL EXPOSURE"=19, "FIRST TRIGGER BEHAVIOR"=20, "TRIGGER TIMES"=21, "OUTPUT TRIGGER POLARITY"=22, "OUTPUT TRIGGER DELAY"=23, "OUTPUT TRIGGER PERIOD"=24, "TEMPERATURE"=25, "TEMPERATURE TARGET"=26, "SENSOR COOLER FAN"=27, "MECHANICAL SHUTTER"=28, "BACK FOCUS POSITION"=29, "FRAMEBUNDLE MODE"=30, "FRAMEBUNDLE NUMBER"=31, "LINEBUNDLE HEIGHT"=32, "TRIGGER CONNECTOR"=33, "IMAGE PIXEL TYPE"=34] ("Parameter")
                    # "Default is Internal"
                    n618 = local read "Exposure (msec)"() -> (w1432:dbl)
                    n619 = local read "cam frame\nrate (Hz)"() -> (w1430:dbl[])
                    n620 = local read "Error"() -> (w1434:errorcluster)
                    n621 = local write "Start acquisition"(FALSE) -> ()
                    n622 = local read "Camera mode"() -> (w1433:u16)
                    n623 = local write "Status"("ready" ("Status")) -> ()
                    n624 = call <userlib>:"tm_setparameter.vi"("error in (no error)"=w1434, "Value in"=w1436, "Parameter"=w1437, "Handle in"=w1435) -> ("error out"=w1421:errorcluster, "Handle out"=w1424:u32)  [unwired: 6 in]
                    n625 = Reciprocal(x=w1430) -> (1/x=w1429:dbl[])
                    n626 = Divide(x=w1432, y=1000.0 ("milliseconds to wait")) -> (x/y=w1427:dbl)
                    n627 = Build Array (concatenate)(w1427, w1429) -> (w1426:dbl[])
                    n628 = Index Array(array=w1426, index=w1433) -> (element=w1425:dbl)
                    n629 = call <userlib>:"tm_setparameter.vi"("error in (no error)"=w1421, "Value in"=w1425, "Parameter"=w1431, "Handle in"=w1424) -> ("error out"=w1422:errorcluster, "Handle out"=w1423:u32)  [unwired: 6 in]
                    n630 = local read "Live"() -> (w1441:bool)
                    n631 = case shown="True" w1441 {
                      tunnel: w1423 -> [w1446 w1451]
                      tunnel: w1422 -> [w1445 w1450]
                      tunnel: [w1445 w1449] -> w1440
                      tunnel: [w1446 w1448] -> w1439
                      tunnel: [T16 {"width"=0, "height"=0, "datatype"=0} ("Buffer") w1447] -> w1438
                      frame False {
                      }
                      frame True {
                        w1452 = 1 items=["Snap", "Sequence"] ("Capture mode")
                        n632 = call <userlib>:"tm_preparecapture.vi"("error in (no error)"=w1450, "Capture mode"=w1452, "Handle in"=w1451) -> ("error out"=w1454:errorcluster, "Buffer"=w1447:T16, "Handle out"=w1453:u32)  [unwired: 5 in, 1 out]
                        n633 = call <userlib>:"tm_startcapture_b.vi"("error in (no error)"=w1454, "Handle in"=w1453) -> ("error out"=w1449:errorcluster, "Handle out"=w1448:u32)  [unwired: 8 in]
                      }
                    }
                  }
                }
              }
              frame True {
                n634 = local write "Start acquisition"(FALSE) -> ()
                n635 = One Button Dialog(message="Acquisition cancelled because camera frame rate is too fast.  \nReduce ROI or lower frame rate.") -> ()  [unwired: 1 in, 1 out]
              }
            }
          }
        }
        n636 = Wait (ms)(milliseconds to wait=u32 50) -> ()  [unwired: 1 out]
        n637 = local write "Error"(w425) -> ()
      }
      n638 = while {
        stop <- w155 stop-if-true
        # "Other Events"
        n639 = local read "Error"() -> (w154:errorcluster)
        n640 = event shown="[1] \"AOTF digital\", \"Shutters\": Value Change" {
          selector: _ -> [_ _ _ _ _ _ _ _ _ _ _ _]
          dyn-events: _ -> [_ _ _ _ _ _ _ _ _ _ _ _]
          timeout: 0 -> [_ _ _ _ _ _ _ _ _ _ _ _]
          tunnel: w154 -> [w157 w164 w168 w172 w179 w203 w219 w266 w301 w347 w366 w393]
          tunnel: [w157 w163 w167 w171 w178 w202 w218 w266 w295 w344 w365 w393] -> w153
          event Timeout {
            n641 = event-data() -> ()  [unwired: 1 in, 1 out]
          }
          event "AOTF\ndigital", "Shutters": Value Change {
            n642 = event-data() -> ()  [unwired: 1 in, 6 out]
            n643 = Cluster To Array(cluster="Shutter lines") -> (array=w166:tag[])
            n644 = call "subSetDigStates_NW348.vi"("Error in (no error)"=w164, "Digital line array"=w166, "Digital state array"="Shutters") -> ("Error out"=w165:errorcluster)  [unwired: 8 in]
            n645 = Cluster To Array(cluster="AOTF digital lines") -> (array=w162:tag[])
            n646 = call "subSetDigStates_NW348.vi"("Error in (no error)"=w165, "Digital line array"=w162, "Digital state array"="AOTF\ndigital") -> ("Error out"=w163:errorcluster)  [unwired: 8 in]
          }
          event "Emission filter": Value Change {
            n647 = event-data() -> ()  [unwired: 1 in, 1 out]
            n648 = call "subFilterWheelSet_NW348.vi"("Error in"=w168, "Filter Wheel Position - Control"="Emission filter") -> ("Error out"=w167:errorcluster)  [unwired: 9 in]
          }
          event "AOTF efficiency": Value Change {
            w176 = u16 1 items=["Amplitude", "Efficiency"] ("Input type")
            n649 = event-data() -> ()  [unwired: 1 in, 1 out]
            n650 = local read "AOTF amplitude"() -> (w173:u16[])
            n651 = local read "AOTF info"() -> (w177:T3)
            n652 = call "subAOTFamplitude_6channels_NW348.vi"("AOTF info"=w177, "Input type"=w176, "Error in"=w172, "Efficiency In"="AOTF efficiency", "Amplitude In"=w173) -> ("Error out"=w171:errorcluster, "Efficiency Out"=w174:dbl[], "Amplitude Out"=w175:u16[])  [unwired: 4 in]
            n653 = local write "AOTF amplitude"(w175) -> ()
            n654 = local write "AOTF efficiency"(w174) -> ()
          }
          event "apply const fluor", "apply const power", "apply dualview", "AOTF amplitude": Value Change {
            w183 = u16 0 items=["Amplitude", "Efficiency"] ("Input type")
            n655 = event-data() -> ()  [unwired: 1 in, 1 out]
            n656 = case shown="True" "apply const fluor" {
              tunnel: [w197 "Const fluor."] -> w185
              tunnel: "AOTF amplitude" -> [w197 _]
              frame False {
              }
              frame True {
                n657 = local write "apply const fluor"(FALSE ("apply const fluor")) -> ()
              }
            }
            n658 = case shown="True" "apply const power" {
              tunnel: w185 -> [w194 _]
              tunnel: [w194 "Const power"] -> w186
              frame False {
              }
              frame True {
                n659 = local write "apply const power"(FALSE ("apply const fluor")) -> ()
              }
            }
            n660 = case shown="True" "apply dualview" {
              tunnel: w186 -> [w191 _]
              tunnel: [w191 "DualView"] -> w180
              frame False {
              }
              frame True {
                n661 = local write "apply dualview"(FALSE ("apply const fluor")) -> ()
              }
            }
            n662 = call "subAOTFamplitude_6channels_NW348.vi"("AOTF info"="AOTF info", "Input type"=w183, "Error in"=w179, "Amplitude In"=w180) -> ("Error out"=w178:errorcluster, "Efficiency Out"=w182:dbl[], "Amplitude Out"=w181:u16[])  [unwired: 5 in]
            n663 = local write "AOTF efficiency"(w182) -> ()
            n664 = local write "AOTF amplitude"(w181) -> ()
          }
          event "447nm", "447 signal": Value Change {
            n665 = event-data() -> ()  [unwired: 1 in, 6 out]
            n666 = local read "AO ports"() -> (w201:T7)
            n667 = Unbundle By Name(w201) -> ("447nm laser"=w200:tag)
            n668 = call-poly <vilib>:"DAQmx Create Virtual Channel.vi"("maximum value"=5.0, "minimum value"=-5.0, "physical channels"=w200, "error in"=w203) -> ("task out"=w207:refnum<k21>, "error out"=w208:errorcluster)  [unwired: 5 in, 5 out]
            n669 = call <vilib>:"DAQmx Start Task.vi"("task/channels in"=w207, "error in"=w208) -> ("task out"=w206:refnum<k21>, "error out"=w205:errorcluster)  [unwired: 12 out]
            n670 = case shown="True" "447nm" {
              tunnel: [0.0 ("peak voltage") "447 signal"] -> w204
              frame False {
              }
              frame True {
              }
            }
            n671 = call-poly <vilib>:"DAQmx Write.vi"("task/channels in"=w206, "data"=w204, "error in"=w205) -> ("task out"=w212:refnum<k21>, "error out"=w211:errorcluster)  [unwired: 1 in, 10 out]
            n672 = call <vilib>:"DAQmx Clear Task.vi"("task in"=w212, "error in"=w211) -> ("error out"=w202:errorcluster)  [unwired: 13 out]
          }
          event "White LED", "White Light\nCurrent (mA)": Value Change {
            n673 = event-data() -> ()  [unwired: 1 in, 1 out]
            n674 = case shown="True" "White LED" {
              tunnel: [0.0 ("peak voltage") w233] -> w220
              tunnel: "White Light\nCurrent (mA)" -> [_ w232]
              frame False {
              }
              frame True {
                # "Thorlabs LED driver conversion factor (200 mA/V)."
                n675 = Divide(x=w232, y=200.0) -> (x/y=w234:dbl)
                n676 = Greater?(x=w234, y=3.5) -> (0:w236:bool)
                n677 = case shown="False" w236 {
                  tunnel: w234 -> [w238 _]
                  tunnel: [w238 1.0 ("peak voltage")] -> w233
                  frame False {
                  }
                  frame True {
                    n678 = call <vilib>:"Simple Error Handler.vi"("error source (\" \")"="Your peak voltage \nwas too high, \nso we used 1V = 200mA." ("error source (\" \")")) -> ()  [unwired: 4 in, 5 out]
                  }
                }
              }
            }
            n679 = Unbundle By Name("AO ports") -> ("White LED"=w216:tag)
            n680 = call-poly <vilib>:"DAQmx Create Virtual Channel.vi"("maximum value"=5.0, "minimum value"=-5.0, "physical channels"=w216, "error in"=w219) -> ("task out"=w223:refnum<k21>, "error out"=w224:errorcluster)  [unwired: 5 in, 5 out]
            n681 = call <vilib>:"DAQmx Start Task.vi"("task/channels in"=w223, "error in"=w224) -> ("task out"=w222:refnum<k21>, "error out"=w221:errorcluster)  [unwired: 12 out]
            n682 = call-poly <vilib>:"DAQmx Write.vi"("task/channels in"=w222, "data"=w220, "error in"=w221) -> ("task out"=w228:refnum<k21>, "error out"=w227:errorcluster)  [unwired: 1 in, 10 out]
            n683 = call <vilib>:"DAQmx Clear Task.vi"("task in"=w228, "error in"=w227) -> ("error out"=w218:errorcluster)  [unwired: 13 out]
          }
          event "Tab": Value Change {
            # "2 byte/pixel (16-bit)\n1024 bit/KB"
            n684 = event-data() -> ()  [unwired: 1 in, 1 out]
            n685 = local read "Triangle setting"() -> (w252:T9)
            n686 = local read "Square setting"() -> (w251:T8)
            n687 = local read "Triangle info"() -> (w263:T10)
            n688 = local read "Simultaneous"() -> (→"simultaneous ind":bool)
            n689 = local read "Square info"() -> (w262:cluster{"# frames":u32, "# output\nsamples":u32})
            n690 = local read "Lasers to use"() -> (→"laser bool array":bool[])
            n691 = Unbundle By Name(w251) -> ("Frame rate (Hz)"=w257:dbl)
            n692 = Unbundle By Name(w252) -> ("Frame rate (Hz)"=w258:dbl)
            n693 = Unbundle By Name(w262) -> ("# frames"=w264:u32)
            n694 = Unbundle By Name(w263) -> ("# frames"=w265:u32)
            n695 = local read "# cam\nframes"() -> (w261:i32[])
            n696 = local read "cam frame\nrate (Hz)"() -> (w255:dbl[])
            n697 = Build Array(w257, w258) -> (w253:dbl[])
            n698 = Build Array(w264, w265) -> (w259:u32[])
            n699 = Replace Array Subset(array=w261, new element=w259, index=0) -> (w245:i32[])
            "# cam\nframes" <- w245
            n700 = Replace Array Subset(array=w255, new element=w253, index=0) -> (→"cam frame\nrate (Hz)":dbl[])
            n701 = local read "ROI"() -> (w246:T1)
            n702 = Unbundle By Name(w246) -> ("x width"=w244:i32, "y width"=w243:i32)
            n703 = Multiply(x=w244, y=w243) -> (x*y=w242:i32)
            n704 = Multiply(x=w242, y=w245) -> (x*y=w249:i32[])
            n705 = Divide(x=w249, y=512000.0) -> (x/y=w247:dbl[])
            n706 = local write "file size (MB)"(w247) -> ()
          }
          event "Square setting", "Triangle setting", "Pump setting", "Lasers to use", "Simultaneous", "DAQ sampling rate", "External": Value Change {
            # "Generate 3 types of waveforms: \nvoltage square wave to test speed (for each color, multiple cycles through the spectrum)\nvoltage triangle wave to test sensitivity (dF/F) (for each color, multiple cycles through the spectrum)\nand lase modulation to test pumping (for each color, multiple cycles through the spectrum)"
            n707 = event-data() -> ()  [unwired: 1 in, 1 out]
            n708 = while {
              tunnel: [w341] -> w293
              tunnel: ["Lasers to use"] -> w269
              stop <- w342 stop-if-true
              n709 = Boolean To (0,1)(Boolean="Lasers to use") -> (0, 1=w343:i16[])
              n710 = Add Array Elements(numeric array=w343) -> (sum=w341:i16)
              n711 = Greater Than 0?(x=w341) -> (x > 0?=w342:bool)
            }
            n712 = local read "External"() -> (w297:dbl)
            n713 = call "subGenerateSquareWaveform_NW348.vi"("num colors"=w293, "Simultaneous"="Simultaneous", "error in (no error)"=w301, "Square wave settings"="Square setting", "External"=w297, "DAQ sampling rate"="DAQ sampling rate") -> ("error out"=w299:errorcluster, "Info"=→"Square info":T18, "Display Waveform"=→"Square Waveform":waveform(dbl)[])  [unwired: 3 out]
            n714 = Build Array(u32 16711680, u32 16744192, u32 14872320, u32 5621760, u32 54255) -> (w272:u32[])
            n715 = Build Array("Red laser", "Orange laser", "Yellow laser", "Green laser", "Blue laser") -> (w273:string[])
            n716 = for {
              shift-right: [w319] -> w271
              shift-left: 1 -> [w320]
              tunnel: w269 -> [w321] mode=indexing
              tunnel: w273 -> [w318] mode=indexing
              tunnel: w272 -> [w317] mode=indexing
              tunnel: TRUE ("Plot.Visible") -> [w316]
              n717 = case shown="True" w321 {
                tunnel: w320 -> [w322 w323]
                tunnel: [w322 w327] -> w319
                tunnel: w318 -> [_ w325]
                tunnel: w317 -> [_ w324]
                tunnel: w316 -> [_ w326]
                frame False {
                }
                frame True {
                  n718 = stacked-sequence {
                    tunnel: w326 -> [w328 w333 w338]
                    tunnel: w325 -> [w329 w332 w337]
                    tunnel: w324 -> [w331 w334 w339]
                    tunnel: w323 -> [w330 w335 w336]
                    frame #0 {
                      n719 = property on="Square Waveform" class="WFGraph (strict)"("Active Plot"=w330, "Plot.Plot Color"=w331, "Plot.Visible?"=w328, "Plot.Plot Name"=w329) -> ()  [unwired: 2 in, 2 out]
                    }
                    frame #1 {
                      n720 = property on="Triangle Waveform" class="WFGraph (strict)"("Active Plot"=w335, "Plot.Plot Color"=w334, "Plot.Visible?"=w333, "Plot.Plot Name"=w332) -> ()  [unwired: 2 in, 2 out]
                    }
                    frame #2 {
                      n721 = property on="Laser Pump Waveform" class="WFGraph (strict)"("Active Plot"=w336, "Plot.Plot Color"=w339, "Plot.Visible?"=w338, "Plot.Plot Name"=w337) -> ()  [unwired: 2 in, 2 out]
                    }
                  }
                  n722 = Increment(x=w323) -> (x+1=w327:i32)
                }
              }
            }
            n723 = call "subGenerateTriangleWaveform_NW348.vi"("num colors"=w293, "Simultaneous"="Simultaneous", "error in (no error)"=w299, "Triangle wave settings"="Triangle setting", "External"=w297, "DAQ sampling rate"="DAQ sampling rate") -> ("error out"=w296:errorcluster, "Triangle info"=→"Triangle info":T20, "Triangle Waveform"=→"Triangle Waveform":waveform(dbl)[])  [unwired: 3 out]
            n724 = Subtract(x=6, y=w271) -> (x-y=w268:i32)
            n725 = for {
              N: w268 -> [_]
              tunnel: w271 -> [w303]
              i -> [w302]
              n726 = Add(x=w303, y=w302) -> (x+y=w306:i32)
              n727 = stacked-sequence {
                tunnel: w306 -> [w309 w312 w313]
                tunnel: "" ("Plot.Plot Name") -> [w308 w310 w314]
                tunnel: FALSE ("Plot.Visible") -> [w307 w311 w315]
                frame #0 {
                  n728 = property on="Square Waveform" class="WFGraph (strict)"("Active Plot"=w309, "Plot.Visible?"=w307, "Plot.Plot Name"=w308) -> ()  [unwired: 2 in, 2 out]
                }
                frame #1 {
                  n729 = property on="Triangle Waveform" class="WFGraph (strict)"("Active Plot"=w312, "Plot.Visible?"=w311, "Plot.Plot Name"=w310) -> ()  [unwired: 2 in, 2 out]
                }
                frame #2 {
                  n730 = property on="Laser Pump Waveform" class="WFGraph (strict)"("Active Plot"=w313, "Plot.Visible?"=w315, "Plot.Plot Name"=w314) -> ()  [unwired: 2 in, 2 out]
                }
              }
            }
            n731 = call "subGenerateLaserPumpWaveform_NW348.vi"("num colors"=w293, "Simultaneous"="Simultaneous", "error in (no error)"=w296, "Laser pump settings"="Pump setting", "A & D I/O\nsampling rate"="DAQ sampling rate") -> ("error out"=w295:errorcluster, "num. output\nsamples L"=→"# output\nsamples L":u32, "Display Waveform"=→"Laser Pump Waveform":waveform(dbl)[])  [unwired: 2 in, 2 out]
          }
          event "Test patch": Value Change {
            # "mV/nA --> V/pA"
            n732 = event-data() -> ()  [unwired: 1 in, 1 out]
            n733 = case shown="False" "Probe Gain" {
              tunnel: [100 10000] -> w355
              frame False {
                # "Low: 100mV/nA"
              }
              frame True {
                # "High: 10000 mV/nA"
              }
            }
            n734 = Compound Arithmetic op=MULTIPLY(w355, "Gain", 1e-06 ("value")) -> (w352:dbl)
            n735 = local read "AO ports"() -> (w349:T7)
            n736 = local read "AI ports"() -> (w348:T6)
            n737 = Reciprocal(x=w352) -> (1/x=w351:dbl)
            n738 = Bundle(w351, "External"="External") -> (w346:cluster{dbl, "External":dbl})  [unwired: 1 in]
            n739 = call "subPipetteTuning_NW348.vi"("A-M param"=w346, "Error in (no error)"=w347, "AI ports"=w348, "AO ports"=w349, "Pipet tuning param"="Patch tuning param") -> ("Error out"=w345:errorcluster, "Average I-t curve"=→"Average I-t curve":cluster{"xo":i32, dbl, dbl[]}, "Scaled output"=→"Scaled output":cluster{"xo":i32, dbl, "data":dbl[][]}, "Patch quality"=→"Patch quality":T14)  [unwired: 3 in]
            n740 = flat-sequence {
              tunnel: w345 -> [w362]
              tunnel: [w362] -> w344
              frame #0 {
                n741 = local write "Test patch"(FALSE ("Test patch")) -> ()
              }
            }
          }
          event "Save patch param": Value Change {
            n742 = event-data() -> ()  [unwired: 1 in, 1 out]
            n743 = local read "Patch quality"() -> (w372:T14)
            n744 = local read "base path"() -> (w367:path)
            n745 = call "File Dialog - Save patch"("start path"=w367, "prompt"="Choose path and file name.", "button label"="SAVE", "default name"="patch param" ("button label"), "error in"=w366, "pattern (all files)"="*.txt" ("default name"), "pattern label"="Text file" ("default name")) -> ("selected path"=w376:path, "cancelled"=w374:bool, "error out"=w378:errorcluster)  [unwired: 5 in, 1 out]
            n746 = Number To Decimal String(number=w372) -> (decimal integer string=w375:T39)  [unwired: 1 in]
            n747 = case shown="False" w374 {
              tunnel: w375 -> [w381 _]
              tunnel: w376 -> [w380 _]
              tunnel: w378 -> [w379 _]
              tunnel: [w379 errorcluster {"status"=FALSE, "code"=0, "source"=""} ("camera \ninitialization\nerror")] -> w365
              frame False {
                w387 = " Mohm"
                w386 = "\r"
                n748 = Unbundle By Name(w381) -> ("Ra (Mohm)"=w389:string, "Rm (Mohm)"=w388:string, "Cm (pF)"=w384:string)
                n749 = Concatenate Strings("Ra = ", w389, w387, w386, "Rm = ", w388, w387, w386, "Cm = ", w384, " pF", w386) -> (w382:string)
                n750 = Write to Text File(file (use dialog)=w380, text=w382) -> ()  [unwired: 2 in, 3 out]
              }
              frame True {
              }
            }
            n751 = local write "Save patch param"(FALSE ("Save patch param")) -> ()
          }
          event "Load Mem_AbsV waveform": Value Change {
            n752 = event-data() -> ()  [unwired: 1 in, 1 out]
            n753 = stacked-sequence {
              frame #0 {
                # "camera duty cycle (%)"
                # "sampling rate"
                # "Load memory waveform into memory"
                n754 = call "Load_waveforms_subvi.vi"("Camera trigger duty cycle (%)"=20.0, "Camera frame rate (Hz)"="Cam frame rate (Hz)\nMem", "waveform txt file"="Memory Waveform txt file", "Sampling rate (Hz)"=5000.0) -> ("memory camera"=→"memory camera":digitalwaveform, "Memory dig waveform"=→"Memory DO":digitalwaveform[], "Memory lasers"=→"Memory lasers":digitalwaveform[], "Total time"=→"Tot time \nMem (s)":dbl, "Memory AO"=→"Memory AO":waveform(dbl), "Number of Camera Frames"=→"# cam. \nframes Mem":i32, "laser boolean array"=→"laser boolean array memory":bool[], "sample num"=→"Sample num mem":i32)
              }
              frame #1 {
                # "camera duty cycle (%)"
                # "sampling rate"
                # "Load abs V waveform into memory"
                n755 = call "Load_waveforms_subvi.vi"("Camera trigger duty cycle (%)"=20.0, "Camera frame rate (Hz)"="Cam frame rate (Hz)\nAbs V", "waveform txt file"="Abs V Waveform txt file", "Sampling rate (Hz)"=5000.0) -> ("memory camera"=→"Abs V camera":digitalwaveform, "Memory dig waveform"=→"Abs V DO":digitalwaveform[], "Memory lasers"=→"Abs V lasers":digitalwaveform[], "Total time"=→"Tot time \nAbs V (s)":dbl, "Memory AO"=→"Abs V AO":waveform(dbl), "Number of Camera Frames"=→"# cam. \nframes AbsV":i32, "laser boolean array"=→"laser boolean array abs V":bool[], "sample num"=→"sample num AbsV":i32)
              }
              frame #2 {
                n756 = local write "Load Mem_AbsV waveform"(FALSE ("Load Mem_AbsV waveform")) -> ()
                "Waveform generated" <- TRUE ("Waveform generated")
              }
            }
          }
        }
        n757 = Wait (ms)(milliseconds to wait=u32 50) -> ()  [unwired: 1 out]
        n758 = local read "stop program"() -> (w155:bool)
        n759 = local write "Error"(w153) -> ()
      }
    }
    frame #2 {
      w1460 = 0 ("Initialize")
      w1461 = "-" ("Camera ID")
      # "Close camera and deinitialize"
      n760 = local read "Error"() -> (w1463:errorcluster)
      n761 = call <userlib>:"tm_closecamera.vi"("error in (no error)"=w1463, "Handle in"=u32 0) -> ("error out"=w1465:errorcluster)  [unwired: 9 in]
      n762 = local write "stop program"(FALSE ("stop program")) -> ()
      n763 = local write "Initialize?"(FALSE ("stop program")) -> ()
      n764 = call <userlib>:"tm_deinitialize.vi"("error in (no error)"=w1465) -> ("error out"=w1466:errorcluster)  [unwired: 10 in]
      n765 = local write "Error"(w1466) -> ()
      n766 = local write "Bits per Channel"(w1460) -> ()
      n767 = local write "x pixels"(w1460) -> ()
      n768 = local write "y pixels"(w1460) -> ()
      n769 = local write "Camera ID"(w1461) -> ()
      n770 = local write "Model"(w1461) -> ()
    }
  }
